vi "Vision_MainUI.vi"(5 "Seq Edit":T2, 7 "Vision Station On?":bool, 8 "error constant":errorcluster, 9 "Real Position Info":T1) -> (0 "error out":errorcluster)   [LabVIEW 2019]
doc: "20160716\nAdd VersionCheck\n\n20160614\nModify Analysis VI : Disable \"Inistialize\" When run it\nModify dll VI : ForCalCalculation memory allocation"
uses:
  Analysis/Controls/Analysis_Type.ctl
  <vilib>/vision/Image Controls.llb/IMAQ Image.ctl
  Controls/UI_Action.ctl
  ROI/Controls/ROI_List_Action.ctl
  Analysis/Controls/Analysis_Setting.ctl
  Process/Controls/Process_Setting.ctl
  Controls/Vision_DataEntry.ctl
  Caliper/Controls/Caliper_Entry_FGV_Action.ctl
  Caliper/Controls/CaliperResult.ctl
  Caliper/Controls/SelectionListEntryPointType.ctl
  Caliper/Controls/SelectionListEntry.ctl
  Caliper/Controls/CaliperType.ctl
  Caliper/Controls/CaliperDataEntry.ctl
  Coordinate/Control/CoordinateAction.ctl
  Coordinate/Control/CoordinateAnalysisSetting.ctl
  Coordinate/Control/CoordinatteEntry.ctl
  Caliper/Controls/AnalysisResultPointsAction.ctl
  Analysis/Controls/Analysis_Result_To_Caliper.ctl
  Controls/Parameter.ctl
  Controls/ParameterData.ctl
  <vilib>/vision/NI_Vision_Development_Module.lvlib
  SubVIs/[Global]iVision_Version.vi
  Controls/iVisionSEQ.ctl
  Coordinate/Control/CoordinateCaliperSetting.ctl
  Analysis/SubVI/[Global]VisionAnalysis_DVR.vi
  Analysis/VisionAnalysisFramework/PackedLibrary/VisionAnalysisFramework.lvlibp/VisionAnalysisFramework/Object/VisionAnalysisFramework.lvclass
  <vilib>/Utility/miscctls.llb/LVRowAndColumnUnsignedTypeDef.ctl
  Analysis/Controls/V_Analysis_Type.ctl
  Ctrl/VisionProcessName.ctl
panel:
  out "Boolean":bool
  in  "CameraName 2":u16(ring) items=["cam0"]
  out "ProjectNameOut":string
  out "Cal Info Image":T3
  in  "Calib":bool
  in  "ConfigROI":bool
  out "RootPath":path
  out "Folder Image Files":path[](array[path])
  in  "SEQ_Name":u16(ring) caption="SEQ Name" items=["v1"]
  in  "Main_Tab":enum32{"Setting", "Result"}(tab)
  in  "Rotate Image Angle":bool
  in  "Angle":dbl format="%#_6f"
  in  "Calibration On":bool
  out "Image Calibration":bool
  in  "Coordinate On":bool
  out "Coordinate Status":bool
  in  "File Path":path
  in  "CycleThruFolder":bool
  in  "GetImage":bool
  in  "SingleRun":bool
  in  "Snap":bool
  in  "ContRun":bool
  out "Vision_Image":T3(plugin-control)
  in  "ROI List":i32[](listbox)
  in  "DeleteROI":bool
  in  "Function_Tab":enum32{"Process", "Analysis", "Caliper"}(tab)
  out "Process Steps":i32(listbox)
  in  "ConfigProcess":bool
  in  "Analysis Function":T4 items=["None", "PatternMatch", "Edge Detection", "Barcode 1D", "Barcode 2D", "Clamp", "Clamp MAX", "Particle", "Histogram", "Straight Edge", "Circle", "Shape Detect", "OCR", "Contour", "ColorMatch"]
  in  "ConfigAnalysis":bool
  in  "CaliperList":i32[](listbox)
  in  "ConfigureCaliper":bool
  in  "RemoveROI":bool
  in  "CreateROI":bool
  in  "CameraName":u16(ring) items=["cam0"]
  in  "Auto Loading ROI Setting":bool
  in  "RemoveFromList":bool caption="Remove"
  in  "AddToOutput":bool caption="Add"
  in  "Output List":i32[](listbox)
  in  "Analysis Result":i32[](listbox)
  out "Item Names":string[][](array[string])
  in  "ExitVisionEditor":bool caption="Exit"
  in  "SaveVisionSEQ":bool caption="Save"
  in  "DeleteVisionSEQ":bool caption="Delete"
  in  "Vision_SEQ_Name":enum16{""}(ring)
  in  "NewVisionSEQ":bool caption="New"
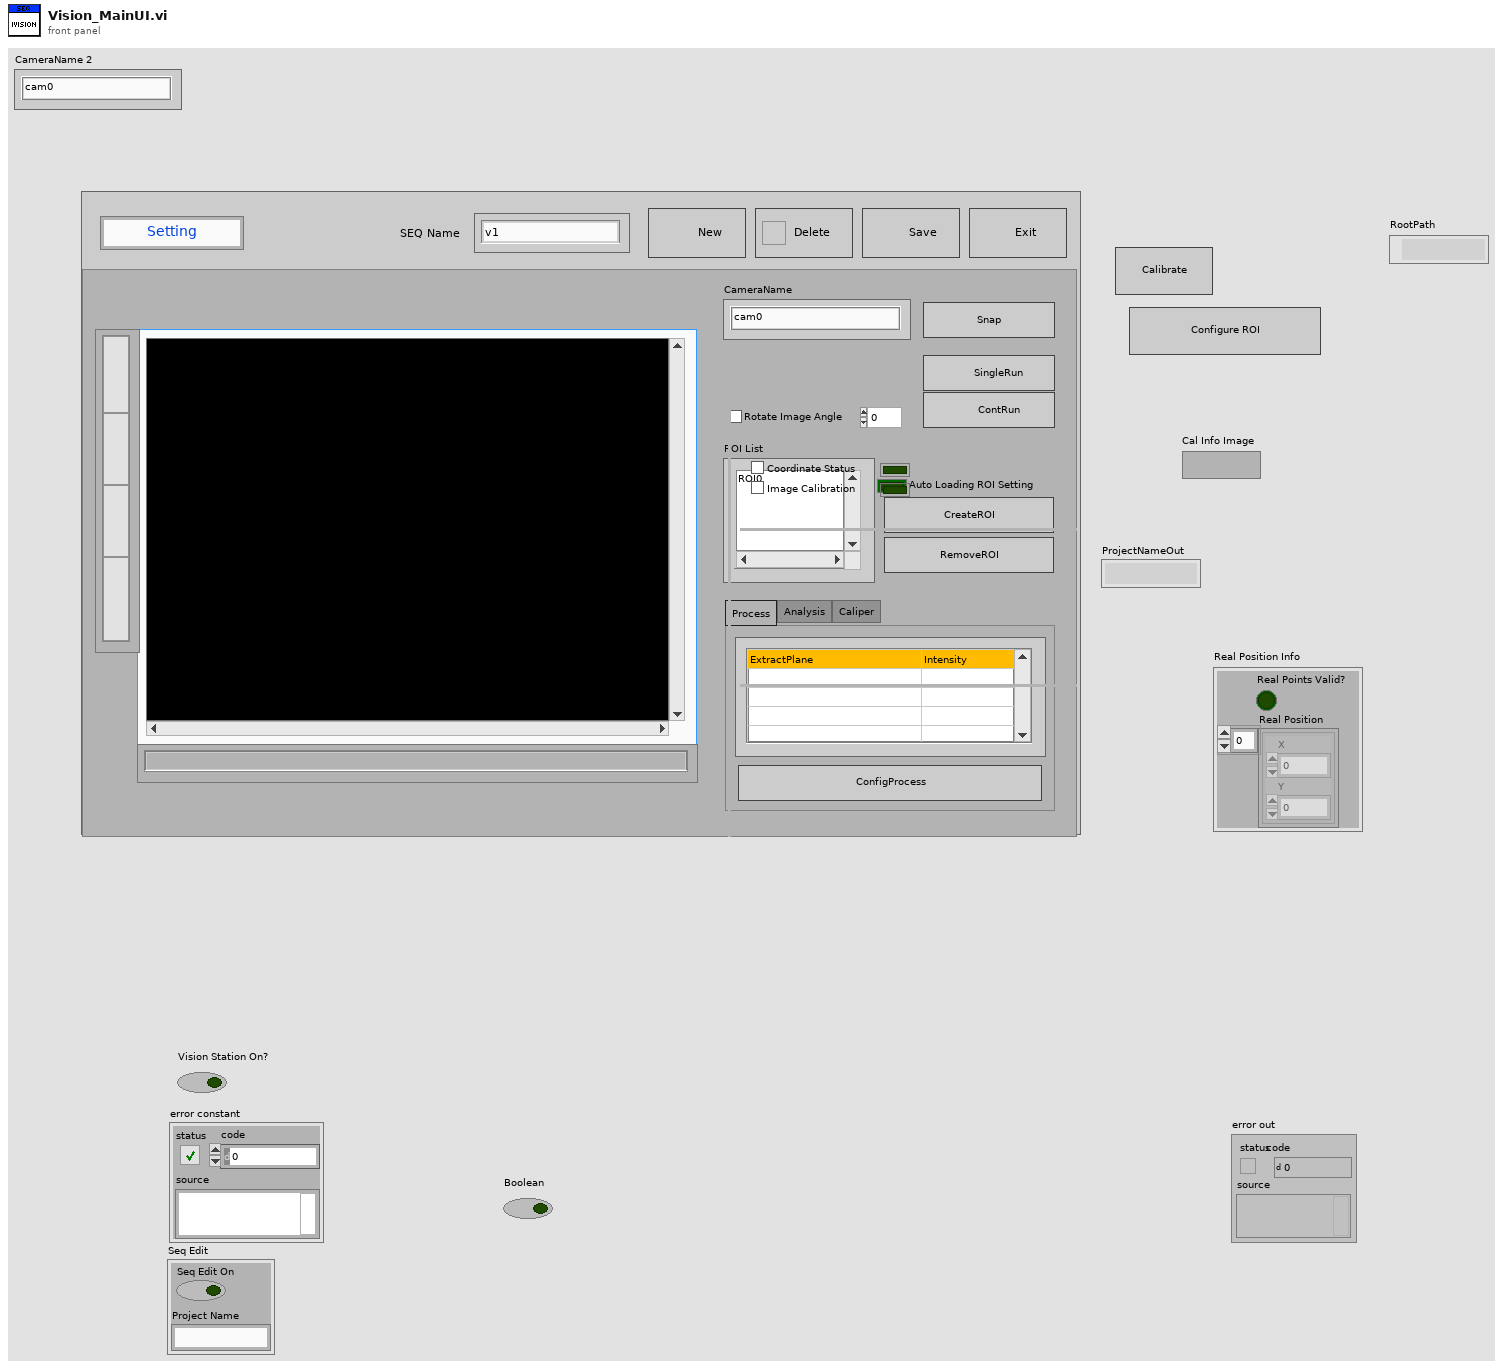
[diagram p1: front panel]
types:
  T1 = cluster{"Real Points Valid?":bool, "Real Position":cluster{"X":dbl, "Y":dbl}[]}
  T2 = cluster{"Seq Edit On":bool, "Project Name":string}
  T3 = typedef "IMAQ Image.ctl" = refnum<image>
  T4 = typedef "Analysis_Type.ctl" = u16
  T5 = typedef "UI_Action.ctl" = enum16{"Init Setting", "Get Root Path", "Exit", "ActivateAllControls", "UpdateROIListbox", "UpdateSelectROIOverlay", "UpdateUIOverlay", "UpdateSelectedOverlay", "ConfigAnalysis", "ConfigProcess", "UpdateExistProjNames", "Init Result Page", "UpdateResultTable", "Init Menu", "Activate Menu", "UpdateProcess", "UpdateAnalysis", "SingleRun", "UpdateSelecedOutput", "ReloadResultTable", "SingleRunWithoutCaliper", "AddNewSeq", "UpdateCaliper", "SaveVisionSEQ", "Init User Parameter", "Cont.Run", "CalRotateImage", "Idle", "UpdateInitStatus", "Initilaize Camera", "Init Read Template", ""}
  T6 = typedef "AnalysisResultPointsAction.ctl" = enum16{"Init", "Add", "Delete", "ReplaceAll", "ReadAll", "Close"}
  T7 = typedef "Caliper_Entry_FGV_Action.ctl" = enum16{"Init", "Close", "Add", "Delete", "ReplaceAll", "ReadAll"}
  T8 = enum8{"Enabled", "Disabled", "Disabled and Grayed Out"}
  T9 = enum16{"Init", "Add", "Remove", "Read All", "Remove All"}
  T10 = typedef "ROI_List_Action.ctl" = enum16{"Init", "Add ROI", "Delete ROI", "Get All ROI", "Get Specific ROI", "Set Analysis Setting", "Set Process Setting", "Replace All Entries", "ROIEntryBackup", "ROIEntryBackupClear", "ROIEntryReturn"}
  T11 = typedef "CoordinateAction.ctl" = enum16{"Initialize", "CoordEntryInput", "CoordEntryOutput", "CoordEntryTemp", "CoordEntryBackup", "CoordEntryReturn"}
  T12 = typedef "Parameter.ctl" = enum16{"Initialize", "Write", "Read", "WriteAll", "Save", "Load"}
  T13 = enum16{"Init", "Grab", "Get All", "Close", "Set Camera"}
  T14 = enum16{"None", "Pattern Match", "Edge Detection", "Barcode 1D", "Barcode 2D", "Clamp", "Clamp MAX", "Particle", "Histogram", "Straight Edge", "Circle", "Shape Dectect", "OCR"}
  T15 = typedef "Analysis_Result_To_Caliper.ctl" = cluster{"PointName":string, "Position_X":dbl, "Position_Y":dbl}
  T16 = enum16{"Init", "Add", "Remove", "Read All", "Remove All", "WriteCriteria"}
  T17 = typedef "CoordinatteEntry.ctl" = cluster{"ProcessSetting":T18[], "Project Name":string, "AnalysisSetting":T20[], "Coord?":bool, "OriginPointInfo":cluster{"Output Original":bool, "Origin Name":string, "Angle":dbl, "Mode":u16, "OriginPoint":cluster{"X":dbl, "Y":dbl}}, "CaliperSetting":T22[], "CoordIndex":i32[]}
  T18 = typedef "Process_Setting.ctl" = cluster{"Enum_PreProcess":T19, "Parameter":string}
  T19 = typedef "VisionProcessName.ctl" = enum16{"*CamParameter*", "CamAttributes", "*Preprocess*", "CG_Brightness", "C_Plane Extraction", "C_Threshold", "G_Lookup Table", "G_Threshold"}
  T20 = typedef "CoordinateAnalysisSetting.ctl" = cluster{"Analysis_Type":enum16{"PatternMatch", "Straight Edge"}, "ROI ":T21, "Parameter":variant, "Step Result":variant, "AnalysisStepName":string, "CoordinateUse":bool}
  T21 = typedef "ROI Descriptor" = cluster{"Global Rectangle":i32[], "Contours":cluster{"ID":enum32{"External", "Internal"}, "Type":u32, "Coordinates":i32[]}[]}
  T22 = typedef "CoordinateCaliperSetting.ctl" = cluster{"Result":variant, "CoordinateUse":bool, "CaliperEntry":T23}
  T23 = typedef "CaliperDataEntry.ctl" = cluster{"CaliperType":T24, "Points":T25[], "Result":T27, "StepName":string}
  T24 = typedef "CaliperType.ctl" = u32
  T25 = typedef "SelectionListEntry.ctl" = cluster{"Type":T26, "Index":i32}
  T26 = typedef "SelectionListEntryPointType.ctl" = enum16{"AnalysisResult", "CaliperResult"}
  T27 = typedef "CaliperResult.ctl" = cluster{"PointInclude?":bool, "Num_Of_Pts":u8, "Position.X":dbl, "Position.Y":dbl, "Angle":dbl, "Distance":dbl, "Area":dbl, "Radius_MAX":dbl, "Radius2_min":dbl, "Dev_Residual":dbl, "P2.X":dbl, "P2.Y":dbl, "StepName":string, "Point ID":u8, "StepError?":bool, "ResultDiff?":bool}
  T28 = typedef "ParameterData.ctl" = cluster{"Rotate Angle":dbl, "Rotate?":bool, "Calibration File Path":string, "Cal?":bool}
  T29 = typedef "Vision_DataEntry.ctl" = cluster{"vROIName":string, "vROIContour":cluster{"Contour Type":u32, "ROI Type":u32, "Points":i32[]}, "ProcessSetting":T18[], "Analysis_Setting":T30}
  T30 = typedef "Analysis_Setting.ctl" = cluster{"PreProcess":T31, "Parameter":string}
  T31 = typedef "V_Analysis_Type.ctl" = enum16{"None", "C_Color Pattern Matching", "G_PatternMatching", "G_ShapeDectect", "G_GeometricMatch", "B_Area Check"}
  T32 = typedef "Image Type" = u32
  T33 = enum32{"invalid app kind", "Development System", "Run Time System", "Student Edition", "Embedded LabVIEW", "Evaluation", "Custom"}
  T34 = typedef "Vision_DataEntry.ctl" = cluster{"vROIName":string, "vROIContour":cluster{"Contour Type":u32, "ROI Type":u32, "Points":i32[]}, "ProcessSetting":T18[], "Analysis_Setting":T35}
  T35 = typedef "Analysis_Setting.ctl" = cluster{"PreProcess":T36, "Parameter":string}
  T36 = typedef "VisionProcessName.ctl" = enum16{"*CamParameter*", "CamAttributes", "*Preprocess*", "CG_Brightness", "C_Plane Extraction", "C_Threshold", "G_Lookup Table", "G_Threshold", "B_Image Inversion", "*Algorithm*", "CG_Histogram", "C_Color Matching", "C_Color Pattern Matching", "G_PatternMatch", "CG_Find Straight Edge", "CG_Adv. Find Straight Edge", "CG_Find Circular Edge", "G_Max Clamp", "G_Clamp (Rake)", "G_Pattern Matching"}
  T37 = typedef "IMAQ Coordinate System" = cluster{"Reference System":cluster{"Origin":cluster{"X":sgl, "Y":sgl}, "Angle (deg)":sgl, "Axis Reference":u32}, "Measurement System":cluster{"Origin":cluster{"X":sgl, "Y":sgl}, "Angle (deg)":sgl, "Axis Reference":u32}}
  T38 = typedef "Analysis_Setting.ctl" = cluster{"PreProcess":T39, "Parameter":string}
  T39 = typedef "V_Analysis_Type.ctl" = enum16{"None", "C_Color Pattern Matching", "G_PatternMatching"}
  T40 = typedef "LVMenuShortCut.ctl" = cluster{"include Shift key?":bool, "include Ctrl key?":bool, "shortcut key":string}
  T41 = cluster{"OutputList":u16[], "Criteria Condition":string[]}
  T42 = typedef "iVisionSEQ.ctl" = cluster{"iVision_Version":string, "iVisionSEQParam":variant}
  T43 = enum16{"open", "replace", "create", "open or create", "replace or create", "replace or create with confirmation"}
  T44 = cluster{"All ROI":cluster{"vROIName":string, "vROIContour":cluster{"Contour Type":u32, "ROI Type":u32, "Points":i32[]}, "ProcessSetting":cluster{"Process_Type":enum16{"None", "ExtractPlane", "BinaryMono", "Operators", "GrayMorphology", "Filters", "Lookup Table", "Particle Filter", "Mask"}, "Parameter":variant}[], "Analysis_Setting":cluster{"Analysis_Type":enum16{"None", "PatternMatch", "Edge Detection", "Barcode 1D", "Barcode 2D", "Clamp", "Clamp MAX", "Particle", "Histogram", "Straight Edge", "Circle", "Shape Dectect", "OCR"}, "RegionContour":cluster{"Contour Type":u32, "ROI Type":u32, "Points":i32[]}, "Parameter":variant}}[], "Output":cluster{"OutputList":u16[], "Criteria Condition":string[]}, string[][], "AllCaliperEntries":cluster{"CaliperType":u32, "Points":cluster{"Type":enum16{"AnalysisResult", "CaliperResult"}, "Index":i32}[], "Result":cluster{"PointInclude?":bool, "Num_Of_Pts":u8, "Position.X":dbl, "Position.Y":dbl, "Angle":dbl, "Distance":dbl, "Area":dbl, "Radius_MAX":dbl, "Radius2_min":dbl, "Dev_Residual":dbl, "P2.X":dbl, "P2.Y":dbl, "StepName":string, "Point ID":u8, "StepError?":bool, "ResultDiff?":bool}, "StepName":string}[], "CoordinatteEntry Output":cluster{"ProcessSetting":cluster{"Process_Type":enum16{"None", "ExtractPlane", "BinaryMono", "Operators", "GrayMorphology", "Filters", "Lookup Table", "Particle Filter", "Mask"}, "Parameter":variant}[], "Project Name":string, "AnalysisSetting":cluster{"Analysis_Type":enum16{"PatternMatch", "Straight Edge"}, "ROI ":T21, "Parameter":variant, "Step Result":variant, "OriginPointInfo":cluster{"Output Original":bool, "Origin Name":string, "Angle":dbl, "Mode":u16, "OriginPoint":cluster{"X":dbl, "Y":dbl}}, "AnalysisStepName":string}[], "Coord?":bool}, "ParameterData Out":cluster{"Rotate Angle":dbl, "Rotate?":bool, "Calibration File Path":string, "Cal?":bool}, "AllCaliperEntries":cluster{"CaliperType":u32, "Points":cluster{"Type":enum16{"AnalysisResult", "CaliperResult"}, "Index":i32}[], "Result":cluster{"PointInclude?":bool, "Num_Of_Pts":u8, "Position.X":dbl, "Position.Y":dbl, "Angle":dbl, "Distance":dbl, "Area":dbl, "Radius_MAX":dbl, "Radius2_min":dbl, "Dev_Residual":dbl, "P2.X":dbl, "P2.Y":dbl, "StepName":string, "Point ID":u8, "StepError?":bool, "ResultDiff?":bool}, "StepName":string}[]}
  T45 = cluster{"All ROI":T29[], "Output":cluster{"OutputList":u16[], "Criteria Condition":string[]}, string[][], "AllCaliperEntries":T23[], "CoordinatteEntry Output":T17, "ParameterData Out":T28, "AllCaliperEntries":T23[]}
  T46 = typedef "LVRowAndColumnUnsignedTypeDef.ctl" = cluster{"Row":u32, "Column":u32}
  T47 = typedef "IMAQdx.ctl" = refnum<k21>
  T48 = cluster{"Global Rectangle":i32[], "Contours":cluster{"Contour Type":u32, "ROI Type":u32, "Points":i32[]}[]}
  T49 = cluster{"Contour Type":u32, "ROI Type":u32, "Points":i32[]}[]
  T50 = cluster{"Contour Type":u32, "ROI Type":u32, "Points":i32[]}
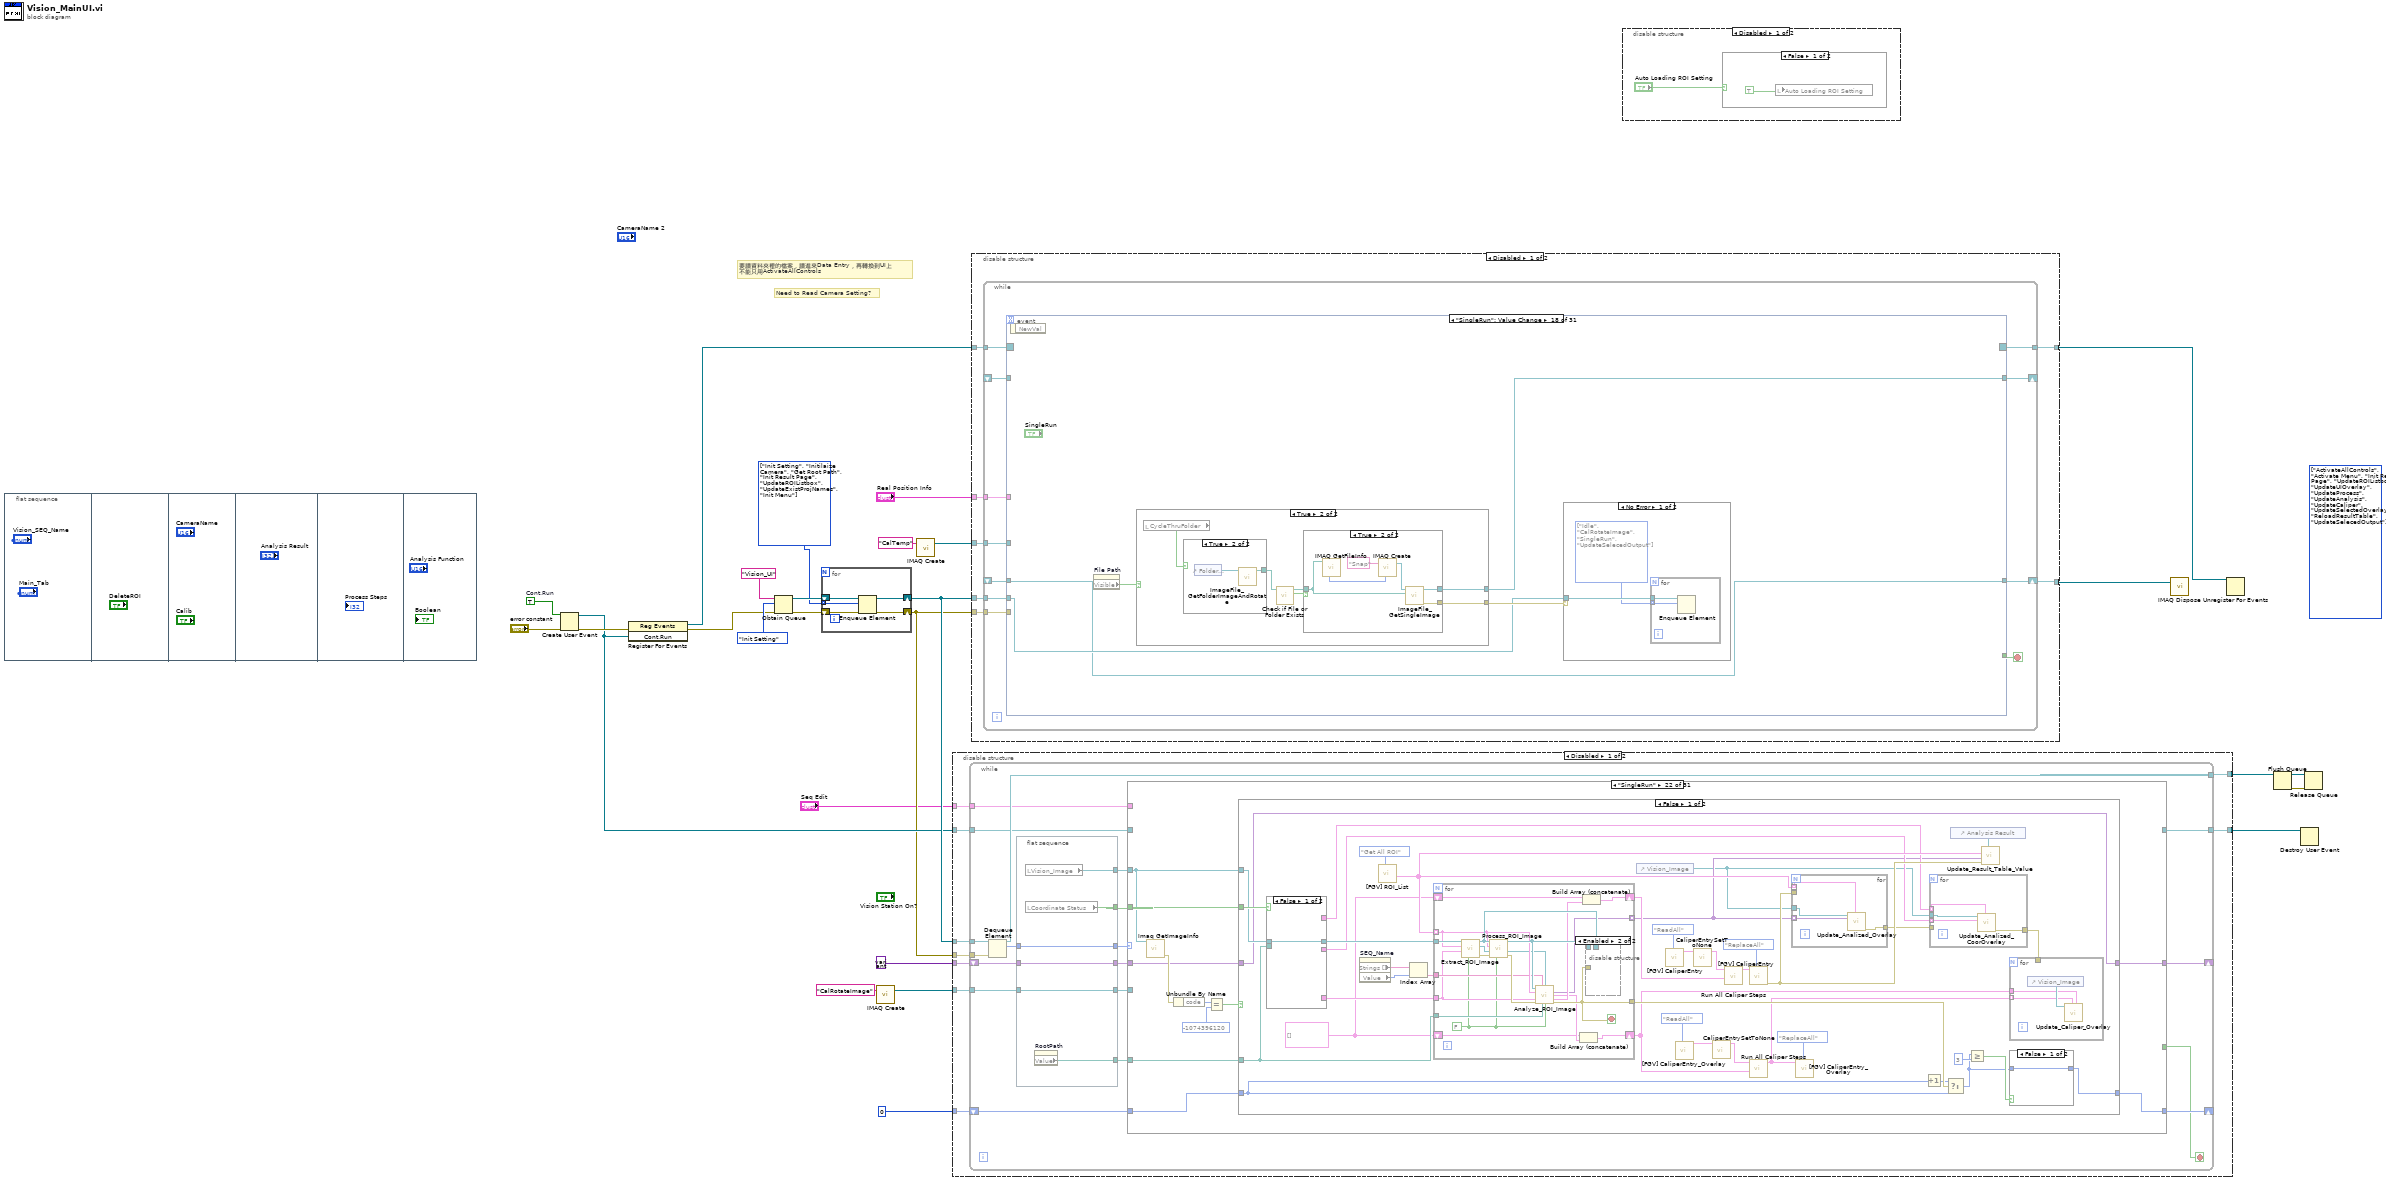
[diagram p0: block diagram]
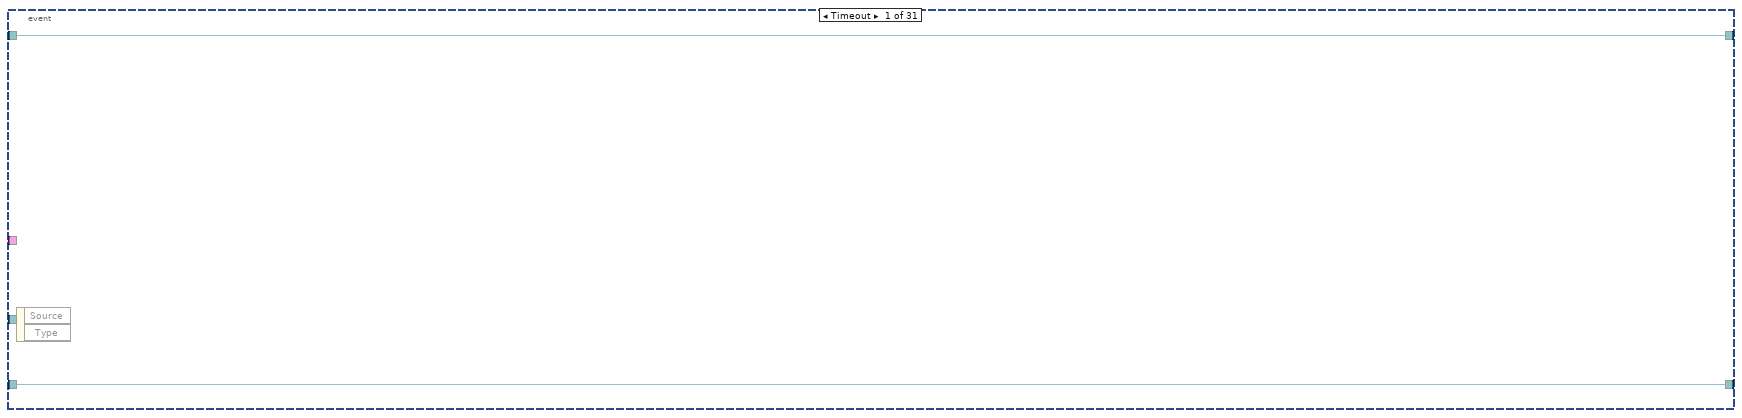
[diagram p2: hidden frame]
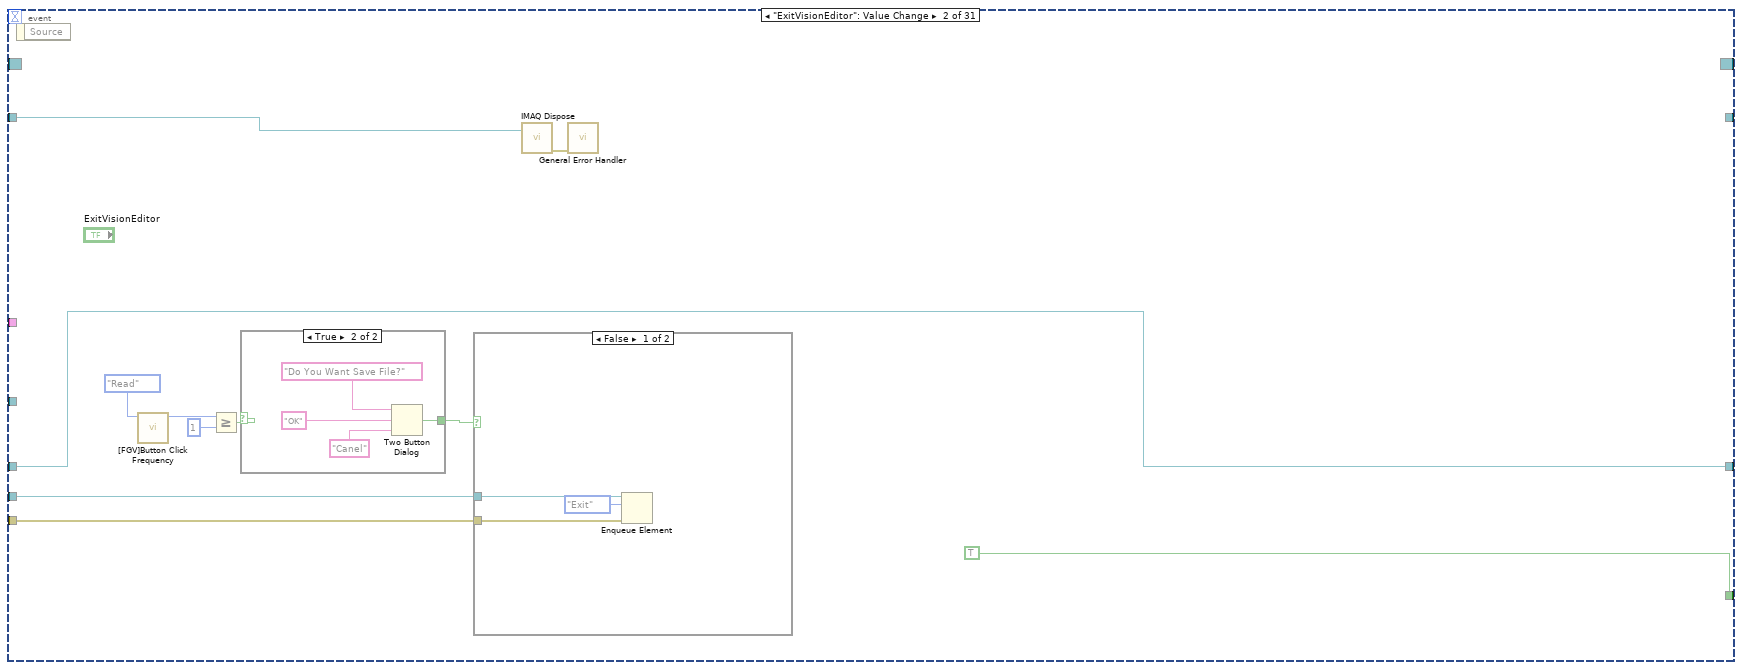
[diagram p3: hidden frame]
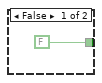
[diagram p4: hidden frame]
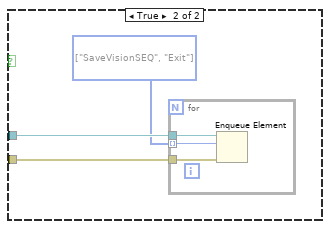
[diagram p5: hidden frame]
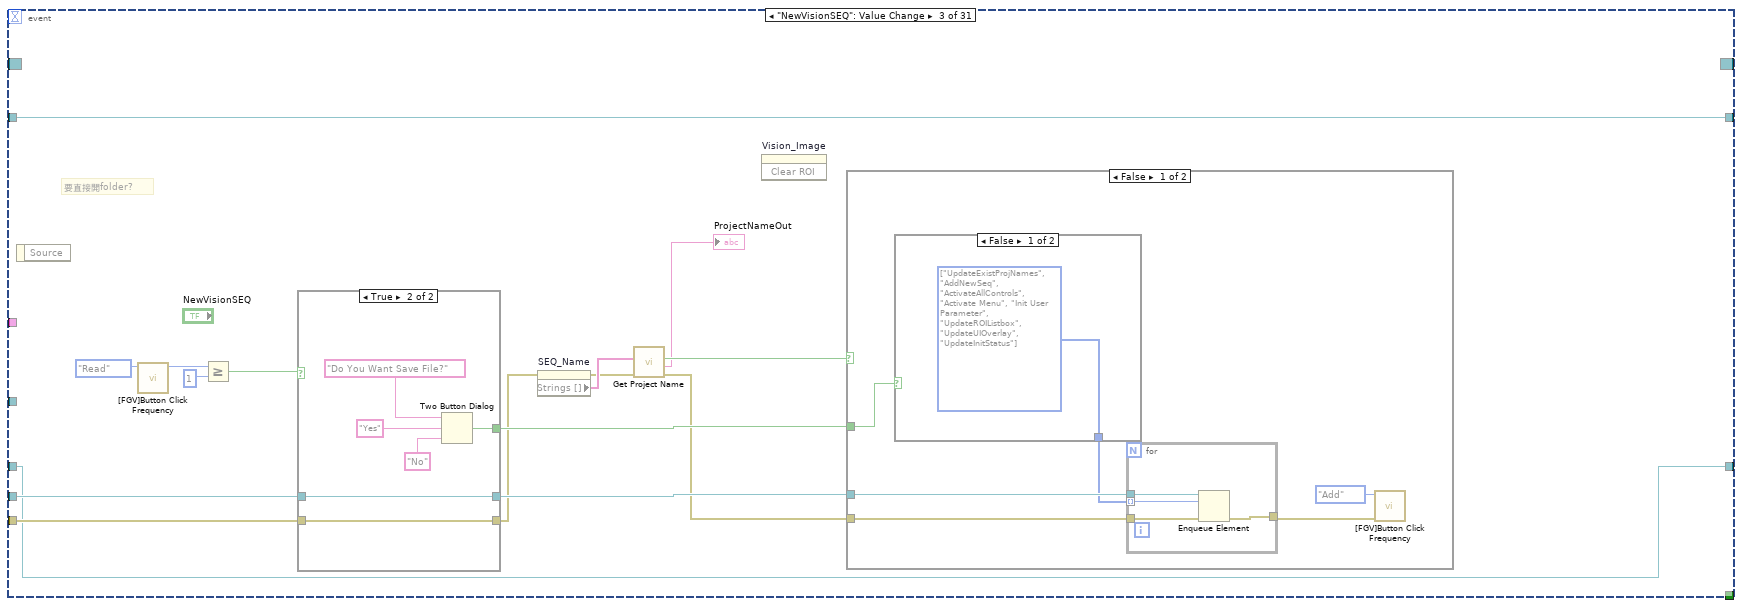
[diagram p6: hidden frame]
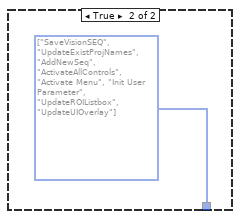
[diagram p7: hidden frame]
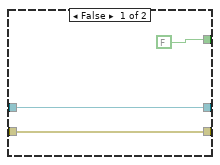
[diagram p9: hidden frame]
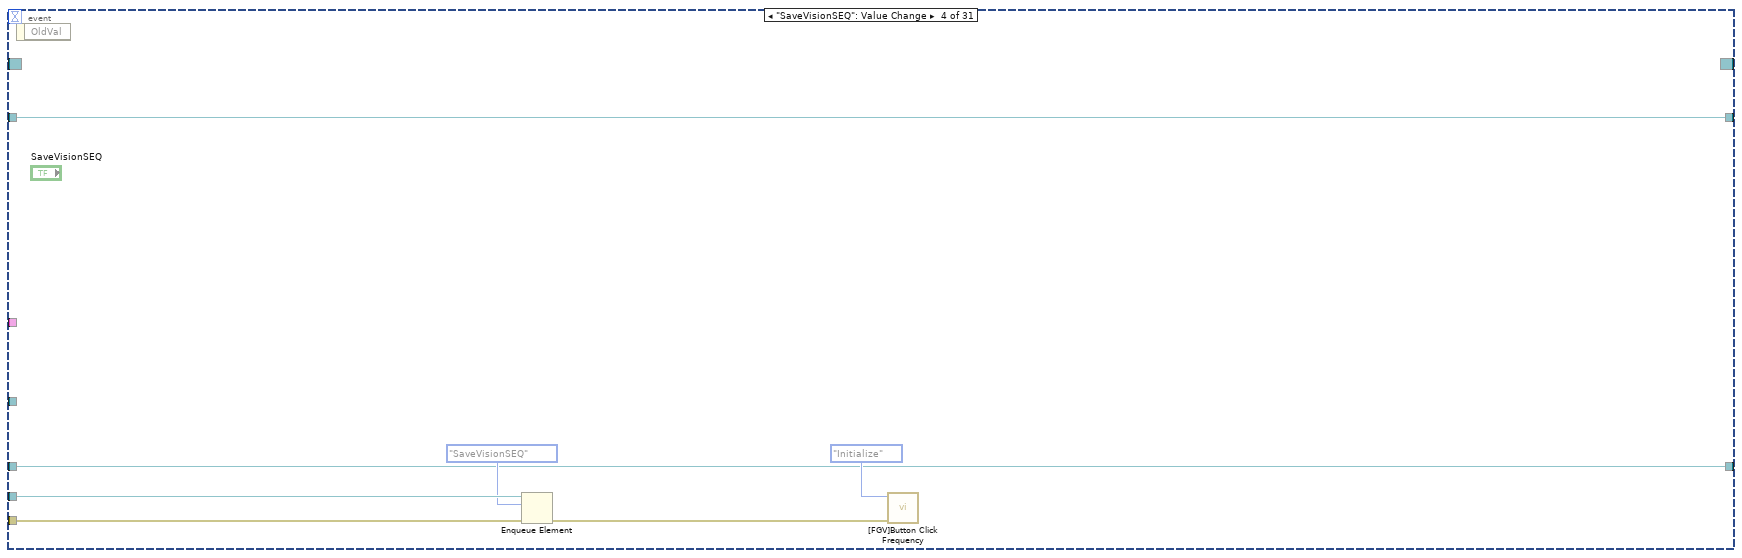
[diagram p10: hidden frame]
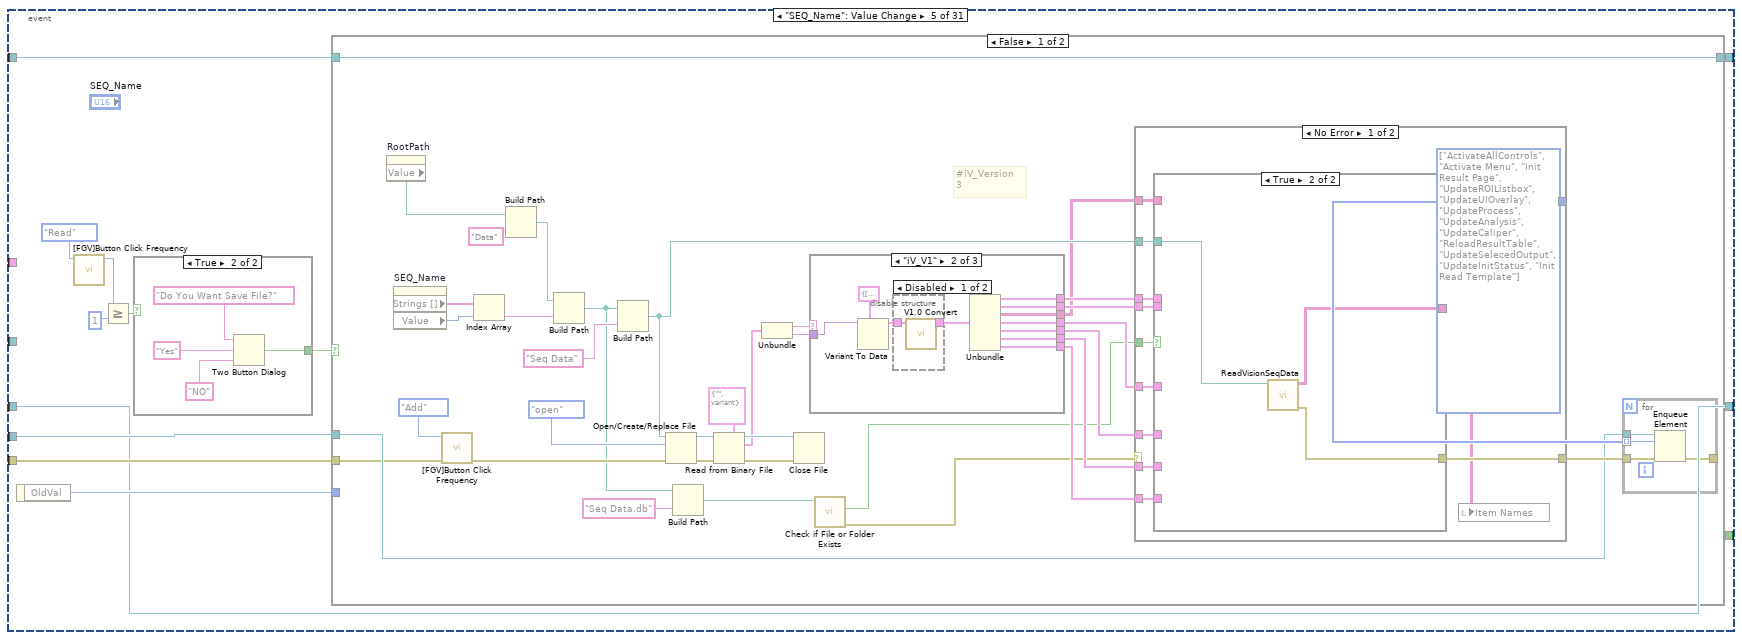
[diagram p11: hidden frame]
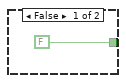
[diagram p12: hidden frame]
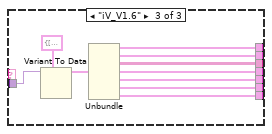
[diagram p15: hidden frame]
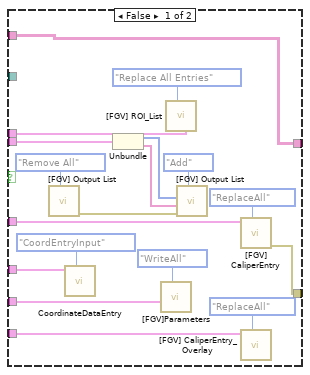
[diagram p16: hidden frame]
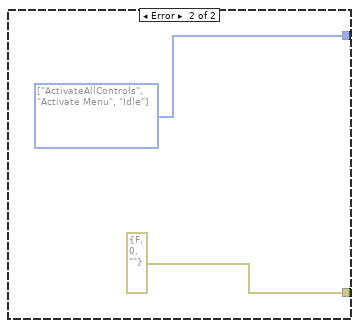
[diagram p17: hidden frame]
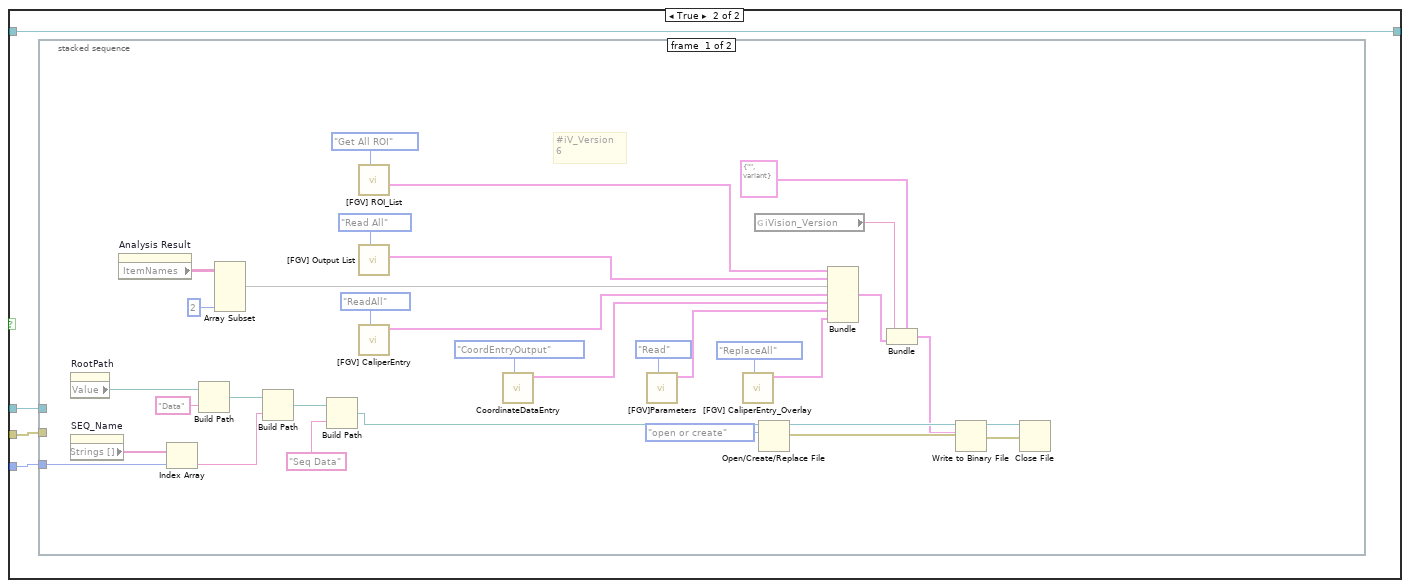
[diagram p18: hidden frame]
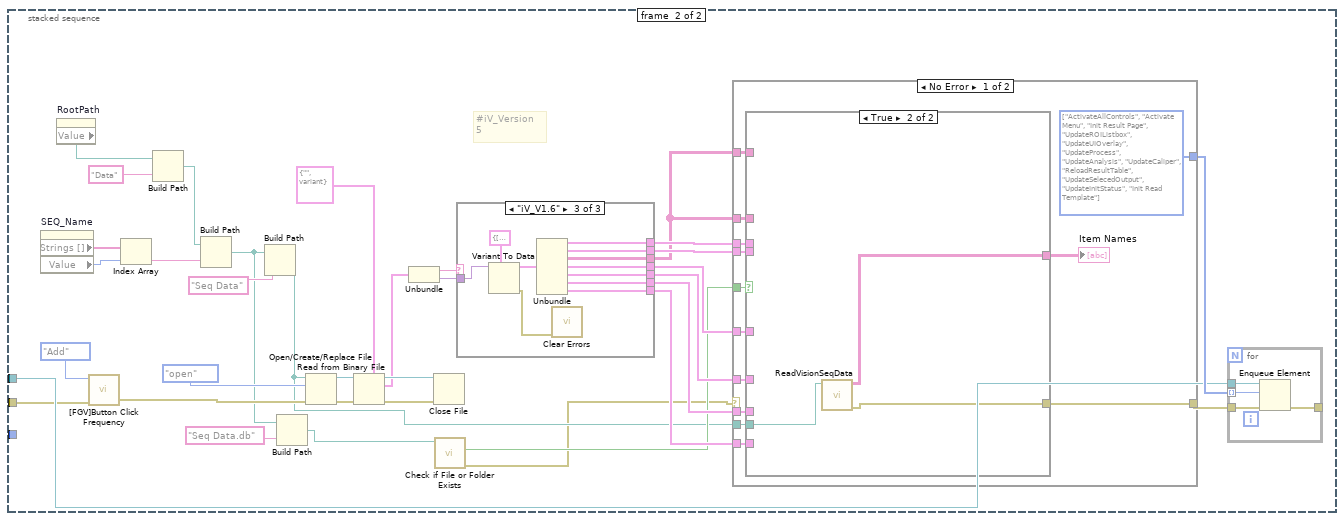
[diagram p19: hidden frame]
diagram:
  w20 = T5[] [enum."Init Setting", enum."Initilaize Camera", enum."Get Root Path", enum."Init Result Page", enum."UpdateROIListbox", enum."UpdateExistProjNames", enum."Init Menu"] items=["Init Setting", "Get Root Path", "Exit", "ActivateAllControls", "UpdateROIListbox", "UpdateSelectROIOverlay", "UpdateUIOverlay", "UpdateSelectedOverlay", "ConfigAnalysis", "ConfigProcess", "UpdateExistProjNames", "Init Result Page", "UpdateResultTable", "Init Menu", "Activate Menu", "UpdateProcess", "UpdateAnalysis", "SingleRun", "UpdateSelecedOutput", "ReloadResultTable", "SingleRunWithoutCaliper", "AddNewSeq", "UpdateCaliper", "SaveVisionSEQ", "Init User Parameter", "Cont.Run", "CalRotateImage", "Idle", "UpdateInitStatus", "Initilaize Camera", "Init Read Template", ""]
  w18 = TRUE  # Cont.Run
  (unwired) T5[] [enum."ActivateAllControls", enum."Activate Menu", enum."Init Result Page", enum."UpdateROIListbox", enum."UpdateUIOverlay", enum."UpdateProcess", enum."UpdateAnalysis", enum."UpdateCaliper", enum."UpdateSelectedOverlay", enum."ReloadResultTable", enum."UpdateSelecedOutput"] items=["Init Setting", "Get Root Path", "Exit", "ActivateAllControls", "UpdateROIListbox", "UpdateSelectROIOverlay", "UpdateUIOverlay", "UpdateSelectedOverlay", "ConfigAnalysis", "ConfigProcess", "UpdateExistProjNames", "Init Result Page", "UpdateResultTable", "Init Menu", "Activate Menu", "UpdateProcess", "UpdateAnalysis", "SingleRun", "UpdateSelecedOutput", "ReloadResultTable", "SingleRunWithoutCaliper", "AddNewSeq", "UpdateCaliper", "SaveVisionSEQ", "Init User Parameter", "Cont.Run", "CalRotateImage", "Idle", "UpdateInitStatus", "Initilaize Camera", "Init Read Template", ""]
  # "要讀資料夾裡的檔案，讀進來Data Entry，再轉換到UI上\n不能只用ActivateAllControls"
  # "Need to Read Camera Setting?"
  n1 = flat-sequence {
    frame #0 {
    }
    frame #1 {
    }
    frame #2 {
    }
    frame #3 {
    }
    frame #4 {
    }
    frame #5 {
    }
  }
  n2 = Create User Event(user event datatype=w18, error in="error constant") -> (user event=w14:refnum<user-event>, error out=w15:errorcluster)
  n3 = register-events(error in=w15, w14) -> (reference out=w17:refnum<event-registration>, error out=w5:errorcluster)  [unwired: 1 in]
  n4 = Obtain Queue(name (unnamed)="Vision_UI", element data type=UI_Action."Init Setting" ("UI_Action"), error in (no error)=w5) -> (queue out=w26:refnum<queue>, error out=w16:errorcluster)  [unwired: 2 in, 1 out]
  n5 = for {
    shift-right: [w30] -> w24
    shift-left: w26 -> [w32]
    shift-right: [w29] -> w4
    shift-left: w16 -> [w31]
    tunnel: w20 -> [w28] mode=indexing
    n6 = Enqueue Element(queue=w32, element=w28, error in (no error)=w31) -> (queue out=w30:refnum<queue>, error out=w29:errorcluster)  [unwired: 1 in, 1 out]
  }
  n7 = call "IMAQ Create"("Image Name"="CalRotateImage") -> ("New Image"=w8:T3)  [unwired: 4 in, 1 out]
  n8 = call "IMAQ Create"("Image Name"="CalTemp") -> ("New Image"=w10:T3)  [unwired: 4 in, 1 out]
  n9 = disable-structure shown="Disabled" {
    disable-tunnel: w24 -> [w41 _]
    disable-tunnel: [w40 _] -> w23
    disable-tunnel: w14 -> [w39 _]
    disable-tunnel: [w38 _] -> w13
    disable-tunnel: w8 -> [w37 _]
    disable-tunnel: 0 -> [w36 _]
    disable-tunnel: variant ("TempAnalysisResult") -> [w35 _]
    disable-tunnel: w4 -> [w34 _]
    disable-tunnel: "Seq Edit" -> [w33 _]
    frame Disabled {
      n10 = while {
        tunnel: w41 -> [w60]
        tunnel: w34 -> [w59]
        tunnel: [w58] -> w40
        tunnel: w39 -> [w55]
        tunnel: [w54] -> w38
        tunnel: w37 -> [w50]
        shift-right: [w47] -> _
        shift-left: w36 -> [w48]
        shift-right: [w46] -> _
        shift-left: w35 -> [w45]
        tunnel: w33 -> [w42]
        stop <- w43 stop-if-true
        n11 = Dequeue Element(queue=w60, error in (no error)=w59) -> (queue out=w58:refnum<queue>, element=w53:T5)  [unwired: 1 in, 2 out]
        n12 = flat-sequence {
          tunnel: [w66] -> w57
          tunnel: [w65] -> w56
          tunnel: [w62] -> w49
          tunnel: [w64] -> w52
          tunnel: w53 -> [w64]
          tunnel: [w63] -> w51
          tunnel: w50 -> [w63]
          tunnel: [w61] -> w44
          tunnel: w45 -> [w61]
          frame #0 {
            n13 = local read "Vision_Image"() -> (w62:T3)
            n14 = local read "Coordinate Status"() -> (w66:bool)
            n15 = property on="RootPath" class="Path"() -> ("Value"=w65:path)  [unwired: 2 in, 2 out]
          }
        }
        n16 = case shown="\"SingleRun\"" w52 {
          tunnel: w57 -> [_ _ _ _ _ _ _ _ _ _ _ w277 w452 _ _ _ _ _ _ _ _ w598 _ w719 _ _ _ _ _ _ _]
          tunnel: w56 -> [_ w116 _ w151 _ _ _ _ _ _ _ w278 w453 _ _ _ _ _ _ _ _ w597 _ w718 _ _ _ _ _ _ _]
          tunnel: w49 -> [_ _ _ _ _ _ _ _ _ _ _ w281 w456 _ _ _ _ _ _ _ _ w592 _ w713 _ _ _ _ _ _ _]
          tunnel: [_ _ _ _ _ TRUE _ _ _ _ _ _ _ _ _ _ _ _ _ _ _ _ _ _ _ _ _ _ _ _ _] -> w43
          tunnel: w55 -> [_ _ _ _ _ w241 _ _ _ _ _ _ _ _ _ _ _ _ _ _ _ _ _ _ _ _ _ _ _ w861 _]
          tunnel: [_ _ _ _ _ w241 _ _ _ _ _ _ _ _ _ _ _ _ _ _ _ _ _ _ _ _ _ _ _ w860 _] -> w54
          tunnel: w51 -> [_ _ _ _ _ _ _ _ _ _ _ _ _ _ _ _ _ _ _ _ _ _ w689 _ _ _ _ _ _ _ _]
          tunnel: w48 -> [w89 w119 w136 w154 w212 w240 w253 w259 w262 w267 w272 w280 w455 w497 w515 w519 w525 w528 w546 w562 w571 w591 w688 w712 w794 w810 w818 w838 w847 w859 w868]
          tunnel: [w89 w119 w136 w154 w212 w240 w253 w259 w262 w267 w272 w280 w455 w497 w515 w519 w525 w528 w546 w562 w571 w590 w688 w712 w794 w810 w818 w838 w847 w859 w868] -> w47
          tunnel: [w87 w115 w135 w153 w211 w239 w252 w258 w261 w266 w271 w279 w454 w496 w514 w518 w524 w527 w545 w561 w570 w589 w687 w711 w793 w809 w817 w837 w846 w858 w867] -> w46
          tunnel: w44 -> [w87 w115 w135 w153 w211 w239 w252 w258 w261 w266 w271 _ w454 w496 w514 w518 w524 w527 w545 w561 w570 w588 w687 w711 w793 w809 w817 w837 w846 w858 w867]
          tunnel: w42 -> [_ _ w134 _ w201 w238 _ _ _ _ _ _ _ _ _ _ _ _ _ _ _ _ _ _ _ _ _ _ _ _ _]
          frame "Init Setting", Default {
            w74 = T4 0 items=["None", "PatternMatch", "Edge Detection", "Barcode 1D", "Barcode 2D", "Clamp", "Clamp MAX", "Particle", "Histogram", "Straight Edge", "Circle", "Shape Detect", "OCR", "Contour", "ColorMatch"] ("Analysis Function")
            # "Load Vision Project Names?"
            # "Load Camera Setting?"
            n17 = control-ref of="Pane"() -> (w106:refnum<vi>)
            n18 = property class="Pane"(reference=w106) -> ("Controls[]"=w105:refnum<vi>[])  [unwired: 1 in, 2 out]
            n19 = for {
              tunnel: w105 -> [w114] mode=indexing
              tunnel: [T8."Enabled" ("Disabled")] -> w101
              tunnel: T8."Disabled and Grayed Out" ("Disabled") -> [w112]
              n20 = property class="Ctl" props=["DisabledEnum", "ClassName", "Label", "Text"](reference=w114, "DisabledEnum"=w112) -> ()  [unwired: 1 in, 4 out]
            }
            n21 = invoke on="Vision_Image" class="ImageControl" method="Reinit To Default"() -> (error out=w75:errorcluster)  [unwired: 3 in, 2 out]
            n22 = invoke on="Vision_Image" class="ImageControl" method="Clear ROI"(error in=w75) -> ()  [unwired: 2 in, 3 out]
            n23 = property on="Analysis Function" class="Ring (strict)"("Value"=w74) -> ()  [unwired: 2 in, 2 out]
            n24 = local write "Main_Tab"(enum32{"Setting", "Result"}."Setting" ("Main_Tab")) -> ()
            n25 = property on="Vision_SEQ_Name" class="Enum (strict)"("DisabledEnum"=w101) -> ()  [unwired: 2 in, 2 out]
            n26 = property on="NewVisionSEQ" class="Bool"("DisabledEnum"=w101) -> ()  [unwired: 2 in, 2 out]
            n27 = property on="ExitVisionEditor" class="Bool"("DisabledEnum"=w101) -> ()  [unwired: 2 in, 2 out]
            n28 = property on="SEQ_Name" class="Ring (strict)"("DisabledEnum"=w101) -> ()  [unwired: 2 in, 2 out]
            n29 = local write "Vision_Image"(T3 refnum ("Vision_Image")) -> ()
            n30 = control-ref of="This VI"() -> (w83:refnum<vi>)
            n31 = property on="ConfigROI" class="Bool"("Visible"=TRUE) -> ()  [unwired: 2 in, 2 out]
            n32 = property class="VI"(reference=w83, "Front Panel.CustomTitle"=TRUE ("Front Panel Window:Custom Title")) -> (reference out=w81:refnum<vi>, "Help.Tag"=w80:string)  [unwired: 1 in, 1 out]
            n33 = property on="Process Steps" class="MCListbox (strict)"("Value"=0 ("Process Steps"), "ItemNames"=string[][] [] ("Item Names")) -> ()  [unwired: 2 in, 2 out]
            n34 = property on="CaliperList" class="LstBox (strict)"("Item Names"=string[] [], "Value"=i32[] [] ("CaliperList")) -> ()  [unwired: 2 in, 2 out]
            n35 = Match Pattern(string=w80, regular expression="_") -> (after substring=w77:string)  [unwired: 1 in, 3 out]
            n36 = global write "[Global]iVision_Version.vi" "iVision_Version"(w80) -> ()
            n37 = call "[FGV] ROI_List.vi"("Action"=ROI_List_Action."Init") -> ()  [unwired: 8 in, 3 out]
            n38 = Concatenate Strings("iVision_" ("string"), w77) -> (w76:string)
            n39 = property class="VI"(reference=w81, "Front Panel.Title"=w76) -> ()  [unwired: 1 in, 2 out]
            n40 = call "[FGV] Analysis_Result_Points.vi"("Action"=AnalysisResultPointsAction."Init") -> ()  [unwired: 9 in, 2 out]
            n41 = call "[FGV] Analysis_Result_Points_Overlay.vi"("Action"=AnalysisResultPointsAction."Init") -> ()  [unwired: 9 in, 2 out]
            n42 = call "[FGV] Analysis_Result_Points_Overlay.vi"("Action"=AnalysisResultPointsAction."Init") -> ()  [unwired: 9 in, 2 out]
            n43 = call "[FGV] CaliperEntry.vi"("Action"=Caliper_Entry_FGV_Action."Init") -> ()  [unwired: 9 in, 2 out]
            n44 = call "[FGV] CaliperEntry_Overlay.vi"("Action"=Caliper_Entry_FGV_Action."Init") -> ()  [unwired: 9 in, 2 out]
            n45 = call "[FGV] Output List.vi"("Action"=T9."Init") -> ()  [unwired: 9 in, 2 out]
            n46 = call "[FGV]Button Click Frequency.vi"("Command"=enum16{"Initialize", "Add", "Read"}."Initialize") -> ()  [unwired: 9 in, 2 out]
            n47 = local read "File Path"() -> (w98:path)
            n48 = call "GetAllPPLFunction_VisionAnalysis.vi"() -> ("PluginRunTime Folder"=w70:path, "AnalysisFunction"=w71:string[])  [unwired: 10 in]
            n49 = call "ImageFile_GetFolderImageFiles.vi"("File Path"=w98) -> ("Folder Image Files"=→"Folder Image Files":path[])  [unwired: 9 in, 1 out]
            n50 = Build Array (concatenate)(string[] ["None", "PatternMatch", "Edge Detection", "Barcode 1D", "Barcode 2D", "Clamp", "Clamp MAX", "Particle", "Histogram", "Straight Edge", "Circle", "Shape Detect", "OCR", "Contour", "ColorMatch"] ("Strings []"), w71) -> (w72:string[])
            n51 = property on="Analysis Function" class="Ring (strict)"("Strings []"=w72) -> ()  [unwired: 2 in, 2 out]
            n52 = for {
              tunnel: w71 -> [w111] mode=indexing
              tunnel: w70 -> [w110]
              tunnel: [w108] -> w69 mode=indexing
              tunnel: refnum<class "VisionAnalysisFramework.lvclass"> refnum ("VisionAnalysisFramework.lvlibp:VisionAnalysisFramework.lvclass") -> [w107]
              n53 = call "GetClassInPPL_VisionAnalysis.vi"("FuncName"=w111, "appended path"=w110) -> ("object"=w109:refnum<class>)  [unwired: 9 in]
              n54 = To More Specific Class(target class=w107, reference=w109) -> (specific class reference=w108:refnum<class "VisionAnalysisFramework.lvclass">)  [unwired: 1 in, 1 out]
            }
            n55 = New Data Value Reference(data value=w69) -> (data value reference=w67:refnum<data-value>)  [unwired: 1 in, 1 out]
            n56 = global write "[Global]VisionAnalysis_DVR.vi" "VisionAnalysis_DVR"(w67) -> ()
          }
          frame "UpdateInitStatus" {
            n57 = call "CoordinateDataEntry.vi"("CoordinateAction"=CoordinateAction."CoordEntryOutput") -> ("CoordinatteEntry Output"=w121:T17)  [unwired: 9 in, 1 out]
            n58 = Unbundle By Name(w121) -> ("Coord?"=w120:bool)
            n59 = local write "Coordinate Status"(w120) -> ()
            n60 = local write "Coordinate On"(w120) -> ()
            n61 = call "[FGV]Parameters.vi"("Parameter"=Parameter."Read") -> ("ParameterData Out"=w125:T28)  [unwired: 9 in, 1 out]
            n62 = Unbundle By Name(w125) -> ("Rotate Angle"=w123:dbl, "Rotate?"=w124:bool, "Cal?"=w118:bool, "Calibration File Path"=w117:string)
            n63 = local write "Angle"(w123) -> ()
            n64 = local write "Rotate Image Angle"(w124) -> ()
            n65 = case shown="True" w118 {
              tunnel: w117 -> [_ w131]
              tunnel: w116 -> [_ w132]
              frame False {
              }
              frame True {
                (unwired) "Snap"
                n66 = Build Path(base path=w132, name or relative path=w131) -> (appended path=w130:path)
                n67 = call "IMAQ Read Image And Vision Info"("File Path"=w130, "Image"="CalTemp" ("string")) -> ("error out"=→"error out":errorcluster, "Image Out"=w129:T3)  [unwired: 7 in, 1 out]
                n68 = local write "Cal Info Image"(w129) -> ()
              }
            }
            n69 = local write "Calibration On"(w118) -> ()
            n70 = local write "Image Calibration"(w118) -> ()
          }
          frame "Initilaize Camera" {
            # "理論上Camera Setting會在Vision之前做好 ?"
            n71 = Unbundle By Name(w134) -> ("Seq Edit On"=w133:bool)
            n72 = case shown="True" w133 {
              tunnel: [w140 _] -> w137
              frame False {
                n73 = call "[FGV] Camera Settings.vi"("Action"=T13."Init") -> ("error out"=w140:errorcluster)  [unwired: 8 in, 2 out]
              }
              frame True {
              }
            }
            n74 = control-ref of="CameraName"() -> (w138:refnum<vi>)
            n75 = call "Camera_SetCameraRing.vi"("error in (no error)"=w137, "Camera Index"=u16 0, "CameraName"=w138) -> ()  [unwired: 8 in, 1 out]
          }
          frame "Init Read Template" {
            # "G:\\¹¤×÷\\Ÿo¹«Ë¾Œ¦Ïó¹²ÓÃ\\jesseFlowCtrl\\Automation_20160802\\Data\\1\\ivision\\data\\1\\CalTemp.png"
            # "CalTemp"
            # "先將所有專案中所有的ROI的Patterm MatchTemplate預讀進來"
            n76 = property on="SEQ_Name" class="Ring (strict)"() -> ("Strings []"=w158:string[], "Value"=w157:u16)  [unwired: 2 in, 2 out]
            n77 = Index Array(array=w158, index=w157) -> (element=w149:string)
            n78 = Build Path(base path=w151, name or relative path="Data") -> (appended path=w160:path)
            n79 = String To Path(string=w149) -> (path=w147:path)
            n80 = Build Path(base path=w160, name or relative path=w149) -> (appended path=w152:path)
            n81 = call "[FGV]Read Template.vi"("Project Name"=w149, "RootPath"=w151) -> ()  [unwired: 9 in, 1 out]
            n82 = Build Path(base path=w147, name or relative path="CalTemp.png" ("string")) -> (appended path=w146:path)
            n83 = call "IMAQ Read Image And Vision Info"("File Path"=w146, "Image"="CalTemp" ("string")) -> ("error out"=w145:errorcluster)  [unwired: 7 in, 2 out]
            n84 = call <vilib>:"Clear Errors.vi"("error in (no error)"=w145) -> ()  [unwired: 5 in, 2 out]
            n85 = call "[FGV] ROI_List.vi"("Action"=ROI_List_Action."Get All ROI") -> ("All ROI"=w162:T29[])  [unwired: 8 in, 2 out]
            n86 = for {
              tunnel: w162 -> [w175] mode=indexing
              tunnel: [w172] -> w156 mode=indexing
              tunnel: [w171] -> w155 mode=indexing
              tunnel: w149 -> [w170]
              tunnel: w152 -> [w169]
              tunnel: [w165] -> w143 mode=indexing
              tunnel: [w164] -> w142 mode=indexing
              i -> [w168]
              n87 = Unbundle By Name(w175) -> ("vROIName"=w167:string, "Analysis_Type"=w166:T4)
              n88 = Concatenate Strings(w170, "_" ("string"), w167) -> (w173:string)
              n89 = case shown="14" w166 {
                tunnel: w173 -> [_ w177 w194]
                tunnel: w169 -> [_ w186 w199]
                tunnel: w168 -> [_ w185 w198]
                tunnel: [T3 refnum ("Template Out") w179 _] -> w172
                tunnel: [_ w178 _] -> w171
                tunnel: [_ _ w192] -> w165
                tunnel: [_ _ w190] -> w164
                frame 0, Default {
                }
                frame 1 {
                  n90 = Number To Decimal String(number=w185) -> (decimal integer string=w184:string)  [unwired: 1 in]
                  n91 = Concatenate Strings(w184, "iVision Template" ("string")) -> (w182:string)
                  n92 = Concatenate Strings(w177, "_PM" ("string")) -> (w178:string)
                  n93 = Build Path(base path=w186, name or relative path=w178) -> (appended path=w181:path)
                  n94 = call "IMAQ Create"("Image Name"=w182) -> ("New Image"=w180:T3)  [unwired: 4 in, 1 out]
                  n95 = call "PatternMatch_ReadTemplate.vi"("template path"=w181, "Template"=w180) -> ("Template Out"=w179:T3)  [unwired: 8 in, 1 out]
                }
                frame 14 {
                  n96 = Number To Decimal String(number=w198) -> (decimal integer string=w197:string)  [unwired: 1 in]
                  n97 = Concatenate Strings(w197, "iVision Template" ("string")) -> (w195:string)
                  n98 = Concatenate Strings(w194, "_CM" ("string")) -> (w190:string)
                  n99 = Build Path(base path=w199, name or relative path=w190) -> (appended path=w189:path)
                  n100 = call "IMAQ GetFileInfo"("File Path"=w189) -> ("Image Type"=w188:T32)  [unwired: 4 in, 6 out]
                  n101 = call "IMAQ Create"("Image Name"=w195, "Image Type"=w188) -> ("New Image"=w193:T3)  [unwired: 3 in, 1 out]
                  n102 = call "IMAQ ReadFile"("File Path"=w189, "Image"=w193) -> ("error out"=w191:errorcluster, "Image Out"=w192:T3)  [unwired: 5 in, 3 out]
                  n103 = call <vilib>:"Clear Errors.vi"("error in (no error)"=w191) -> ()  [unwired: 5 in, 2 out]
                }
              }
            }
            n104 = call "[FGV] Template.vi"("Image Name Array"=w155, "Image Array"=w156, "Command"=enum16{"Initialize", "Save", "Read"}."Save") -> ()  [unwired: 6 in, 3 out]
            n105 = call "[FGV]ColorMatch_Template.vi"("CMTemplateCommand"="Save", "Image Name Array"=w142, "Image Array"=w143) -> ()  [unwired: 6 in, 3 out]
          }
          frame "Get Root Path" {
            n106 = local read "Vision Station On?"() -> (w210:bool)
            n107 = Unbundle By Name(w201) -> ("Seq Edit On"=w209:bool, "Project Name"=w205:string)
            n108 = Build Array(w210, w209) -> (w208:bool[])
            n109 = Search 1D Array(1D array=w208, element=TRUE) -> (index of element=w206:i32)  [unwired: 1 in]
            n110 = case shown="1" w206 {
              tunnel: [w213 w223 w231] -> w204
              tunnel: w205 -> [_ _ w234]
              tunnel: [w213 _ w226] -> w202
              frame -1, Default {
                n111 = control-ref of="This Application"() -> (w214:refnum<vi>)
                n112 = property class="App"(reference=w214) -> (reference out=w216:refnum<vi>, "App.Kind"=w215:T33)  [unwired: 1 in, 1 out]
                n113 = Close Reference(reference=w216) -> ()  [unwired: 1 in, 1 out]
                n114 = Current VI's Path() -> (path=w217:path)
                n115 = case shown="\"Run Time System\"" w215 {
                  tunnel: w217 -> [w219 w222]
                  tunnel: [w218 w220] -> w213
                  frame "Development System", Default {
                    n116 = Strip Path(path=w219) -> (stripped path=w218:path)  [unwired: 1 out]
                  }
                  frame "Run Time System" {
                    n117 = Strip Path(path=w222) -> (stripped path=w221:path)  [unwired: 1 out]
                    n118 = Strip Path(path=w221) -> (stripped path=w220:path)  [unwired: 1 out]
                  }
                }
              }
              frame 0 {
                n119 = call <vilib>:"Application Directory.vi"() -> ("Application Directory"=w225:path)
                n120 = Build Path(base path=w225, name or relative path="Data\\IVision") -> (appended path=w223:path)
              }
              frame 1 {
                n121 = call <vilib>:"Application Directory.vi"() -> ("Application Directory"=w230:path)
                n122 = Build Path(base path=w230, name or relative path="Data") -> (appended path=w235:path)
                n123 = Build Path(base path=w230, name or relative path="Vision") -> (appended path=w228:path)
                n124 = Build Path(base path=w235, name or relative path=w234) -> (appended path=w233:path)
                n125 = Build Path(base path=w228, name or relative path="iVision") -> (appended path=w226:path)
                n126 = Build Path(base path=w233, name or relative path="ivision") -> (appended path=w231:path)
              }
            }
            "RootPath" <- w204
            n127 = call "Get Dll Path.vi"("Action"=enum16{"WriteDllRoot", "GetDllRoot"}."WriteDllRoot", "Root"=w202) -> ()  [unwired: 9 in, 1 out]
          }
          frame "Exit" {
            w243 = u16 0
            w244 = string[] [] ("Strings []")
            n128 = control-ref of="Pane"() -> (w246:refnum<vi>)
            n129 = property class="Pane"(reference=w246) -> ("Controls[]"=w245:refnum<vi>[])  [unwired: 1 in, 2 out]
            n130 = Unbundle By Name(w238) -> ("Seq Edit On"=w237:bool)
            n131 = for {
              tunnel: w245 -> [w251] mode=indexing
              n132 = property class="Ctl"(reference=w251, "DisabledEnum"=T8."Enabled" ("Disabled")) -> ()  [unwired: 1 in, 2 out]
            }
            n133 = case shown="False" w237 {
              frame False {
                n134 = call "[FGV] Camera Settings.vi"("Action"=T13."Close") -> ()  [unwired: 8 in, 3 out]
              }
              frame True {
              }
            }
            n135 = disable-structure shown="Enabled" {
              disable-tunnel: w244 -> [w249 _]
              disable-tunnel: w243 -> [w248 _]
              frame Enabled {
                n136 = property on="CameraName" class="Ring (strict)"("Value"=w248, "Strings []"=w249) -> ()  [unwired: 2 in, 2 out]
              }
              frame Disabled {
              }
            }
            n137 = property on="SEQ_Name" class="Ring (strict)"("Value"=w243, "Strings []"=w244) -> ()  [unwired: 2 in, 2 out]
          }
          frame "ActivateAllControls" {
            n138 = control-ref of="Pane"() -> (w255:refnum<vi>)
            n139 = property class="Pane"(reference=w255) -> ("Controls[]"=w254:refnum<vi>[])  [unwired: 1 in, 2 out]
            n140 = for {
              tunnel: w254 -> [w257] mode=indexing
              n141 = property class="Ctl"(reference=w257, "DisabledEnum"=T8."Enabled" ("Disabled")) -> ()  [unwired: 1 in, 2 out]
            }
          }
          frame "UpdateROIListbox" {
            n142 = control-ref of="ROI List"() -> (w260:refnum<vi>)
            n143 = call "Update_UI_ROI_List.vi"("LstBox Refnum"=w260) -> ()  [unwired: 10 in, 1 out]
          }
          frame "UpdateUIOverlay" {
            n144 = control-ref of="Vision_Image"() -> (w263:refnum<vi>)
            n145 = call "Update_UI_Overlay.vi"("Image Refnum"=w263) -> ()  [unwired: 10 in, 1 out]
          }
          frame "UpdateSelectROIOverlay" {
            n146 = property on="ROI List" class="LstBox (strict)"() -> ("Value"=w265:i32[])  [unwired: 2 in, 2 out]
            n147 = control-ref of="Vision_Image"() -> (w268:refnum<vi>)
            n148 = Index Array(array=w265) -> (element=w264:i32)  [unwired: 1 in]
            n149 = call "UpdateSelectROIOverlay.vi"("Index"=w264, "Image Refnum"=w268) -> ()  [unwired: 9 in, 1 out]
          }
          frame "UpdateSelectedOverlay" {
            n150 = control-ref of="Vision_Image"() -> (w270:refnum<vi>)
            n151 = control-ref of="ROI List"() -> (w269:refnum<vi>)
            n152 = disable-structure shown="Enabled" {
              disable-tunnel: w270 -> [w274 w276]
              disable-tunnel: w269 -> [w273 w275]
              frame Disabled {
                n153 = call "Update_UI_SelectedOverlay.vi"("LstBox Refnum"=w273, "Image Refnum"=w274) -> ()  [unwired: 9 in, 1 out]
              }
              frame Enabled {
                n154 = call "Update_UI_SelectedOverlayChangeToROI.vi"("LstBox Refnum"=w275, "Image Refnum"=w276) -> ()  [unwired: 9 in, 1 out]
              }
            }
          }
          frame "ConfigAnalysis" {
            # "沒有影像輸入的錯誤碼"
            n155 = call "Imaq GetImageInfo"("Image"=w281) -> ("error out"=w282:errorcluster)  [unwired: 3 in, 7 out]
            n156 = Unbundle By Name(w282) -> ("code"=w285:i32)
            n157 = Equal?(x=w285, y=-1074396120) -> (x = y?=w283:bool)
            n158 = case shown="False" w283 {
              tunnel: w281 -> [w298 _]
              tunnel: w282 -> [_ _]
              tunnel: [w288 _] -> w279
              tunnel: w278 -> [w286 _]
              tunnel: w277 -> [w287 _]
              frame False {
                # "1 or 0"
                n159 = property on="ROI List" class="LstBox (strict)"() -> ("Value"=w291:i32[])  [unwired: 2 in, 2 out]
                n160 = property on="Analysis Function" class="Ring (strict)"() -> ("Value"=w297:T4)  [unwired: 2 in, 2 out]
                n161 = control-ref of="ROI List"() -> (w293:refnum<vi>)
                n162 = call "IMAQ Clear Overlay"("Image"=w298) -> ("Image Out"=w289:T3)  [unwired: 9 in, 1 out]
                n163 = Index Array(array=w291) -> (element=w295:i32)  [unwired: 1 in]
                n164 = call "[FGV] ROI_List.vi"("Action"=ROI_List_Action."Get Specific ROI", "ROIs_Index"=w291) -> ("ROI Entry"=w290:T34)  [unwired: 7 in, 2 out]
                n165 = Greater Or Equal?(x=w295, y=0) -> (x >= y?=w294:bool)
                n166 = case shown="True" w294 {
                  tunnel: w297 -> [_ w324]
                  tunnel: w289 -> [_ w304]
                  tunnel: w293 -> [_ w323]
                  tunnel: w291 -> [_ w313]
                  tunnel: w290 -> [_ w311]
                  tunnel: w286 -> [_ w300]
                  tunnel: [_ w308] -> w288
                  tunnel: w286 -> [_ _]
                  tunnel: w287 -> [_ w302]
                  frame False {
                    n167 = One Button Dialog(message="Please Create & Select  1 ROI For Analysis~!!!") -> ()  [unwired: 1 in, 1 out]
                  }
                  frame True {
                    w309 = FALSE ("CreatDllImage")
                    n168 = case shown="True" w302 {
                      tunnel: w304 -> [w325 w329]
                      tunnel: [w325 w328] -> w303
                      tunnel: [_ w327] -> w301
                      tunnel: w300 -> [_ w326]
                      frame False {
                      }
                      frame True {
                        n169 = call "RunCoordinateSys.vi"("RootPath"=w326, "Image In"=w329) -> ("Coordinate System Out"=w327:T37, "Vision_Image Out"=w328:T3)  [unwired: 5 in, 3 out]
                      }
                    }
                    n170 = call "Extract_ROI_Image.vi"("CreatDllImage"=w309, "Coordinate System Out"=w301, "ROI Entry"=w311, "ImageIn"=w303) -> ("error out"=w322:errorcluster, "ForCalCalculaton Out"=w307:T3, "ExtractedOriginalImage"=w305:T3)  [unwired: 5 in]
                    n171 = call "Process_ROI_Image.vi"("CreatDllImage"=w309, "error in (no error)"=w322, "ForCalCalculaton In"=w307, "ROI Entry"=w311, "ImageIn"=w305) -> ("error out"=w321:errorcluster, "ForCalCalculaton Out"=w306:T3, "ExtractedProcessedImage"=w320:T3)  [unwired: 4 in]
                    n172 = property on="SEQ_Name" class="Ring (strict)"() -> ("Strings []"=w316:string[], "Value"=w315:u16)  [unwired: 2 in, 2 out]
                    n173 = Unbundle By Name(w311) -> ("Analysis_Setting"=w312:T35)
                    n174 = Index Array(array=w316, index=w315) -> (element=w314:string)
                    n175 = case shown="1" w324 {
                      tunnel: w320 -> [_ w345 w353 w361 w369 w377 w384 w395 w403 w411 w419 w425 w426 w439 w449 _]
                      tunnel: w323 -> [_ w344 w348 w356 w364 w371 w379 w389 w396 w410 w415 _ w433 _ w448 _]
                      tunnel: w321 -> [_ w343 w352 w360 w368 w376 w385 w394 w402 w404 w412 w420 w428 w438 w447 _]
                      tunnel: [_ w342 w351 w359 w367 w375 w382 w393 w399 w405 w416 w424 w431 w434 w446 _] -> w317
                      tunnel: [_ w341 w350 w357 w366 w374 w381 w392 w400 w406 w417 w423 w427 w435 w445 _] -> w319
                      tunnel: [_ w340 w349 w358 w365 w373 w383 w391 w401 w407 w418 w422 w432 w436 w444 _] -> w318
                      tunnel: w314 -> [_ w339 w347 w355 w362 w370 w378 w388 w398 w408 w414 _ w430 _ w443 _]
                      tunnel: w312 -> [_ w338 w346 w354 w363 w372 w380 w390 w397 w409 w413 w421 w429 w437 w442 _]
                      tunnel: w300 -> [_ w337 _ _ _ _ _ _ _ _ _ _ _ _ w441 _]
                      tunnel: [_ _ _ _ _ _ _ w387 _ _ _ _ _ _ _ _] -> w308
                      tunnel: w306 -> [_ _ _ _ _ _ _ w386 _ _ _ _ _ _ _ _]
                      frame 0 {
                      }
                      frame 1 {
                        n176 = call "PatternMatch_Setting_UI.vi"("RootPath"=w337, "Type"="iVision", "Analysis_Setting In"=w338, "error in (no error)"=w343, "ProjectName"=w339, "LstBox Refnum"=w344, "Vision_Image In"=w345) -> ("error out"=w342:errorcluster, "Cancel?"=w341:bool, "Analysis_Setting"=w340:T38)  [unwired: 2 in]
                      }
                      frame 2 {
                        n177 = call "EdgeDetection_Setting_UI.vi"("Analysis_Setting IN"=w346, "error in (no error)"=w352, "ProjectName"=w347, "ROI List IN"=w348, "Vision_Image"=w353) -> ("error out"=w351:errorcluster, "Cancel?"=w350:bool, "Analysis_Setting"=w349:T35)  [unwired: 4 in]
                      }
                      frame 3 {
                        n178 = call "Barcode 1D_Setting_UI.vi"("Analysis_Setting IN"=w354, "error in (no error)"=w360, "ProjectName"=w355, "ROI List IN"=w356, "Vision_Image"=w361) -> ("error out"=w359:errorcluster, "Cancel?"=w357:bool, "Analysis_Setting"=w358:T35)  [unwired: 4 in]
                      }
                      frame 4 {
                        n179 = call "Barcode 2D_Setting_UI.vi"("Analysis_Setting In"=w363, "error in (no error)"=w368, "ProjectName"=w362, "ROI List IN"=w364, "Vision_Image"=w369) -> ("error out"=w367:errorcluster, "Cancel?"=w366:bool, "Analysis_Setting"=w365:T35)  [unwired: 4 in]
                      }
                      frame 5 {
                        n180 = call "Clamp_Setting_UI.vi"("Analysis_Setting IN"=w372, "error in (no error)"=w376, "ProjectName"=w370, "ROI List IN"=w371, "Vision_Image"=w377) -> ("error out"=w375:errorcluster, "Cancel?"=w374:bool, "Analysis_Setting"=w373:T35)  [unwired: 4 in]
                      }
                      frame 6 {
                        n181 = call "Clamp MAX_Setting_UI.vi"("Analysis_Setting IN"=w380, "error in (no error)"=w385, "ProjectName"=w378, "ROI List IN"=w379, "Vision_Image"=w384) -> ("error out"=w382:errorcluster, "Cancel?"=w381:bool, "Analysis_Setting"=w383:T35)  [unwired: 4 in]
                      }
                      frame 7 {
                        n182 = call "Particles_Setting_UI.vi"("ForCalCalculaton In"=w386, "Analysis_Setting IN"=w390, "error in (no error)"=w394, "ProjectName"=w388, "ROI List IN"=w389, "Vision_Image"=w395) -> ("error out"=w393:errorcluster, "Cancel?"=w392:bool, "TempAnalysisResult"=w387:variant, "Analysis_Setting"=w391:T35)  [unwired: 2 in]
                      }
                      frame 8 {
                        n183 = call "Histogram_Setting_UI.vi"("Analysis_Setting IN"=w397, "error in (no error)"=w402, "ProjectName"=w398, "ROI List IN"=w396, "Vision_Image"=w403) -> ("error out"=w399:errorcluster, "Cancel?"=w400:bool, "Analysis_Setting"=w401:T35)  [unwired: 4 in]
                      }
                      frame 9 {
                        n184 = call "Find Straight Edge.vi"("Analysis_Setting IN"=w409, "error in (no error)"=w404, "ProjectName"=w408, "ROI List IN"=w410, "Vision_Image"=w411) -> ("error out"=w405:errorcluster, "Cancel?"=w406:bool, "Analysis_Setting"=w407:T35)  [unwired: 4 in]
                      }
                      frame 10 {
                        n185 = call "Circle_Setting_UI.vi"("Analysis_Setting IN"=w413, "error in (no error)"=w412, "ProjectName"=w414, "ROI List IN"=w415, "Vision_Image"=w419) -> ("error out"=w416:errorcluster, "Cancel?"=w417:bool, "Analysis_Setting"=w418:T35)  [unwired: 4 in]
                      }
                      frame 11 {
                        n186 = call "ShapeDetect_Setting_UI.vi"(6:w421, "error in (no error)"=w420, "Vision_Image"=w425) -> ("error out"=w424:errorcluster, "Cancel?"=w423:bool, "ParameterOut"=w422:string)  [unwired: 6 in]
                      }
                      frame 12 {
                        n187 = call "OCR_Setting_UI.vi"("Analysis_Setting"=w429, "error in (no error)"=w428, "ProjectName"=w430, "LstBox Refnum"=w433, "Vision_Image"=w426) -> ("error out"=w431:errorcluster, "Cancel?"=w427:bool, "output cluster"=w432:T35)  [unwired: 4 in]
                      }
                      frame 13 {
                        n188 = call "Contour_Setting_UI.vi"("Analysis_Setting In"=w437, "error in (no error)"=w438, "Vision_Image"=w439) -> ("error out"=w434:errorcluster, "Cancel?"=w435:bool, "Analysis_Setting Out"=w436:T35)  [unwired: 6 in]
                      }
                      frame 14 {
                        n189 = call "ColorMatch_Setting_UI.vi"("Vision_Image In"=w449, 3:"iVision" ("Type"), "List ROI 2"=w448, "ProjectName"=w443, "error in (no error)"=w447, "Parameter"=w442, "RootPath"=w441) -> ("Analysis_Setting"=w444:string, "Cancel?"=w445:bool, "error out"=w446:errorcluster)  [unwired: 4 in, 2 out]
                      }
                      frame 15, Default {
                      }
                    }
                    n190 = case shown="False" w319 {
                      tunnel: w318 -> [w333 _]
                      tunnel: w317 -> [w331 w335]
                      tunnel: w313 -> [w332 _]
                      tunnel: [w330 w335] -> w310
                      frame False {
                        n191 = call "[FGV] ROI_List.vi"("Action"=ROI_List_Action."Set Analysis Setting", "error in (no error)"=w331, "ROIs_Index"=w332, "Analysis_Setting"=w333) -> ("error out"=w330:errorcluster)  [unwired: 5 in, 2 out]
                      }
                      frame True {
                      }
                    }
                    n192 = call "IMAQ Dispose"("Image"=w320, "error in (no error)"=w310) -> ()  [unwired: 4 in, 1 out]
                    n193 = call "IMAQ Dispose"("Image"=w305, "error in (no error)"=w310) -> ()  [unwired: 4 in, 1 out]
                  }
                }
              }
              frame True {
                n194 = One Button Dialog(message="Not an image.", button name ("OK")="Stop") -> ()  [unwired: 1 out]
              }
            }
          }
          frame "ConfigProcess" {
            # "沒有影像輸入的錯誤碼"
            n195 = call "Imaq GetImageInfo"("Image"=w456) -> ("error out"=w458:errorcluster)  [unwired: 3 in, 7 out]
            n196 = Unbundle By Name(w458) -> ("code"=w460:i32)
            n197 = Equal?(x=w460, y=-1074396120) -> (x = y?=w457:bool)
            n198 = case shown="False" w457 {
              tunnel: w456 -> [w464 _]
              tunnel: w453 -> [w463 _]
              tunnel: w452 -> [w462 _]
              frame False {
                # "1 or 0"
                n199 = call "IMAQ Clear Overlay"("Image"=w464) -> ("Image Out"=w461:T3)  [unwired: 9 in, 1 out]
                n200 = property on="ROI List" class="LstBox (strict)"() -> ("Value"=w466:i32[])  [unwired: 2 in, 2 out]
                n201 = Index Array(array=w466) -> (element=w469:i32)  [unwired: 1 in]
                n202 = control-ref of="ROI List"() -> ()  [unwired: 1 out]
                n203 = Greater Or Equal?(x=w469, y=0) -> (x >= y?=w468:bool)
                n204 = call "[FGV] ROI_List.vi"("Action"=ROI_List_Action."Get Specific ROI", "ROIs_Index"=w466) -> ("ROI Entry"=w465:T34)  [unwired: 7 in, 2 out]
                n205 = case shown="True" w468 {
                  tunnel: w461 -> [_ w474]
                  tunnel: w466 -> [_ w482]
                  tunnel: w465 -> [_ w479]
                  tunnel: w463 -> [_ w476]
                  tunnel: w462 -> [_ w475]
                  frame False {
                    n206 = One Button Dialog(message="Please Create & Select  1 ROI For Analysis~!!!") -> ()  [unwired: 1 in, 1 out]
                  }
                  frame True {
                    # "點選每個ROI,  各自的參數沒辦法各自己顯示"
                    n207 = case shown="True" w475 {
                      tunnel: w474 -> [w485 w489]
                      tunnel: [w485 w488] -> w472
                      tunnel: [_ w487] -> w473
                      tunnel: w476 -> [_ w486]
                      frame False {
                      }
                      frame True {
                        n208 = call "RunCoordinateSys.vi"("RootPath"=w486, "Image In"=w489) -> ("Coordinate System Out"=w487:T37, "Vision_Image Out"=w488:T3)  [unwired: 5 in, 3 out]
                      }
                    }
                    n209 = Unbundle By Name(w479) -> ("ProcessSetting"=w478:T18[])
                    n210 = call "Extract_ROI_Image.vi"("CreatDllImage"=FALSE, "Coordinate System Out"=w473, "ROI Entry"=w479, "ImageIn"=w472) -> ("ExtractedOriginalImage"=w484:T3)  [unwired: 5 in, 2 out]
                    n211 = control-ref of="Process Steps"() -> (w480:refnum<vi>)
                    n212 = call "Process_Setting_UI.vi"("ProcessSettingIn"=w478, "Vision_Image_In"=w484) -> ("Cancel?"=w481:bool, "ProcessSettingOut"=w483:T18[])  [unwired: 8 in]
                    n213 = case shown="False" w481 {
                      tunnel: w483 -> [w490 _]
                      tunnel: w482 -> [w492 _]
                      tunnel: w480 -> [w491 _]
                      frame False {
                        n214 = call "Show_Process_Steps.vi"("ProcessSettingIn"=w490, "ProcessSteps"=w491) -> ()  [unwired: 9 in, 1 out]
                        n215 = call "[FGV] ROI_List.vi"("ProcessSetting"=w490, "Action"=ROI_List_Action."Set Process Setting", "ROIs_Index"=w492) -> ()  [unwired: 6 in, 3 out]
                      }
                      frame True {
                      }
                    }
                  }
                }
              }
              frame True {
                n216 = One Button Dialog(message="Not an image.", button name ("OK")="Stop") -> ()  [unwired: 1 out]
              }
            }
          }
          frame "UpdateExistProjNames" {
            # "在執行UpdateExistProjNames之前，\n一定要先執行 Get Root Path"
            n217 = property on="RootPath" class="Path"() -> ("Value"=w498:path)  [unwired: 2 in, 2 out]
            n218 = Build Path(base path=w498, name or relative path="Data") -> (appended path=w503:path)
            n219 = call <vilib>:"Check if File or Folder Exists.vi"("path"=w503) -> ("file or folder exists?"=w502:bool, "dup path"=w501:path)  [unwired: 8 in, 1 out]
            n220 = case shown="False" w502 {
              tunnel: w501 -> [_ w513]
              tunnel: [w506 w511] -> w500
              tunnel: [FALSE w508] -> _
              frame False {
                # "要Create Foldedr?"
                n221 = Build Array("") -> (w506:string[])
              }
              frame True {
                n222 = List Folder(path=w513) -> (folder names=w510:string[])  [unwired: 3 in, 3 out]
                n223 = Array Size(array=w510) -> (size(s)=w509:i32)
                n224 = Build Array (concatenate)("", w510) -> (w511:string[])
                n225 = Not Equal To 0?(x=w509) -> (x != 0?=w508:bool)
              }
            }
            n226 = property on="SEQ_Name" class="Ring (strict)"("Strings []"=w500, "Value"=u16 0) -> ()  [unwired: 2 in, 2 out]
          }
          frame "Init Result Page" {
            w516 = i32[] [] ("Analysis Result")
            w517 = string[][] [] ("Item Names")
            n227 = property on="Analysis Result" class="MCListbox (strict)"("Value"=w516, "ItemNames"=w517) -> ()  [unwired: 2 in, 2 out]
            n228 = property on="Output List" class="MCListbox (strict)"("Value"=w516, "ItemNames"=w517) -> ()  [unwired: 2 in, 2 out]
          }
          frame "UpdateResultTable" {
            # "#AnalysisResult \nitem names"
            n229 = property on="SEQ_Name" class="Ring (strict)"() -> ("Strings []"=w523:string[], "Value"=w522:u16)  [unwired: 2 in, 2 out]
            n230 = Index Array(array=w523, index=w522) -> (element=w521:string)
            n231 = control-ref of="Analysis Result"() -> (w520:refnum<vi>)
            n232 = call "Update_Result_Table.vi"("MCListbox Refnum"=w520, "TempAnalysisResult"=w518, "ProjectName"=w521) -> ()  [unwired: 9 in]
          }
          frame "ReloadResultTable" {
            n233 = property on="Item Names" class="Arr (strict)"() -> ("Value"=w526:string[][])  [unwired: 2 in, 2 out]
            n234 = property on="Analysis Result" class="MCListbox (strict)"("ItemNames"=w526) -> ()  [unwired: 2 in, 2 out]
          }
          frame "Init Menu" {
            w530 = FALSE ("checked")
            w529 = TRUE ("checked")
            w535 = "Image File Mode" ("message")
            w540 = "Camera Mode" ("message")
            n235 = Current VI's Menubar() -> (w542:refnum<k9>)
            n236 = Get Menu Item Info(7:w540, 11:w542) -> (2:w539:string, 3:w541:refnum<k9>, 6:w538:T40)  [unwired: 1 in, 4 out]
            n237 = Set Menu Item Info(4:w538, 6:w529, 7:w540, 9:FALSE ("enabled"), 10:w539, 11:w541) -> (3:w533:refnum<k9>)  [unwired: 1 in, 1 out]
            n238 = Get Menu Item Info(7:w535, 11:w533) -> (2:w536:string, 3:w534:refnum<k9>, 6:w537:T40)  [unwired: 1 in, 4 out]
            n239 = disable-structure shown="Enabled" {
              disable-tunnel: w529 -> [w543 w544]
              frame Enabled {
                n240 = property on="CameraName" class="Ring (strict)"("Visible"=w543) -> ()  [unwired: 2 in, 2 out]
              }
              frame Disabled {
              }
            }
            n241 = property on="Snap" class="Bool"("Visible"=w529) -> ()  [unwired: 2 in, 2 out]
            n242 = Set Menu Item Info(4:w537, 6:w530, 7:w535, 9:FALSE ("enabled"), 10:w536, 11:w534) -> ()  [unwired: 1 in, 2 out]
            n243 = property on="CycleThruFolder" class="Bool (strict)"("Visible"=w530) -> ()  [unwired: 2 in, 2 out]
            n244 = property on="GetImage" class="Bool"("Visible"=w530) -> ()  [unwired: 2 in, 2 out]
            n245 = property on="File Path" class="Path"("Visible"=w530) -> ()  [unwired: 2 in, 2 out]
          }
          frame "Activate Menu" {
            w553 = "Image File Mode" ("message")
            w558 = "Camera Mode" ("message")
            n246 = Current VI's Menubar() -> (w560:refnum<k9>)
            n247 = Get Menu Item Info(7:w558, 11:w560) -> (2:w557:string, 3:w559:refnum<k9>, 4:w548:bool, 6:w556:T40)  [unwired: 1 in, 3 out]
            n248 = Set Menu Item Info(4:w556, 6:w548, 7:w558, 9:TRUE ("enabled"), 10:w557, 11:w559) -> (3:w551:refnum<k9>)  [unwired: 1 in, 1 out]
            n249 = Get Menu Item Info(7:w553, 11:w551) -> (2:w554:string, 3:w552:refnum<k9>, 4:w547:bool, 6:w555:T40)  [unwired: 1 in, 3 out]
            n250 = Set Menu Item Info(4:w555, 6:w547, 7:w553, 9:TRUE ("enabled"), 10:w554, 11:w552) -> ()  [unwired: 1 in, 2 out]
          }
          frame "UpdateProcess" {
            n251 = property on="ROI List" class="LstBox (strict)"() -> ("Value"=w566:i32[])  [unwired: 2 in, 2 out]
            n252 = call "[FGV] ROI_List.vi"("Action"=ROI_List_Action."Get Specific ROI", "ROIs_Index"=w566) -> ("ROI Entry"=w564:T34)  [unwired: 7 in, 2 out]
            n253 = Unbundle By Name(w564) -> ("ProcessSetting"=w563:T18[])
            n254 = control-ref of="Process Steps"() -> (w565:refnum<vi>)
            n255 = call "Show_Process_Steps.vi"("ProcessSettingIn"=w563, "ProcessSteps"=w565) -> ()  [unwired: 9 in, 1 out]
          }
          frame "UpdateAnalysis" {
            n256 = property on="ROI List" class="LstBox (strict)"() -> ("Value"=w572:i32[])  [unwired: 2 in, 2 out]
            n257 = call "[FGV] ROI_List.vi"("Action"=ROI_List_Action."Get Specific ROI", "ROIs_Index"=w572) -> ("ROI Entry"=w569:T34)  [unwired: 7 in, 2 out]
            n258 = Unbundle By Name(w569) -> ("Analysis_Type"=w568:T4)
            n259 = disable-structure shown="Disabled" {
              disable-tunnel: w568 -> [w574 _]
              frame Disabled {
                n260 = case shown="3" w574 {
                  tunnel: [T14."None" ("Analysis Function") T14."Pattern Match" ("Analysis Function") T14."Edge Detection" ("Analysis Function") T14."Barcode 1D" ("Analysis Function") T14."Barcode 2D" ("Analysis Function") T14."Clamp" ("Analysis Function") T14."Clamp MAX" ("Analysis Function") T14."Particle" ("Analysis Function") T14."Histogram" ("Analysis Function") T14."Straight Edge" ("Analysis Function") T14."Circle" ("Analysis Function") T14."Shape Dectect" ("Analysis Function") T14."OCR" ("Analysis Function")] -> _
                  frame 0, Default {
                  }
                  frame 1 {
                  }
                  frame 2 {
                  }
                  frame 3 {
                  }
                  frame 4 {
                  }
                  frame 5 {
                  }
                  frame 6 {
                  }
                  frame 7 {
                  }
                  frame 8 {
                  }
                  frame 9 {
                  }
                  frame 10 {
                  }
                  frame 11 {
                  }
                  frame 12 {
                  }
                }
              }
              frame Enabled {
              }
            }
            n261 = property on="Analysis Function" class="Ring (strict)"("Value"=w568) -> ()  [unwired: 2 in, 2 out]
          }
          frame "SingleRun" {
            n262 = call "Imaq GetImageInfo"("Image"=w592) -> ("error out"=w594:errorcluster)  [unwired: 3 in, 7 out]
            n263 = Unbundle By Name(w594) -> ("code"=w596:i32)
            n264 = Equal?(x=w596, y=-1074396120) -> (x = y?=w593:bool)
            n265 = case shown="False" w593 {
              tunnel: w598 -> [w629 _]
              tunnel: w597 -> [w626 _]
              tunnel: w592 -> [w624 _]
              tunnel: w591 -> [w619 w683]
              tunnel: [w615 w683] -> w590
              tunnel: [w613 w682] -> w589
              tunnel: w588 -> [w613 w682]
              frame False {
                w610 = T15[] [] ("Analysis_Point_Result")
                n266 = case shown="False" w629 {
                  tunnel: w624 -> [w652 w658]
                  tunnel: [w652 w657] -> w628
                  tunnel: [_ w656] -> w627
                  tunnel: w626 -> [_ w655]
                  tunnel: [_ w654] -> w603
                  tunnel: [_ w653] -> w604
                  frame False {
                  }
                  frame True {
                    n267 = call "RunCoordinateSys.vi"("RootPath"=w655, "Image In"=w658) -> ("AnalysisSetting"=w654:T20[], "Coordinate System Out"=w656:T37, "Vision_Image Out"=w657:T3, "Main Out"=w653:T29[])  [unwired: 5 in, 1 out]
                  }
                }
                n268 = property on="SEQ_Name" class="Ring (strict)"() -> ("Strings []"=w636:string[], "Value"=w625:u16)  [unwired: 2 in, 2 out]
                n269 = call "[FGV] ROI_List.vi"("Action"=ROI_List_Action."Get All ROI") -> ("All ROI"=w623:T29[])  [unwired: 8 in, 2 out]
                n270 = Index Array(array=w636, index=w625) -> (element=w635:string)
                n271 = for {
                  tunnel: w623 -> [w673] mode=indexing
                  tunnel: w628 -> [w677]
                  tunnel: [w665] -> w600 mode=indexing
                  tunnel: w626 -> [w672]
                  tunnel: w635 -> [w671]
                  shift-right: [w668] -> w621
                  shift-left: w610 -> [w670]
                  tunnel: w627 -> [w667]
                  tunnel: [w666] -> w620
                  shift-right: [w659] -> w605
                  shift-left: w610 -> [w660]
                  stop <- w666 stop-if-true
                  w662 = FALSE ("CreatDllImage")
                  n272 = call "Extract_ROI_Image.vi"("CreatDllImage"=w662, "Coordinate System Out"=w667, "ROI Entry"=w673, "ImageIn"=w677) -> ("error out"=w678:errorcluster, "ForCalCalculaton Out"=w664:T3, "ExtractedOriginalImage"=w675:T3)  [unwired: 5 in]
                  n273 = call "Process_ROI_Image.vi"("CreatDllImage"=w662, "error in (no error)"=w678, "ForCalCalculaton In"=w664, "ROI Entry"=w673, "ImageIn"=w675) -> ("error out"=w676:errorcluster, "ForCalCalculaton Out"=w663:T3, "ExtractedProcessedImage"=w674:T3)  [unwired: 4 in]
                  n274 = call "Analyze_ROI_Image.vi"("ImageIn"=w674, "ProjectName"=w671, "ForCalCalculaton In"=w663, "ROI Entry"=w673, "Coordinate System In"=w667, "error in (no error)"=w676, "RootPath"=w672, "CreatDllImage"=w662) -> ("AnalysisResult"=w665:variant, "Analysis_Point_Result Out Overlay"=w661:T15[], "Analysis_Point_Result"=w669:T15[], "error out"=w666:errorcluster)  [unwired: 3 in, 1 out]
                  n275 = Build Array (concatenate)(w660, w661) -> (w659:T15[])
                  n276 = Build Array (concatenate)(w670, w669) -> (w668:T15[])
                  n277 = disable-structure shown="Enabled" {
                    disable-tunnel: w675 -> [w681 _]
                    disable-tunnel: w666 -> [w680 _]
                    disable-tunnel: w674 -> [w679 _]
                    frame Disabled {
                      n278 = call "IMAQ Dispose"("Image"=w681, "error in (no error)"=w680) -> ()  [unwired: 4 in, 1 out]
                      n279 = call "IMAQ Dispose"("Image"=w679, "error in (no error)"=w680) -> ()  [unwired: 4 in, 1 out]
                    }
                    frame Enabled {
                    }
                  }
                }
                n280 = control-ref of="Vision_Image"() -> (w599:refnum<vi>)
                n281 = call "[FGV] CaliperEntry.vi"("Action"=Caliper_Entry_FGV_Action."ReadAll") -> ("AllCaliperEntries"=w632:T23[])  [unwired: 9 in, 1 out]
                n282 = call "[FGV] CaliperEntry_Overlay.vi"("Action"=Caliper_Entry_FGV_Action."ReadAll") -> ("AllCaliperEntries"=w608:T23[])  [unwired: 9 in, 1 out]
                n283 = call "CaliperEntrySetToNone.vi"("CaliperEntryList"=w632) -> ("CaliperEntryOut"=w634:T23[])  [unwired: 9 in, 1 out]
                n284 = call "CaliperEntrySetToNone.vi"("CaliperEntryList"=w608) -> ("CaliperEntryOut"=w609:T23[])  [unwired: 9 in, 1 out]
                n285 = call "Run All Caliper Steps.vi"("Analysis_Point_Result"=w621, "CaliperEntryList"=w634) -> ("CaliperEntryOut"=w622:T23[])  [unwired: 9 in]
                n286 = call "[FGV] CaliperEntry.vi"("Action"=Caliper_Entry_FGV_Action."ReplaceAll", "CaliperEntriesIn"=w622) -> ("error out"=w630:errorcluster)  [unwired: 8 in, 1 out]
                n287 = call "Run All Caliper Steps.vi"("Analysis_Point_Result"=w605, "CaliperEntryList"=w609) -> ("CaliperEntryOut"=w606:T23[])  [unwired: 9 in]
                n288 = for {
                  tunnel: w623 -> [w648] mode=indexing
                  tunnel: w600 -> [w647] mode=indexing
                  tunnel: [w646] -> w602
                  tunnel: w630 -> [_]
                  tunnel: w599 -> [w645]
                  n289 = call "Update_Analized_Overlay.vi"("ROI Entry"=w648, "AnalysisResult"=w647, "Image Refnum"=w645) -> ("error out"=w646:errorcluster)  [unwired: 7 in, 1 out]
                }
                n290 = call "[FGV] CaliperEntry_Overlay.vi"("Action"=Caliper_Entry_FGV_Action."ReplaceAll", "CaliperEntriesIn"=w606) -> ()  [unwired: 8 in, 2 out]
                n291 = Increment(x=w619) -> (x+1=w618:i32)
                n292 = for {
                  tunnel: w604 -> [w641] mode=indexing
                  tunnel: w603 -> [w640] mode=indexing
                  tunnel: w602 -> [_]
                  tunnel: [w639] -> w601
                  tunnel: w599 -> [w638]
                  n293 = call "Update_Analized_CoorOverlay.vi"("ROI Entry"=w641, "AnalysisResult"=w640, "Image Refnum"=w638) -> ("error out"=w639:errorcluster)  [unwired: 7 in, 1 out]
                }
                n294 = Select(t=w618, s=w620, f=w619) -> (s? t:f=w614:i32)
                n295 = control-ref of="Analysis Result"() -> (w612:refnum<vi>)
                n296 = Greater Or Equal?(x=w614, y=3) -> (x >= y?=w616:bool)
                n297 = call "Update_Result_Table_Value.vi"("MCListbox Refnum"=w612, "error in (no error)"=w630, "AnalysisResults"=w600, "All ROI"=w623) -> ()  [unwired: 7 in, 1 out]
                n298 = for {
                  tunnel: w606 -> [w643] mode=indexing
                  tunnel: w605 -> [w642]
                  tunnel: w601 -> [_]
                  n299 = control-ref of="Vision_Image"() -> (w644:refnum<vi>)
                  n300 = call "Update_Caliper_Overlay.vi"("Analysis_Point_Result"=w642, "CaliperEntry"=w643, "Image Refnum"=w644) -> ()  [unwired: 9 in]
                }
                n301 = case shown="False" w616 {
                  tunnel: [w649 0 ("y")] -> w615
                  tunnel: w614 -> [w649 _]
                  frame False {
                  }
                  frame True {
                    n302 = property on="ContRun" class="Bool (strict)"("Val(Sgnl)"=FALSE ("ContRun")) -> ()  [unwired: 2 in, 2 out]
                  }
                }
              }
              frame True {
                n303 = One Button Dialog(message="Not an image.", button name ("OK")="Stop") -> ()  [unwired: 1 out]
              }
            }
          }
          frame "CalRotateImage" {
            # "記得在做dll時要另外建立一個calibration記憶體空間"
            n304 = local read "Image Calibration"() -> (w690:bool)
            n305 = local read "Cal Info Image"() -> (w693:T3)
            n306 = call "SetCalInfo.vi"("CalRotateImage"=w689, "CalibrationTemplate"=w693, "Image Calibration"=w690, "Vision_Image"="Snap") -> ("Not an Image?"=w691:bool, "ImageRef Out"=w692:T3)  [unwired: 6 in]
            n307 = case shown="False" w691 {
              frame False {
              }
              frame True {
                n308 = One Button Dialog(message="Not an image.", button name ("OK")="Stop") -> ()  [unwired: 1 out]
              }
            }
            n309 = local read "Rotate Image Angle"() -> (w694:bool)
            n310 = case shown="False" w694 {
              tunnel: [w698 w702] -> w695
              tunnel: w692 -> [w698 w700]
              tunnel: w690 -> [_ w701]
              tunnel: w689 -> [_ w699]
              frame False {
              }
              frame True {
                n311 = case shown="False" w701 {
                  tunnel: [w709 w710] -> w703
                  tunnel: w700 -> [w708 w710]
                  tunnel: w699 -> [w707 _]
                  frame False {
                    n312 = call "IMAQ Copy"("Image Dst"=w707, "Image Src"=w708) -> ("Image Dst Out"=w709:T3)  [unwired: 4 in, 1 out]
                  }
                  frame True {
                  }
                }
                n313 = call "[FGV]Parameters.vi"("Parameter"=Parameter."Read") -> ("ParameterData Out"=w705:T28)  [unwired: 9 in, 1 out]
                n314 = Unbundle By Name(w705) -> ("Rotate Angle"=w704:dbl)
                n315 = call "IMAQ Rotate"("Angle (degrees)"=w704, "Image Src"=w703) -> ("Image Dst Out"=w702:T3)  [unwired: 8 in, 1 out]
              }
            }
            n316 = local write "Vision_Image"(w695) -> ()
          }
          frame "SingleRunWithoutCaliper" {
            # "沒有影像輸入的錯誤碼"
            n317 = call "Imaq GetImageInfo"("Image"=w713) -> ("error out"=w715:errorcluster)  [unwired: 3 in, 7 out]
            n318 = Unbundle By Name(w715) -> ("code"=w717:i32)
            n319 = Equal?(x=w717, y=-1074396120) -> (x = y?=w714:bool)
            n320 = case shown="False" w714 {
              tunnel: w719 -> [w733 _]
              tunnel: w718 -> [w732 _]
              tunnel: w713 -> [w731 _]
              frame False {
                n321 = property on="SEQ_Name" class="Ring (strict)"() -> ("Strings []"=w746:string[], "Value"=w745:u16)  [unwired: 2 in, 2 out]
                n322 = disable-structure shown="Enabled" {
                  disable-tunnel: w731 -> [w750 w751]
                  disable-tunnel: [w749 w751] -> w730
                  frame Enabled {
                    n323 = call "IMAQ Clear Overlay"("Image"=w750) -> ("Image Out"=w749:T3)  [unwired: 9 in, 1 out]
                  }
                  frame Disabled {
                  }
                }
                n324 = Index Array(array=w746, index=w745) -> (element=w744:string)
                n325 = call "[FGV] ROI_List.vi"("Action"=ROI_List_Action."Get All ROI") -> ("All ROI"=w747:T29[])  [unwired: 8 in, 2 out]
                n326 = case shown="False" w733 {
                  tunnel: w730 -> [w752 w756]
                  tunnel: [w752 w755] -> w729
                  tunnel: [_ w754] -> w720
                  tunnel: w732 -> [_ w753]
                  frame False {
                  }
                  frame True {
                    n327 = call "RunCoordinateSys.vi"("RootPath"=w753, "Image In"=w756) -> ("Coordinate System Out"=w754:T37, "Vision_Image Out"=w755:T3)  [unwired: 5 in, 3 out]
                  }
                }
                n328 = for {
                  tunnel: w747 -> [w771] mode=indexing
                  tunnel: w729 -> [w782]
                  tunnel: [w777] -> w735 mode=indexing
                  tunnel: w732 -> [w776]
                  tunnel: w744 -> [w775]
                  shift-right: [w772] -> w722
                  shift-left: T15[] [] ("Analysis_Point_Result") -> [w774]
                  tunnel: [w771] -> w741 mode=indexing
                  shift-right: [w766] -> w726
                  shift-left: T15[] [] -> [w767]
                  tunnel: w720 -> [w765]
                  n329 = call "Extract_ROI_Image.vi"("Coordinate System Out"=w765, "ROI Entry"=w771, "ImageIn"=w782) -> ("error out"=w783:errorcluster, "ForCalCalculaton Out"=w770:T3, "ExtractedOriginalImage"=w780:T3)  [unwired: 6 in]
                  n330 = call "Process_ROI_Image.vi"("error in (no error)"=w783, "ForCalCalculaton In"=w770, "ROI Entry"=w771, "ImageIn"=w780) -> ("error out"=w781:errorcluster, "ForCalCalculaton Out"=w769:T3, "ExtractedProcessedImage"=w778:T3)  [unwired: 5 in]
                  n331 = call "Analyze_ROI_Image.vi"("ImageIn"=w778, "ProjectName"=w775, "ForCalCalculaton In"=w769, "ROI Entry"=w771, "Coordinate System In"=w765, "error in (no error)"=w781, "RootPath"=w776) -> ("AnalysisResult"=w777:variant, "Analysis_Point_Result Out Overlay"=w768:T15[], "Analysis_Point_Result"=w773:T15[], "error out"=w779:errorcluster)  [unwired: 4 in, 1 out]
                  n332 = Build Array (concatenate)(w774, w773) -> (w772:T15[])
                  n333 = Build Array (concatenate)(w767, w768) -> (w766:T15[])
                  n334 = disable-structure shown="Enabled" {
                    disable-tunnel: w780 -> [w786 _]
                    disable-tunnel: w779 -> [w785 _]
                    disable-tunnel: w778 -> [w784 _]
                    frame Disabled {
                      n335 = call "IMAQ Dispose"("Image"=w786, "error in (no error)"=w785) -> ()  [unwired: 4 in, 1 out]
                      n336 = call "IMAQ Dispose"("Image"=w784, "error in (no error)"=w785) -> ()  [unwired: 4 in, 1 out]
                    }
                    frame Enabled {
                    }
                  }
                }
                n337 = call "[FGV] Analysis_Result_Points.vi"("Action"=AnalysisResultPointsAction."ReplaceAll", "Analysis_Point_Result"=w722) -> ("error out"=w734:errorcluster)  [unwired: 8 in, 1 out]
                n338 = call "[FGV] Analysis_Result_Points_Overlay.vi"("Action"=AnalysisResultPointsAction."ReplaceAll", "Analysis_Point_Result"=w726) -> ()  [unwired: 8 in, 2 out]
                n339 = for {
                  tunnel: w741 -> [w763] mode=indexing
                  tunnel: w735 -> [w762] mode=indexing
                  tunnel: [w761] -> w740
                  tunnel: w734 -> [_]
                  n340 = control-ref of="Vision_Image"() -> (w764:refnum<vi>)
                  n341 = call "Update_Analized_Overlay.vi"("ROI Entry"=w763, "AnalysisResult"=w762, "Image Refnum"=w764) -> ("error out"=w761:errorcluster)  [unwired: 7 in, 1 out]
                }
                n342 = call "[FGV] CaliperEntry.vi"("Action"=Caliper_Entry_FGV_Action."ReadAll") -> ("AllCaliperEntries"=w738:T23[])  [unwired: 9 in, 1 out]
                n343 = call "[FGV] CaliperEntry_Overlay.vi"("Action"=Caliper_Entry_FGV_Action."ReadAll") -> ("AllCaliperEntries"=w724:T23[])  [unwired: 9 in, 1 out]
                n344 = call "Caliper Setting UI.vi"("Coor?"=FALSE, "error in (no error)"=w740, "CaliperEntryIn Overlay In"=w724, "CaliperEntryIn"=w738, "Vision_Image"=w729) -> ("CaliperEntryOut Overlay"=w723:T23[], "CaliperEntryOut"=w736:T23[], "Cancel?"=w737:bool)  [unwired: 3 in, 1 out]
                n345 = case shown="False" w737 {
                  tunnel: w736 -> [w759 _]
                  tunnel: w723 -> [w757 _]
                  frame False {
                    n346 = call "[FGV] CaliperEntry.vi"("Action"=Caliper_Entry_FGV_Action."ReplaceAll", "CaliperEntriesIn"=w759) -> ()  [unwired: 8 in, 2 out]
                    n347 = call "[FGV] CaliperEntry_Overlay.vi"("Action"=Caliper_Entry_FGV_Action."ReplaceAll", "CaliperEntriesIn"=w757) -> ()  [unwired: 8 in, 2 out]
                  }
                  frame True {
                  }
                }
              }
              frame True {
                n348 = One Button Dialog(message="Not an image.", button name ("OK")="Stop") -> ()  [unwired: 1 out]
              }
            }
          }
          frame "UpdateSelecedOutput" {
            n349 = call "[FGV] Output List.vi"("Action"=T16."Read All") -> ("Output"=w791:T41)  [unwired: 9 in, 1 out]
            n350 = property on="Analysis Result" class="MCListbox (strict)"() -> ("ItemNames"=w796:string[][])  [unwired: 2 in, 2 out]
            n351 = Unbundle(w791) -> ("OutputList"=w790:u16[], "Criteria Condition"=w789:string[])
            n352 = for {
              tunnel: w790 -> [w805] mode=indexing
              shift-right: [w806] -> w795
              shift-left: string[][] [] ("Item Names") -> [w808]
              tunnel: w796 -> [w807]
              tunnel: w789 -> [w803] mode=indexing
              n353 = Index Array(array=w807, index (row)=w805) -> (element=w800:string[])  [unwired: 1 in]
              n354 = Index Array(array=w800, index=2) -> (element=w798:string)
              n355 = call "UpdateCriteriaResult.vi"("Data ain"=w798, "Criteria In"=w803) -> ("PASS?"=w801:string, "Criteria"=w802:string)  [unwired: 7 in, 1 out]
              n356 = Build Array (concatenate)(w800, w802, w801) -> (w804:string[])
              n357 = Build Array (concatenate)(w808, w804) -> (w806:string[][])
            }
            n358 = property on="Output List" class="MCListbox (strict)"("ItemNames"=w795) -> ()  [unwired: 2 in, 2 out]
          }
          frame "UpdateCaliper" {
            n359 = call "[FGV] CaliperEntry.vi"("Action"=Caliper_Entry_FGV_Action."ReadAll") -> ("AllCaliperEntries"=w813:T23[])  [unwired: 9 in, 1 out]
            n360 = for {
              tunnel: w813 -> [w816] mode=indexing
              tunnel: [w815] -> w812 mode=indexing
              n361 = Unbundle By Name(w816) -> ("StepName"=w815:string)
            }
            n362 = property on="CaliperList" class="LstBox (strict)"("Item Names"=w812, "Value"=i32[] [] ("CaliperList")) -> ()  [unwired: 2 in, 2 out]
          }
          frame "AddNewSeq" {
            # "要直接開folder?"
            n363 = property on="SEQ_Name" class="Ring (strict)"() -> ("Strings []"=w824:string[])  [unwired: 2 in, 2 out]
            n364 = local read "ProjectNameOut"() -> (w819:string)
            n365 = Replace Array Subset(array=w824, new element=w819, index=0) -> (w821:string[])
            n366 = property on="SEQ_Name" class="Ring (strict)"("Strings []"=w821, "Value"=u16 0) -> (error out=w825:errorcluster)  [unwired: 2 in, 1 out]
            n367 = case shown="True" TRUE {
              tunnel: w825 -> [_ _]
              tunnel: w819 -> [_ w829]
              tunnel: [_ w826] -> _
              frame False {
              }
              frame True {
                n368 = property on="RootPath" class="Path"() -> ("Value"=w827:path)  [unwired: 2 in, 2 out]
                n369 = Build Path(base path=w827, name or relative path="Data") -> (appended path=w830:path)
                n370 = Build Path(base path=w830, name or relative path=w829) -> (appended path=w828:path)
                n371 = Create Folder(path (use dialog)=w828) -> (error out=w826:errorcluster)  [unwired: 2 in, 2 out]
              }
            }
          }
          frame "SaveVisionSEQ" {
            # "#iV_Version\n4"
            n372 = call <vilib>:"Set Busy.vi"() -> ("error out"=w836:errorcluster)  [unwired: 10 in, 1 out]
            n373 = property on="Analysis Result" class="MCListbox (strict)"() -> ("ItemNames"=w840:string[][])  [unwired: 2 in, 2 out]
            n374 = property on="RootPath" class="Path"() -> ("Value"=w839:path)  [unwired: 2 in, 2 out]
            n375 = property on="SEQ_Name" class="Ring (strict)"(error in=w836) -> ("Strings []"=w834:string[], "Value"=w833:u16)  [unwired: 1 in, 2 out]
            n376 = Index Array(array=w834, index=w833) -> (element=w832:string)
            n377 = call "SaveVseq.vi"("ProjectName"=w832, "ItemNames"=w840, "RootPath"=w839) -> ("error out"=w835:errorcluster)  [unwired: 8 in]
            n378 = call <vilib>:"Unset Busy.vi"("error in (no error)"=w835) -> ()  [unwired: 10 in, 1 out]
          }
          frame "Init User Parameter" {
            w843 = T4 0 items=["None", "PatternMatch", "Edge Detection", "Barcode 1D", "Barcode 2D", "Clamp", "Clamp MAX", "Particle", "Histogram", "Straight Edge", "Circle", "Shape Detect", "OCR", "Contour", "ColorMatch"] ("Analysis Function")
            n379 = invoke on="Vision_Image" class="ImageControl" method="Reinit To Default"() -> ()  [unwired: 3 in, 3 out]
            n380 = property on="Process Steps" class="MCListbox (strict)"("Value"=0 ("Process Steps"), "ItemNames"=string[][] [] ("Item Names")) -> ()  [unwired: 2 in, 2 out]
            n381 = property on="Analysis Function" class="Ring (strict)"("Value"=w843) -> ()  [unwired: 2 in, 2 out]
            n382 = property on="CaliperList" class="LstBox (strict)"("Item Names"=string[] [], "Value"=i32[] [] ("CaliperList")) -> ()  [unwired: 2 in, 2 out]
            n383 = control-ref of="CameraName"() -> (w848:refnum<vi>)
            n384 = call "Camera_SetCameraRing.vi"("Camera Index"=u16 0, "CameraName"=w848) -> ()  [unwired: 9 in, 1 out]
            n385 = call "[FGV] ROI_List.vi"("Action"=ROI_List_Action."Init") -> ()  [unwired: 8 in, 3 out]
            n386 = call "CoordinateDataEntry.vi"("CoordinateAction"=CoordinateAction."Initialize") -> ()  [unwired: 9 in, 2 out]
            n387 = call "[FGV] Output List.vi"("Action"=T9."Init") -> ()  [unwired: 9 in, 2 out]
            n388 = call "[FGV] Analysis_Result_Points.vi"("Action"=AnalysisResultPointsAction."Init") -> ()  [unwired: 9 in, 2 out]
            n389 = call "[FGV] Analysis_Result_Points_Overlay.vi"("Action"=AnalysisResultPointsAction."Init") -> ()  [unwired: 9 in, 2 out]
            n390 = call "[FGV] CaliperEntry.vi"("Action"=Caliper_Entry_FGV_Action."Init") -> ()  [unwired: 9 in, 2 out]
            n391 = call "[FGV] CaliperEntry_Overlay.vi"("Action"=Caliper_Entry_FGV_Action."Init") -> ()  [unwired: 9 in, 2 out]
            n392 = call "[FGV]Parameters.vi"("Parameter"=Parameter."Initialize") -> ()  [unwired: 9 in, 2 out]
          }
          frame "Cont.Run" {
            n393 = case shown="True" "ContRun" {
              tunnel: w861 -> [w863 w866]
              tunnel: [w863 w864] -> w860
              frame False {
              }
              frame True {
                w865 = TRUE  # Cont.Run
                n394 = Generate User Event(user event=w866, event data cluster=w865) -> (user event out=w864:refnum<user-event>)  [unwired: 2 in, 1 out]
              }
            }
          }
          frame "Idle" {
          }
        }
      }
    }
    frame Enabled {
    }
  }
  n395 = disable-structure shown="Disabled" {
    disable-tunnel: w24 -> [w875 _]
    disable-tunnel: [w874 _] -> w19
    disable-tunnel: w17 -> [w873 _]
    disable-tunnel: [w872 _] -> w12
    disable-tunnel: w10 -> [w871 _]
    disable-tunnel: w4 -> [w870 _]
    disable-tunnel: "Real Position Info" -> [w869 _]
    frame Disabled {
      n396 = while {
        tunnel: w875 -> [w886]
        tunnel: w870 -> [w885]
        shift-right: [w878] -> _
        shift-left: _ -> [w884]
        shift-right: [w883] -> w874
        shift-left: _ -> [w882]
        tunnel: w873 -> [w881]
        tunnel: [w880] -> w872
        tunnel: w871 -> [w879]
        tunnel: w869 -> [w876]
        stop <- w877 stop-if-true
        n397 = event shown="[17] \"SingleRun\": Value Change" {
          selector: w881 -> [_ _ _ _ _ _ _ _ _ _ _ _ _ _ _ _ _ _ _ _ _ _ _ _ _ _ _ _ _ _ _]
          dyn-events: [_ _ _ _ _ _ _ _ _ _ _ _ _ _ _ _ _ _ _ _ _ _ _ _ _ _ _ _ _ _ _] -> w880
          timeout: _ -> [_ _ _ _ _ _ _ _ _ _ _ _ _ _ _ _ _ _ _ _ _ _ _ _ _ _ _ _ _ _ _]
          tunnel: w886 -> [_ w896 w920 w955 w967 w1211 w1233 w1242 w1248 w1276 _ _ w1289 w1325 _ w1373 w1383 w1411 w1471 _ _ w1498 w1505 w1509 _ w1631 w1648 _ w1727 w1778 w1842]
          tunnel: w885 -> [_ w895 w919 w956 w964 _ w1232 w1241 w1247 w1275 _ _ _ w1324 _ w1371 w1379 _ w1470 _ _ _ _ w1508 _ w1633 w1647 _ w1726 _ w1841]
          tunnel: [w888 _ w929 w957 w965 w1212 w1231 w1240 w1249 w1278 w1280 w1283 w1284 w1330 w1357 w1378 w1386 w1413 w1472 w1474 w1484 w1495 w1501 w1515 w1624 w1634 w1645 w1718 w1730 w1776 w1847] -> w878
          tunnel: w884 -> [w888 w898 w929 w957 w966 w1212 w1231 w1240 w1249 w1278 w1280 w1283 _ w1330 w1357 w1378 _ _ w1472 w1474 w1484 w1495 w1501 w1515 w1624 w1634 w1646 w1718 w1730 _ w1847]
          tunnel: [w887 w890 w914 w951 w958 w1208 w1229 w1238 w1246 w1271 w1279 w1282 w1285 w1329 w1356 w1377 w1380 w1410 w1462 w1473 w1481 w1494 w1500 w1512 w1623 w1635 w1642 w1719 w1729 w1777 w1839] -> w883
          tunnel: w882 -> [w887 w890 w914 w951 w958 w1208 w1229 w1238 w1246 w1271 w1279 w1282 w1285 w1329 w1356 w1377 w1380 w1410 w1462 w1473 w1481 w1494 w1500 w1511 w1623 w1635 w1642 w1719 w1729 w1777 w1840]
          tunnel: [_ TRUE _ _ _ _ _ _ _ _ _ _ _ _ _ _ _ _ _ _ _ _ _ _ _ _ _ _ _ _ _] -> w877
          tunnel: w879 -> [_ _ _ _ _ _ _ _ _ _ _ _ _ _ _ _ _ _ _ _ _ _ _ w1510 _ _ _ _ _ _ _]
          tunnel: w876 -> [_ _ _ _ _ _ _ _ _ _ _ _ _ _ _ _ _ _ _ _ _ _ _ w1507 _ _ _ _ _ _ _]
          event Timeout {
            n398 = event-data() -> ()  [unwired: 1 in, 2 out]
          }
          event "ExitVisionEditor": Value Change {
            n399 = event-data() -> ()  [unwired: 1 in, 1 out]
            n400 = call "[FGV]Button Click Frequency.vi"("Command"=enum16{"Initialize", "Add", "Read"}."Read") -> ("Value"=w893:i32)  [unwired: 9 in, 1 out]
            n401 = Greater Or Equal?(x=w893, y=1) -> (x >= y?=w891:bool)
            n402 = case shown="True" w891 {
              tunnel: [FALSE ("T button?") w901] -> w897
              frame False {
              }
              frame True {
                n403 = Two Button Dialog(message="Do You Want Save File?", 1:"Canel" ("F button name (\"Cancel\")"), 2:"OK" ("T button name (\"OK\")")) -> (T button?=w901:bool)
              }
            }
            n404 = case shown="False" w897 {
              tunnel: w896 -> [w906 w910]
              tunnel: w895 -> [w905 w909]
              frame False {
                n405 = Enqueue Element(queue=w906, element=UI_Action."Exit", error in (no error)=w905) -> ()  [unwired: 1 in, 3 out]
              }
              frame True {
                w908 = T5[] [enum."SaveVisionSEQ", enum."Exit"] items=["Init Setting", "Get Root Path", "Exit", "ActivateAllControls", "UpdateROIListbox", "UpdateSelectROIOverlay", "UpdateUIOverlay", "UpdateSelectedOverlay", "ConfigAnalysis", "ConfigProcess", "UpdateExistProjNames", "Init Result Page", "UpdateResultTable", "Init Menu", "Activate Menu", "UpdateProcess", "UpdateAnalysis", "SingleRun", "UpdateSelecedOutput", "ReloadResultTable", "SingleRunWithoutCaliper", "AddNewSeq", "UpdateCaliper", "SaveVisionSEQ", "Init User Parameter", "Cont.Run", "CalRotateImage", "Idle", "UpdateInitStatus", "Initilaize Camera", "Init Read Template", ""]
                n406 = for {
                  tunnel: w910 -> [w913]
                  tunnel: w909 -> [w912]
                  tunnel: w908 -> [w911] mode=indexing
                  n407 = Enqueue Element(queue=w913, element=w911, error in (no error)=w912) -> ()  [unwired: 1 in, 3 out]
                }
              }
            }
            n408 = call "IMAQ Dispose"("Image"=w898) -> ("error out"=w899:errorcluster)  [unwired: 5 in]
            n409 = call <vilib>:"General Error Handler.vi"("error in (no error)"=w899) -> ()  [unwired: 2 in, 13 out]
          }
          event "NewVisionSEQ": Value Change {
            # "要直接開folder?"
            n410 = event-data() -> ()  [unwired: 1 in, 1 out]
            n411 = call "[FGV]Button Click Frequency.vi"("Command"=enum16{"Initialize", "Add", "Read"}."Read") -> ("Value"=w925:i32)  [unwired: 9 in, 1 out]
            n412 = Greater Or Equal?(x=w925, y=1) -> (x >= y?=w926:bool)
            n413 = case shown="True" w926 {
              tunnel: [FALSE w950] -> w924
              tunnel: w920 -> [w943 w946]
              tunnel: w919 -> [w942 w945]
              tunnel: [w943 w946] -> w918
              tunnel: [w942 w945] -> w917
              frame False {
              }
              frame True {
                n414 = Two Button Dialog(message="Do You Want Save File?", 1:"No" ("F button name (\"Cancel\")"), 2:"Yes" ("T button name (\"OK\")")) -> (T button?=w950:bool)
              }
            }
            n415 = property on="SEQ_Name" class="Ring (strict)"(error in=w917) -> (error out=w916:errorcluster, "Strings []"=w923:string[])  [unwired: 1 in, 1 out]
            n416 = call "Get Project Name.vi"("error in (no error)"=w916, "ProjectNamesIn"=w923) -> ("error out"=w915:errorcluster, "ProjectNameOut"=→"ProjectNameOut":string, "Cancel?"=w922:bool)  [unwired: 7 in]
            n417 = invoke on="Vision_Image" class="ImageControl" method="Clear ROI"() -> ()  [unwired: 3 in, 3 out]
            n418 = case shown="False" w922 {
              tunnel: w918 -> [w935 _]
              tunnel: w915 -> [w934 _]
              tunnel: w924 -> [w933 _]
              frame False {
                n419 = case shown="False" w933 {
                  tunnel: [w936 w937] -> w930
                  frame False {
                    w936 = T5[] [enum."UpdateExistProjNames", enum."AddNewSeq", enum."ActivateAllControls", enum."Activate Menu", enum."Init User Parameter", enum."UpdateROIListbox", enum."UpdateUIOverlay", enum."UpdateInitStatus"] items=["Init Setting", "Get Root Path", "Exit", "ActivateAllControls", "UpdateROIListbox", "UpdateSelectROIOverlay", "UpdateUIOverlay", "UpdateSelectedOverlay", "ConfigAnalysis", "ConfigProcess", "UpdateExistProjNames", "Init Result Page", "UpdateResultTable", "Init Menu", "Activate Menu", "UpdateProcess", "UpdateAnalysis", "SingleRun", "UpdateSelecedOutput", "ReloadResultTable", "SingleRunWithoutCaliper", "AddNewSeq", "UpdateCaliper", "SaveVisionSEQ", "Init User Parameter", "Cont.Run", "CalRotateImage", "Idle", "UpdateInitStatus", "Initilaize Camera", "Init Read Template", ""]
                  }
                  frame True {
                    w937 = T5[] [enum."SaveVisionSEQ", enum."UpdateExistProjNames", enum."AddNewSeq", enum."ActivateAllControls", enum."Activate Menu", enum."Init User Parameter", enum."UpdateROIListbox", enum."UpdateUIOverlay"] items=["Init Setting", "Get Root Path", "Exit", "ActivateAllControls", "UpdateROIListbox", "UpdateSelectROIOverlay", "UpdateUIOverlay", "UpdateSelectedOverlay", "ConfigAnalysis", "ConfigProcess", "UpdateExistProjNames", "Init Result Page", "UpdateResultTable", "Init Menu", "Activate Menu", "UpdateProcess", "UpdateAnalysis", "SingleRun", "UpdateSelecedOutput", "ReloadResultTable", "SingleRunWithoutCaliper", "AddNewSeq", "UpdateCaliper", "SaveVisionSEQ", "Init User Parameter", "Cont.Run", "CalRotateImage", "Idle", "UpdateInitStatus", "Initilaize Camera", "Init Read Template", ""]
                  }
                }
                n420 = for {
                  tunnel: w935 -> [w941]
                  tunnel: w934 -> [w940]
                  tunnel: w930 -> [w939] mode=indexing
                  tunnel: [w938] -> w931
                  n421 = Enqueue Element(queue=w941, element=w939, error in (no error)=w940) -> (error out=w938:errorcluster)  [unwired: 1 in, 2 out]
                }
                n422 = call "[FGV]Button Click Frequency.vi"("error in (no error)"=w931, "Command"=enum16{"Initialize", "Add", "Read"}."Add") -> ()  [unwired: 8 in, 2 out]
              }
              frame True {
              }
            }
          }
          event "SaveVisionSEQ": Value Change {
            n423 = event-data() -> ()  [unwired: 1 in, 1 out]
            n424 = Enqueue Element(queue=w955, element=UI_Action."SaveVisionSEQ", error in (no error)=w956) -> (error out=w952:errorcluster)  [unwired: 1 in, 2 out]
            n425 = call "[FGV]Button Click Frequency.vi"("error in (no error)"=w952, "Command"=enum16{"Initialize", "Add", "Read"}."Initialize") -> ()  [unwired: 8 in, 2 out]
          }
          event "SEQ_Name": Value Change {
            n426 = event-data() -> ("OldVal"=w959:u16)  [unwired: 1 in]
            n427 = call "[FGV]Button Click Frequency.vi"("Command"=enum16{"Initialize", "Add", "Read"}."Read") -> ("Value"=w962:i32)  [unwired: 9 in, 1 out]
            n428 = Greater Or Equal?(x=w962, y=1) -> (x >= y?=w960:bool)
            n429 = case shown="True" w960 {
              tunnel: [FALSE w973] -> w968
              frame False {
              }
              frame True {
                n430 = Two Button Dialog(message="Do You Want Save File?", 1:"NO" ("F button name (\"Cancel\")"), 2:"Yes" ("T button name (\"OK\")")) -> (T button?=w973:bool)
              }
            }
            n431 = case shown="False" w968 {
              tunnel: w967 -> [w991 w1074]
              tunnel: w966 -> [w990 w1075]
              tunnel: [w990 w1075] -> w965
              tunnel: w964 -> [w988 w1073]
              tunnel: w959 -> [_ w1072]
              frame False {
                # "#iV_Version\n3"
                n432 = property on="RootPath" class="Path"() -> ("Value"=w994:path)  [unwired: 2 in, 2 out]
                n433 = property on="SEQ_Name" class="Ring (strict)"() -> ("Strings []"=w1007:string[], "Value"=w1008:u16)  [unwired: 2 in, 2 out]
                n434 = call "[FGV]Button Click Frequency.vi"("error in (no error)"=w988, "Command"=enum16{"Initialize", "Add", "Read"}."Add") -> ("error out"=w987:errorcluster)  [unwired: 8 in, 1 out]
                n435 = Index Array(array=w1007, index=w1008) -> (element=w1004:string)
                n436 = Build Path(base path=w994, name or relative path="Data") -> (appended path=w1005:path)
                n437 = Build Path(base path=w1005, name or relative path=w1004) -> (appended path=w979:path)
                n438 = Build Path(base path=w979, name or relative path="Seq Data") -> (appended path=w975:path)
                n439 = Open/Create/Replace File(file path (use dialog)=w975, error in=w987, operation (0:open)=T43."open") -> (refnum out=w999:refnum<file>, error out=w1002:errorcluster)  [unwired: 3 in, 1 out]
                n440 = Build Path(base path=w979, name or relative path="Seq Data.db") -> (appended path=w980:path)
                n441 = Read from Binary File(5:T42 {"iVision_Version"="", "iVisionSEQParam"=variant} ("iVisionSEQ"), 8:w1002, 11:w999) -> (0:w1001:errorcluster, 2:w983:T42, 3:w998:refnum<file>)  [unwired: 3 in, 1 out]
                n442 = Unbundle(w983) -> ("iVision_Version"=w982:string, "iVisionSEQParam"=w981:variant)
                n443 = Close File(refnum=w998, error in=w1001) -> ()  [unwired: 2 out]
                n444 = case shown="\"iV_V1\"" w982 {
                  tunnel: [_ w1016 w1032] -> w997
                  tunnel: [_ w1015 w1031] -> w996
                  tunnel: [_ w1013 w1030] -> w993
                  tunnel: [_ w1012 w1029] -> w992
                  tunnel: [_ w1011 w1028] -> w986
                  tunnel: [_ w1010 w1027] -> w985
                  tunnel: w981 -> [_ w1018 w1025]
                  tunnel: [_ w1014 w1023] -> w974
                  frame "False", Default {
                  }
                  frame "iV_V1" {
                    n445 = Variant To Data(type=T44 {"All ROI"=[], "Output"={"OutputList"=[], "Criteria Condition"=[]}, [], "AllCaliperEntries"=[], "CoordinatteEntry Output"={"ProcessSetting"=[], "Project Name"="", "AnalysisSetting"=[], "Coord?"=FALSE}, "ParameterData Out"={"Rotate Angle"=0.0, "Rotate?"=FALSE, "Calibration File Path"="", "Cal?"=FALSE}, "AllCaliperEntries"=[]} ("Old"), Variant=w1018) -> (data=w1020:T44)  [unwired: 1 in, 1 out]
                    n446 = disable-structure shown="Disabled" {
                      disable-tunnel: w1020 -> [w1022 _]
                      disable-tunnel: [w1021 _] -> w1017
                      frame Disabled {
                        n447 = call "V1.0 Convert.vi"("Old"=w1022) -> ("NewOut"=w1021:T45)  [unwired: 10 in]
                      }
                      frame Enabled {
                      }
                    }
                    n448 = Unbundle(w1017) -> ("All ROI"=w1016:T29[], "Output"=w1015:T41, w1014:string[][], "AllCaliperEntries"=w1013:T23[], "CoordinatteEntry Output"=w1012:T17, "ParameterData Out"=w1011:T28, "AllCaliperEntries"=w1010:T23[])
                  }
                  frame "iV_V1.6" {
                    n449 = Variant To Data(type=T45 {"All ROI"=[], "Output"={"OutputList"=[], "Criteria Condition"=[]}, [], "AllCaliperEntries"=[], "CoordinatteEntry Output"={"ProcessSetting"=[], "Project Name"="", "AnalysisSetting"=[], "Coord?"=FALSE, "OriginPointInfo"={"Output Original"=FALSE, "Origin Name"="", "Angle"=0.0, "Mode"=0, "OriginPoint"={"X"=0.0, "Y"=0.0}}, "CaliperSetting"=[], "CoordIndex"=[]}, "ParameterData Out"={"Rotate Angle"=0.0, "Rotate?"=FALSE, "Calibration File Path"="", "Cal?"=FALSE}, "AllCaliperEntries"=[]} ("output cluster"), Variant=w1025) -> (data=w1024:T45)  [unwired: 1 in, 1 out]
                    n450 = Unbundle(w1024) -> ("All ROI"=w1032:T29[], "Output"=w1031:T41, w1023:string[][], "AllCaliperEntries"=w1030:T23[], "CoordinatteEntry Output"=w1029:T17, "ParameterData Out"=w1028:T28, "AllCaliperEntries"=w1027:T23[])
                  }
                }
                n451 = call <vilib>:"Check if File or Folder Exists.vi"("path"=w980) -> ("error out"=w977:errorcluster, "file or folder exists?"=w976:bool)  [unwired: 8 in, 1 out]
                n452 = case shown="No Error" w977 {
                  tunnel: [w1042 w1067] -> w1009
                  tunnel: w997 -> [w1043 _]
                  tunnel: w996 -> [w1044 _]
                  tunnel: [w1039 errorcluster {"status"=FALSE, "code"=0, "source"=""} ("error IO")] -> w995
                  tunnel: w993 -> [w1041 _]
                  tunnel: w992 -> [w1040 _]
                  tunnel: w986 -> [w1038 _]
                  tunnel: w985 -> [w1037 _]
                  tunnel: w976 -> [w1036 _]
                  tunnel: w975 -> [w1035 _]
                  tunnel: w974 -> [w1033 _]
                  frame No Error {
                    w1042 = T5[] [enum."ActivateAllControls", enum."Activate Menu", enum."Init Result Page", enum."UpdateROIListbox", enum."UpdateUIOverlay", enum."UpdateProcess", enum."UpdateAnalysis", enum."UpdateCaliper", enum."ReloadResultTable", enum."UpdateSelecedOutput", enum."UpdateInitStatus", enum."Init Read Template"] items=["Init Setting", "Get Root Path", "Exit", "ActivateAllControls", "UpdateROIListbox", "UpdateSelectROIOverlay", "UpdateUIOverlay", "UpdateSelectedOverlay", "ConfigAnalysis", "ConfigProcess", "UpdateExistProjNames", "Init Result Page", "UpdateResultTable", "Init Menu", "Activate Menu", "UpdateProcess", "UpdateAnalysis", "SingleRun", "UpdateSelecedOutput", "ReloadResultTable", "SingleRunWithoutCaliper", "AddNewSeq", "UpdateCaliper", "SaveVisionSEQ", "Init User Parameter", "Cont.Run", "CalRotateImage", "Idle", "UpdateInitStatus", "Initilaize Camera", "Init Read Template", ""]
                    n453 = case shown="True" w1036 {
                      tunnel: w1044 -> [w1058 _]
                      tunnel: w1043 -> [w1057 _]
                      tunnel: w1041 -> [w1055 _]
                      tunnel: w1040 -> [w1053 _]
                      tunnel: [w1052 w1063] -> w1039
                      tunnel: w1038 -> [w1050 _]
                      tunnel: w1037 -> [w1048 _]
                      tunnel: w1035 -> [_ w1065]
                      tunnel: [w1045 w1064] -> w1034
                      tunnel: w1033 -> [w1045 _]
                      frame False {
                        n454 = call "[FGV] Output List.vi"("Action"=T9."Remove All") -> ("error out"=w1059:errorcluster)  [unwired: 9 in, 1 out]
                        n455 = call "CoordinateDataEntry.vi"("CoordinateAction"=CoordinateAction."CoordEntryInput", "OneCoordStep Input"=w1053) -> ()  [unwired: 8 in, 2 out]
                        n456 = Unbundle(w1058) -> ("OutputList"=w1047:u16[], "Criteria Condition"=w1046:string[])
                        n457 = call "[FGV]Parameters.vi"("Parameter"=Parameter."WriteAll", "ParameterData In"=w1050) -> ()  [unwired: 8 in, 2 out]
                        n458 = call "[FGV] ROI_List.vi"("ROIEntriesIn"=w1057, "Action"=ROI_List_Action."Replace All Entries") -> ()  [unwired: 7 in, 3 out]
                        n459 = call "[FGV] Output List.vi"("Action"=T9."Add", "error in (no error)"=w1059, "Criteria"=w1046, "Indexes In"=w1047) -> ()  [unwired: 6 in, 2 out]
                        n460 = call "[FGV] CaliperEntry.vi"("Action"=Caliper_Entry_FGV_Action."ReplaceAll", "CaliperEntriesIn"=w1055) -> ("error out"=w1052:errorcluster)  [unwired: 8 in, 1 out]
                        n461 = call "[FGV] CaliperEntry_Overlay.vi"("Action"=Caliper_Entry_FGV_Action."ReplaceAll", "CaliperEntriesIn"=w1048) -> ()  [unwired: 8 in, 2 out]
                      }
                      frame True {
                        n462 = call "ReadVisionSeqData.vi"("SeqDataPath"=w1065) -> ("error out"=w1063:errorcluster, "AnalysisResult"=w1064:string[][])  [unwired: 9 in]
                      }
                    }
                    n463 = local write "Item Names"(w1034) -> ()
                  }
                  frame Error {
                    w1067 = T5[] [enum."ActivateAllControls", enum."Activate Menu", enum."Idle"] items=["Init Setting", "Get Root Path", "Exit", "ActivateAllControls", "UpdateROIListbox", "UpdateSelectROIOverlay", "UpdateUIOverlay", "UpdateSelectedOverlay", "ConfigAnalysis", "ConfigProcess", "UpdateExistProjNames", "Init Result Page", "UpdateResultTable", "Init Menu", "Activate Menu", "UpdateProcess", "UpdateAnalysis", "SingleRun", "UpdateSelecedOutput", "ReloadResultTable", "SingleRunWithoutCaliper", "AddNewSeq", "UpdateCaliper", "SaveVisionSEQ", "Init User Parameter", "Cont.Run", "CalRotateImage", "Idle", "UpdateInitStatus", "Initilaize Camera", "Init Read Template", ""]
                  }
                }
                n464 = for {
                  tunnel: w991 -> [w1071]
                  tunnel: w995 -> [w1070]
                  tunnel: w1009 -> [w1069] mode=indexing
                  tunnel: [w1068] -> _
                  n465 = Enqueue Element(queue=w1071, element=w1069, error in (no error)=w1070) -> (error out=w1068:errorcluster)  [unwired: 1 in, 2 out]
                }
              }
              frame True {
                n466 = stacked-sequence {
                  tunnel: w1074 -> [_ w1123]
                  tunnel: w1073 -> [_ w1122]
                  tunnel: w1072 -> [w1084 _]
                  frame #0 {
                    # "#iV_Version\n6"
                    n467 = property on="RootPath" class="Path"() -> ("Value"=w1093:path)  [unwired: 2 in, 2 out]
                    n468 = property on="SEQ_Name" class="Ring (strict)"() -> ("Strings []"=w1085:string[])  [unwired: 2 in, 2 out]
                    n469 = property on="Analysis Result" class="MCListbox (strict)"() -> ("ItemNames"=w1091:string[][])  [unwired: 2 in, 2 out]
                    n470 = Index Array(array=w1085, index=w1084) -> (element=w1106:string)
                    n471 = Build Path(base path=w1093, name or relative path="Data") -> (appended path=w1107:path)
                    n472 = Array Subset(array=w1091, length (col)=2 ("length")) -> (w1090:string[][])  [unwired: 3 in]
                    n473 = Build Path(base path=w1107, name or relative path=w1106) -> (appended path=w1097:path)
                    n474 = Build Path(base path=w1097, name or relative path="Seq Data") -> (appended path=w1096:path)
                    n475 = call "[FGV] ROI_List.vi"("Action"=ROI_List_Action."Get All ROI") -> ("All ROI"=w1099:T29[])  [unwired: 8 in, 2 out]
                    n476 = call "[FGV] Output List.vi"("Action"=T9."Read All") -> ("Output"=w1098:T41)  [unwired: 9 in, 1 out]
                    n477 = call "[FGV] CaliperEntry.vi"("Action"=Caliper_Entry_FGV_Action."ReadAll") -> ("AllCaliperEntries"=w1088:T23[])  [unwired: 9 in, 1 out]
                    n478 = call "CoordinateDataEntry.vi"("CoordinateAction"=CoordinateAction."CoordEntryOutput") -> ("CoordinatteEntry Output"=w1086:T17)  [unwired: 9 in, 1 out]
                    n479 = call "[FGV]Parameters.vi"("Parameter"=Parameter."Read") -> ("ParameterData Out"=w1082:T28)  [unwired: 9 in, 1 out]
                    n480 = call "[FGV] CaliperEntry_Overlay.vi"("Action"=Caliper_Entry_FGV_Action."ReplaceAll") -> ("AllCaliperEntries"=w1080:T23[])  [unwired: 9 in, 1 out]
                    n481 = global read "[Global]iVision_Version.vi" "iVision_Version"() -> (w1076:string)
                    n482 = Open/Create/Replace File(file path (use dialog)=w1096, operation (0:open)=T43."open or create") -> (refnum out=w1105:refnum<file>, error out=w1103:errorcluster)  [unwired: 4 in, 1 out]
                    n483 = Bundle("All ROI"=w1099, "Output"=w1098, w1090, "AllCaliperEntries"=w1088, "CoordinatteEntry Output"=w1086, "ParameterData Out"=w1082, "AllCaliperEntries"=w1080) -> (w1078:T45)  [unwired: 1 in]
                    n484 = Bundle(cluster=T42 {"iVision_Version"="", "iVisionSEQParam"=variant} ("iVisionSEQ"), "iVision_Version"=w1076, "iVisionSEQParam"=w1078) -> (w1077:T42)
                    n485 = Write to Binary File(file (use dialog)=w1105, data=w1077, error in=w1103) -> (refnum out=w1104:refnum<file>, error out=w1102:errorcluster)  [unwired: 3 in, 1 out]
                    n486 = Close File(refnum=w1104, error in=w1102) -> ()  [unwired: 2 out]
                  }
                  frame #1 {
                    # "#iV_Version\n5"
                    n487 = property on="SEQ_Name" class="Ring (strict)"() -> ("Strings []"=w1141:string[], "Value"=w1142:u16)  [unwired: 2 in, 2 out]
                    n488 = property on="RootPath" class="Path"() -> ("Value"=w1128:path)  [unwired: 2 in, 2 out]
                    n489 = call "[FGV]Button Click Frequency.vi"("error in (no error)"=w1122, "Command"=enum16{"Initialize", "Add", "Read"}."Add") -> ("error out"=w1124:errorcluster)  [unwired: 8 in, 1 out]
                    n490 = Index Array(array=w1141, index=w1142) -> (element=w1138:string)
                    n491 = Build Path(base path=w1128, name or relative path="Data") -> (appended path=w1139:path)
                    n492 = Build Path(base path=w1139, name or relative path=w1138) -> (appended path=w1115:path)
                    n493 = Build Path(base path=w1115, name or relative path="Seq Data") -> (appended path=w1111:path)
                    n494 = Build Path(base path=w1115, name or relative path="Seq Data.db") -> (appended path=w1113:path)
                    n495 = Open/Create/Replace File(file path (use dialog)=w1111, error in=w1124, operation (0:open)=T43."open") -> (refnum out=w1133:refnum<file>, error out=w1136:errorcluster)  [unwired: 3 in, 1 out]
                    n496 = Read from Binary File(5:T42 {"iVision_Version"="", "iVisionSEQParam"=variant} ("iVisionSEQ"), 8:w1136, 11:w1133) -> (0:w1135:errorcluster, 2:w1118:T42, 3:w1132:refnum<file>)  [unwired: 3 in, 1 out]
                    n497 = Unbundle(w1118) -> ("iVision_Version"=w1117:string, "iVisionSEQParam"=w1116:variant)
                    n498 = Close File(refnum=w1132, error in=w1135) -> ()  [unwired: 2 out]
                    n499 = call <vilib>:"Check if File or Folder Exists.vi"("path"=w1113) -> ("error out"=w1109:errorcluster, "file or folder exists?"=w1112:bool)  [unwired: 8 in, 1 out]
                    n500 = case shown="\"iV_V1.6\"" w1117 {
                      tunnel: [_ w1150 w1167] -> w1131
                      tunnel: [_ w1149 w1166] -> w1130
                      tunnel: [_ w1148 w1165] -> w1110
                      tunnel: [_ w1147 w1164] -> w1127
                      tunnel: [_ w1146 w1163] -> w1126
                      tunnel: [_ w1145 w1162] -> w1121
                      tunnel: [_ w1144 w1161] -> w1120
                      tunnel: w1116 -> [_ w1154 w1159]
                      frame "False", Default {
                      }
                      frame "iV_V1" {
                        n501 = Variant To Data(type=T44 {"All ROI"=[], "Output"={"OutputList"=[], "Criteria Condition"=[]}, [], "AllCaliperEntries"=[], "CoordinatteEntry Output"={"ProcessSetting"=[], "Project Name"="", "AnalysisSetting"=[], "Coord?"=FALSE}, "ParameterData Out"={"Rotate Angle"=0.0, "Rotate?"=FALSE, "Calibration File Path"="", "Cal?"=FALSE}, "AllCaliperEntries"=[]} ("Old"), Variant=w1154) -> (data=w1152:T44)  [unwired: 1 in, 1 out]
                        n502 = disable-structure shown="Disabled" {
                          disable-tunnel: w1152 -> [w1156 _]
                          disable-tunnel: [w1155 _] -> w1151
                          frame Disabled {
                            n503 = call "V1.0 Convert.vi"("Old"=w1156) -> ("NewOut"=w1155:T45)  [unwired: 10 in]
                          }
                          frame Enabled {
                          }
                        }
                        n504 = Unbundle(w1151) -> ("All ROI"=w1150:T29[], "Output"=w1149:T41, w1148:string[][], "AllCaliperEntries"=w1147:T23[], "CoordinatteEntry Output"=w1146:T17, "ParameterData Out"=w1145:T28, "AllCaliperEntries"=w1144:T23[])
                      }
                      frame "iV_V1.6" {
                        n505 = Variant To Data(type=T45 {"All ROI"=[], "Output"={"OutputList"=[], "Criteria Condition"=[]}, [], "AllCaliperEntries"=[], "CoordinatteEntry Output"={"ProcessSetting"=[], "Project Name"="", "AnalysisSetting"=[], "Coord?"=FALSE, "OriginPointInfo"={"Output Original"=FALSE, "Origin Name"="", "Angle"=0.0, "Mode"=0, "OriginPoint"={"X"=0.0, "Y"=0.0}}, "CaliperSetting"=[], "CoordIndex"=[]}, "ParameterData Out"={"Rotate Angle"=0.0, "Rotate?"=FALSE, "Calibration File Path"="", "Cal?"=FALSE}, "AllCaliperEntries"=[]} ("output cluster"), Variant=w1159) -> (data=w1158:T45, error out=w1157:errorcluster)  [unwired: 1 in]
                        n506 = Unbundle(w1158) -> ("All ROI"=w1167:T29[], "Output"=w1166:T41, w1165:string[][], "AllCaliperEntries"=w1164:T23[], "CoordinatteEntry Output"=w1163:T17, "ParameterData Out"=w1162:T28, "AllCaliperEntries"=w1161:T23[])
                        n507 = call <vilib>:"Clear Errors.vi"("error in (no error)"=w1157) -> ()  [unwired: 5 in, 2 out]
                      }
                    }
                    n508 = case shown="No Error" w1109 {
                      tunnel: [w1179 w1203] -> w1143
                      tunnel: w1131 -> [w1180 _]
                      tunnel: w1130 -> [w1174 _]
                      tunnel: [w1176 errorcluster {"status"=FALSE, "code"=0, "source"=""} ("error IO")] -> w1129
                      tunnel: w1127 -> [w1178 _]
                      tunnel: w1126 -> [w1177 _]
                      tunnel: w1121 -> [w1175 _]
                      tunnel: w1120 -> [w1173 _]
                      tunnel: w1112 -> [w1172 _]
                      tunnel: w1111 -> [w1171 _]
                      tunnel: w1110 -> [w1170 _]
                      tunnel: w1110 -> [w1168 _]
                      frame No Error {
                        w1179 = T5[] [enum."ActivateAllControls", enum."Activate Menu", enum."Init Result Page", enum."UpdateROIListbox", enum."UpdateUIOverlay", enum."UpdateProcess", enum."UpdateAnalysis", enum."UpdateCaliper", enum."ReloadResultTable", enum."UpdateSelecedOutput", enum."UpdateInitStatus", enum."Init Read Template"] items=["Init Setting", "Get Root Path", "Exit", "ActivateAllControls", "UpdateROIListbox", "UpdateSelectROIOverlay", "UpdateUIOverlay", "UpdateSelectedOverlay", "ConfigAnalysis", "ConfigProcess", "UpdateExistProjNames", "Init Result Page", "UpdateResultTable", "Init Menu", "Activate Menu", "UpdateProcess", "UpdateAnalysis", "SingleRun", "UpdateSelecedOutput", "ReloadResultTable", "SingleRunWithoutCaliper", "AddNewSeq", "UpdateCaliper", "SaveVisionSEQ", "Init User Parameter", "Cont.Run", "CalRotateImage", "Idle", "UpdateInitStatus", "Initilaize Camera", "Init Read Template", ""]
                        n509 = case shown="True" w1172 {
                          tunnel: w1180 -> [w1195 _]
                          tunnel: w1178 -> [w1193 _]
                          tunnel: w1177 -> [w1191 _]
                          tunnel: [w1190 w1199] -> w1176
                          tunnel: w1175 -> [w1188 _]
                          tunnel: w1174 -> [w1185 _]
                          tunnel: w1173 -> [w1182 _]
                          tunnel: w1171 -> [_ w1201]
                          tunnel: w1170 -> [_ _]
                          tunnel: [w1181 w1200] -> w1169
                          tunnel: w1168 -> [w1181 _]
                          frame False {
                            n510 = call "[FGV] Output List.vi"("Action"=T16."Remove All") -> ("error out"=w1196:errorcluster)  [unwired: 9 in, 1 out]
                            n511 = call "CoordinateDataEntry.vi"("CoordinateAction"=CoordinateAction."CoordEntryInput", "OneCoordStep Input"=w1191) -> ()  [unwired: 8 in, 2 out]
                            n512 = call "[FGV] ROI_List.vi"("ROIEntriesIn"=w1195, "Action"=ROI_List_Action."Replace All Entries") -> ()  [unwired: 7 in, 3 out]
                            n513 = Unbundle(w1185) -> ("OutputList"=w1184:u16[], "Criteria Condition"=w1183:string[])
                            n514 = call "[FGV]Parameters.vi"("Parameter"=Parameter."WriteAll", "ParameterData In"=w1188) -> ()  [unwired: 8 in, 2 out]
                            n515 = call "[FGV] Output List.vi"("Action"=T9."Add", "error in (no error)"=w1196, "Criteria"=w1183, "Indexes In"=w1184) -> ()  [unwired: 6 in, 2 out]
                            n516 = call "[FGV] CaliperEntry.vi"("Action"=Caliper_Entry_FGV_Action."ReplaceAll", "CaliperEntriesIn"=w1193) -> ("error out"=w1190:errorcluster)  [unwired: 8 in, 1 out]
                            n517 = call "[FGV] CaliperEntry_Overlay.vi"("Action"=Caliper_Entry_FGV_Action."ReplaceAll", "CaliperEntriesIn"=w1182) -> ()  [unwired: 8 in, 2 out]
                          }
                          frame True {
                            n518 = call "ReadVisionSeqData.vi"("SeqDataPath"=w1201) -> ("error out"=w1199:errorcluster, "AnalysisResult"=w1200:string[][])  [unwired: 9 in]
                          }
                        }
                        "Item Names" <- w1169
                      }
                      frame Error {
                        w1203 = T5[] [enum."ActivateAllControls", enum."Activate Menu", enum."Idle"] items=["Init Setting", "Get Root Path", "Exit", "ActivateAllControls", "UpdateROIListbox", "UpdateSelectROIOverlay", "UpdateUIOverlay", "UpdateSelectedOverlay", "ConfigAnalysis", "ConfigProcess", "UpdateExistProjNames", "Init Result Page", "UpdateResultTable", "Init Menu", "Activate Menu", "UpdateProcess", "UpdateAnalysis", "SingleRun", "UpdateSelecedOutput", "ReloadResultTable", "SingleRunWithoutCaliper", "AddNewSeq", "UpdateCaliper", "SaveVisionSEQ", "Init User Parameter", "Cont.Run", "CalRotateImage", "Idle", "UpdateInitStatus", "Initilaize Camera", "Init Read Template", ""]
                      }
                    }
                    n519 = for {
                      tunnel: w1123 -> [w1207]
                      tunnel: w1129 -> [w1206]
                      tunnel: w1143 -> [w1205] mode=indexing
                      tunnel: [w1204] -> _
                      n520 = Enqueue Element(queue=w1207, element=w1205, error in (no error)=w1206) -> (error out=w1204:errorcluster)  [unwired: 1 in, 2 out]
                    }
                  }
                }
              }
            }
          }
          event "ConfigROI": Value Change {
            n521 = event-data() -> ()  [unwired: 1 in, 1 out]
            n522 = Not Equal?(x=w1212, y=T3 refnum ("Image Out")) -> (x != y?=w1209:bool)
            n523 = case shown="True" w1209 {
              tunnel: w1212 -> [_ w1216]
              tunnel: w1211 -> [_ w1215]
              frame False {
                n524 = One Button Dialog(message="Please Acquire Image First") -> ()  [unwired: 1 in, 1 out]
              }
              frame True {
                n525 = call "ROI_Setting_UI.vi"("Vision_Image"=w1216) -> ("error out"=w1214:errorcluster)  [unwired: 10 in]
                n526 = disable-structure shown="Enabled" {
                  disable-tunnel: w1215 -> [w1222 w1225]
                  disable-tunnel: w1214 -> [w1221 w1224]
                  frame Disabled {
                    n527 = Enqueue Element(queue=w1222, element=UI_Action."UpdateROIListbox", error in (no error)=w1221) -> (queue out=w1219:refnum<queue>, error out=w1218:errorcluster)  [unwired: 1 in, 1 out]
                    n528 = Enqueue Element(queue=w1219, element=UI_Action."UpdateUIOverlay", error in (no error)=w1218) -> ()  [unwired: 1 in, 3 out]
                  }
                  frame Enabled {
                    w1223 = T5[] [enum."UpdateROIListbox", enum."UpdateUIOverlay", enum."UpdateProcess", enum."UpdateAnalysis", enum."UpdateCaliper", enum."UpdateResultTable", enum."UpdateSelecedOutput"] items=["Init Setting", "Get Root Path", "Exit", "ActivateAllControls", "UpdateROIListbox", "UpdateSelectROIOverlay", "UpdateUIOverlay", "UpdateSelectedOverlay", "ConfigAnalysis", "ConfigProcess", "UpdateExistProjNames", "Init Result Page", "UpdateResultTable", "Init Menu", "Activate Menu", "UpdateProcess", "UpdateAnalysis", "SingleRun", "UpdateSelecedOutput", "ReloadResultTable", "SingleRunWithoutCaliper", "AddNewSeq", "UpdateCaliper", "SaveVisionSEQ", "Init User Parameter", "Cont.Run", "CalRotateImage", "Idle", "UpdateInitStatus", "Initilaize Camera", "Init Read Template", ""]
                    n529 = for {
                      tunnel: w1225 -> [w1228]
                      tunnel: w1224 -> [w1227]
                      tunnel: w1223 -> [w1226] mode=indexing
                      n530 = Enqueue Element(queue=w1228, element=w1226, error in (no error)=w1227) -> ()  [unwired: 1 in, 3 out]
                    }
                  }
                }
              }
            }
          }
          event "ROI List": Mouse Down {
            w1230 = T5[] [enum."UpdateSelectROIOverlay", enum."UpdateProcess", enum."UpdateAnalysis", enum."UpdateCaliper"] items=["Init Setting", "Get Root Path", "Exit", "ActivateAllControls", "UpdateROIListbox", "UpdateSelectROIOverlay", "UpdateUIOverlay", "UpdateSelectedOverlay", "ConfigAnalysis", "ConfigProcess", "UpdateExistProjNames", "Init Result Page", "UpdateResultTable", "Init Menu", "Activate Menu", "UpdateProcess", "UpdateAnalysis", "SingleRun", "UpdateSelecedOutput", "ReloadResultTable", "SingleRunWithoutCaliper", "AddNewSeq", "UpdateCaliper", "SaveVisionSEQ", "Init User Parameter", "Cont.Run", "CalRotateImage", "Idle", "UpdateInitStatus", "Initilaize Camera", "Init Read Template", ""]
            n531 = event-data() -> ()  [unwired: 1 in, 8 out]
            n532 = for {
              tunnel: w1233 -> [w1236]
              tunnel: w1232 -> [w1235]
              tunnel: w1230 -> [w1234] mode=indexing
              n533 = Enqueue Element(queue=w1236, element=w1234, error in (no error)=w1235) -> ()  [unwired: 1 in, 3 out]
            }
          }
          event "ROI List": Double Click {
            w1239 = T5[] [enum."UpdateSelectedOverlay", enum."UpdateProcess", enum."UpdateAnalysis", enum."UpdateCaliper"] items=["Init Setting", "Get Root Path", "Exit", "ActivateAllControls", "UpdateROIListbox", "UpdateSelectROIOverlay", "UpdateUIOverlay", "UpdateSelectedOverlay", "ConfigAnalysis", "ConfigProcess", "UpdateExistProjNames", "Init Result Page", "UpdateResultTable", "Init Menu", "Activate Menu", "UpdateProcess", "UpdateAnalysis", "SingleRun", "UpdateSelecedOutput", "ReloadResultTable", "SingleRunWithoutCaliper", "AddNewSeq", "UpdateCaliper", "SaveVisionSEQ", "Init User Parameter", "Cont.Run", "CalRotateImage", "Idle", "UpdateInitStatus", "Initilaize Camera", "Init Read Template", ""]
            n534 = event-data() -> ()  [unwired: 1 in, 9 out]
            n535 = for {
              tunnel: w1242 -> [w1245]
              tunnel: w1241 -> [w1244]
              tunnel: w1239 -> [w1243] mode=indexing
              n536 = Enqueue Element(queue=w1245, element=w1243, error in (no error)=w1244) -> ()  [unwired: 1 in, 3 out]
            }
            n537 = local write "Boolean"(TRUE) -> ()
          }
          event "ConfigAnalysis": Value Change {
            n538 = event-data() -> ()  [unwired: 1 in, 1 out]
            n539 = disable-structure shown="Enabled" {
              disable-tunnel: w1248 -> [w1258 w1263]
              disable-tunnel: w1247 -> [w1257 w1262]
              frame Disabled {
                n540 = Enqueue Element(queue=w1258, element=UI_Action."ConfigAnalysis", error in (no error)=w1257) -> (queue out=w1252:refnum<queue>, error out=w1250:errorcluster)  [unwired: 1 in, 1 out]
                n541 = Enqueue Element(queue=w1252, element=UI_Action."UpdateAnalysis", error in (no error)=w1250) -> (queue out=w1253:refnum<queue>, error out=w1251:errorcluster)  [unwired: 1 in, 1 out]
                n542 = Enqueue Element(queue=w1253, element=UI_Action."UpdateResultTable", error in (no error)=w1251) -> ()  [unwired: 1 in, 3 out]
              }
              frame Enabled {
                n543 = Enqueue Element(queue=w1263, element=UI_Action."ConfigAnalysis", error in (no error)=w1262) -> (queue out=w1266:refnum<queue>, error out=w1264:errorcluster)  [unwired: 1 in, 1 out]
                n544 = Enqueue Element(queue=w1266, element=UI_Action."UpdateAnalysis", error in (no error)=w1264) -> (queue out=w1267:refnum<queue>, error out=w1265:errorcluster)  [unwired: 1 in, 1 out]
                n545 = Enqueue Element(queue=w1267, element=UI_Action."UpdateResultTable", error in (no error)=w1265) -> (queue out=w1261:refnum<queue>, error out=w1260:errorcluster)  [unwired: 1 in, 1 out]
                n546 = Enqueue Element(queue=w1261, element=UI_Action."Init Read Template", error in (no error)=w1260) -> ()  [unwired: 1 in, 3 out]
              }
            }
          }
          event "ConfigProcess": Value Change {
            n547 = event-data() -> ()  [unwired: 1 in, 1 out]
            n548 = Enqueue Element(queue=w1276, element=UI_Action."ConfigProcess", error in (no error)=w1275) -> (queue out=w1273:refnum<queue>, error out=w1272:errorcluster)  [unwired: 1 in, 1 out]
            n549 = Enqueue Element(queue=w1273, element=UI_Action."UpdateProcess", error in (no error)=w1272) -> ()  [unwired: 1 in, 3 out]
          }
          event "Function_Tab": Value Change {
            # "Need to Load Entry According to Specified ROI"
            n550 = event-data() -> ()  [unwired: 1 in, 6 out]
          }
          event "Main_Tab": Value Change {
            w1281 = T46 {"Row"=0, "Column"=0} ("Top Left Visible Cell")
            n551 = event-data() -> ()  [unwired: 1 in, 6 out]
            n552 = property on="Analysis Result" class="MCListbox (strict)"("TopLeft"=w1281) -> ()  [unwired: 2 in, 2 out]
            n553 = property on="Output List" class="MCListbox (strict)"("TopLeft"=w1281) -> ()  [unwired: 2 in, 2 out]
          }
          event "Snap": Value Change {
            # "Jesse : 因為我的webcam的問題, 得改成這樣才拍的到照片"
            n554 = event-data() -> ()  [unwired: 1 in, 1 out]
            n555 = control-ref of="CameraName"() -> (w1287:refnum<vi>)
            n556 = call "Camera_CheckCameraSetting.vi"("CameraName"=w1287) -> ("CameraGot?"=w1288:bool, "Camera Session"=w1286:T47)  [unwired: 9 in]
            n557 = case shown="True" w1288 {
              tunnel: w1289 -> [_ w1296]
              tunnel: [T3 refnum ("New Image") w1294] -> w1284
              tunnel: w1286 -> [_ _]
              frame False {
              }
              frame True {
                w1291 = T5[] [enum."CalRotateImage", enum."UpdateUIOverlay"] items=["Init Setting", "Get Root Path", "Exit", "ActivateAllControls", "UpdateROIListbox", "UpdateSelectROIOverlay", "UpdateUIOverlay", "UpdateSelectedOverlay", "ConfigAnalysis", "ConfigProcess", "UpdateExistProjNames", "Init Result Page", "UpdateResultTable", "Init Menu", "Activate Menu", "UpdateProcess", "UpdateAnalysis", "SingleRun", "UpdateSelecedOutput", "ReloadResultTable", "SingleRunWithoutCaliper", "AddNewSeq", "UpdateCaliper", "SaveVisionSEQ", "Init User Parameter", "Cont.Run", "CalRotateImage", "Idle", "UpdateInitStatus", "Initilaize Camera", "Init Read Template", ""]
                n558 = call "IMAQ Create"("Image Name"="Snap") -> ("New Image"=w1293:T3)  [unwired: 3 in, 2 out]
                n559 = disable-structure shown="Enabled" {
                  disable-tunnel: [w1303 w1312] -> w1295
                  disable-tunnel: [w1302 w1313] -> w1294
                  disable-tunnel: w1293 -> [w1301 w1314]
                  disable-tunnel: T13."Grab" ("Action") -> [_ w1315]
                  frame Disabled {
                    n560 = disable-structure shown="Enabled" {
                      disable-tunnel: [w1307 w1311] -> w1303
                      disable-tunnel: w1301 -> [w1306 w1309]
                      disable-tunnel: [w1305 w1310] -> w1302
                      disable-tunnel: _ -> [w1304 w1308]
                      frame Disabled {
                        n561 = call "Camera_Snap.vi"("Camera Session In"=w1304, "Image In"=w1306) -> ("error out"=w1307:errorcluster, "New Image"=w1305:T3)  [unwired: 8 in]
                      }
                      frame Enabled {
                        n562 = call "Camera_Snap_Jesse.vi"("Camera Session In"=w1308, "Image In"=w1309) -> ("error out"=w1311:errorcluster, "New Image"=w1310:T3)  [unwired: 8 in]
                      }
                    }
                  }
                  frame Enabled {
                    n563 = call "[FGV] Camera Settings.vi"("Action"=w1315, "Image In"=w1314) -> ("error out"=w1312:errorcluster, "Image Out"=w1313:T3)  [unwired: 7 in, 1 out]
                  }
                }
                n564 = for {
                  tunnel: w1296 -> [w1300]
                  tunnel: w1295 -> [w1299]
                  tunnel: w1291 -> [w1298] mode=indexing
                  n565 = Enqueue Element(queue=w1300, element=w1298, error in (no error)=w1299) -> ()  [unwired: 1 in, 3 out]
                }
              }
            }
            "Vision_Image" <- w1284
          }
          event "Vision_Image": Mouse Up {
            n566 = event-data() -> ()  [unwired: 1 in, 1 out]
            n567 = control-ref of="ROI List"() -> (w1326:refnum<vi>)
            n568 = property class="LstBox (strict)"(reference=w1326, error in=w1324) -> ("Item Names"=w1327:string[], "Value"=w1328:i32[])  [unwired: 2 out]
            n569 = property on="Vision_Image" class="ImageControl"() -> ("ROI"=w1321:T48)  [unwired: 2 in, 2 out]
            n570 = Unbundle By Name(w1321) -> ("Contours"=w1322:T49)
            n571 = Index Array(array=w1328) -> (element=w1323:i32)  [unwired: 1 in]
            n572 = Index Array(array=w1322) -> (element=w1317:T50)  [unwired: 1 in]
            n573 = local read "Boolean"() -> (w1316:bool)
            n574 = Index Array(array=w1327, index=w1323) -> (element=w1318:string)
            n575 = call "[FGV] ROI_List.vi"("Action"=ROI_List_Action."Get All ROI") -> ("All ROI"=w1319:T29[])  [unwired: 8 in, 2 out]
            n576 = case shown="True" w1316 {
              tunnel: w1325 -> [_ w1339]
              tunnel: w1319 -> [_ w1338]
              tunnel: w1318 -> [_ w1337]
              tunnel: w1317 -> [_ w1332]
              frame False {
              }
              frame True {
                w1334 = T5[] [enum."UpdateUIOverlay"] items=["Init Setting", "Get Root Path", "Exit", "ActivateAllControls", "UpdateROIListbox", "UpdateSelectROIOverlay", "UpdateUIOverlay", "UpdateSelectedOverlay", "ConfigAnalysis", "ConfigProcess", "UpdateExistProjNames", "Init Result Page", "UpdateResultTable", "Init Menu", "Activate Menu", "UpdateProcess", "UpdateAnalysis", "SingleRun", "UpdateSelecedOutput", "ReloadResultTable", "SingleRunWithoutCaliper", "AddNewSeq", "UpdateCaliper", "SaveVisionSEQ", "Init User Parameter", "Cont.Run", "CalRotateImage", "Idle", "UpdateInitStatus", "Initilaize Camera", "Init Read Template", ""]
                n577 = for {
                  tunnel: w1338 -> [w1346] mode=indexing
                  tunnel: w1337 -> [w1349]
                  tunnel: w1332 -> [w1345]
                  tunnel: [w1347] -> w1335 mode=indexing
                  n578 = Unbundle By Name(w1346) -> ("vROIName"=w1350:string)
                  n579 = Equal?(x=w1350, y=w1349) -> (x = y?=w1348:bool)
                  n580 = case shown="True" w1348 {
                    tunnel: [w1351 w1352] -> w1347
                    tunnel: w1346 -> [w1351 w1354]
                    tunnel: w1345 -> [_ w1353]
                    frame False {
                    }
                    frame True {
                      n581 = Bundle By Name(cluster=w1354, "vROIContour"=w1353) -> (w1352:T29)
                    }
                  }
                }
                n582 = call "[FGV] ROI_List.vi"("ROIEntriesIn"=w1335, "Action"=ROI_List_Action."Replace All Entries") -> ("error out"=w1333:errorcluster)  [unwired: 7 in, 2 out]
                n583 = for {
                  tunnel: w1339 -> [w1344]
                  tunnel: w1333 -> [w1343]
                  tunnel: w1334 -> [w1342] mode=indexing
                  tunnel: [w1341] -> w1331
                  n584 = Enqueue Element(queue=w1344, element=w1342, error in (no error)=w1343) -> (error out=w1341:errorcluster)  [unwired: 1 in, 2 out]
                }
                n585 = flat-sequence {
                  tunnel: w1331 -> [_]
                  frame #0 {
                    n586 = invoke on="Vision_Image" class="ImageControl" method="Clear ROI"() -> ()  [unwired: 3 in, 3 out]
                    n587 = local write "Boolean"(FALSE ("Boolean")) -> ()
                  }
                }
              }
            }
          }
          event "Vision_Image": Shortcut Menu Selection (User) {
            n588 = event-data() -> ("ItemTag"=w1355:string)  [unwired: 1 in, 7 out]
            n589 = case shown="\"Zoom to Fit\"" w1355 {
              frame Default {
              }
              frame "Save Image" {
                n590 = call "File Dialog"("pattern (all files)"="*.png") -> ("selected path"=w1361:path, "cancelled"=w1359:bool, "error out"=w1360:errorcluster)  [unwired: 11 in, 1 out]
                n591 = case shown="False" w1359 {
                  tunnel: w1361 -> [w1363 _]
                  tunnel: w1360 -> [w1362 _]
                  frame False {
                    n592 = call-poly "IMAQ Write File 2"("error in (no error)"=w1362, "File Path"=w1363, "Image"="Snap" ("Image Name")) -> ()  [unwired: 7 in, 2 out]
                  }
                  frame True {
                  }
                }
              }
              frame "Zoom to Fit" {
                n593 = property on="Vision_Image" class="ImageControl"("Zoom to Fit Mode"=TRUE) -> ()  [unwired: 2 in, 2 out]
              }
            }
          }
          event "Angle", "Rotate Image Angle": Value Change {
            n594 = event-data() -> ()  [unwired: 1 in, 6 out]
            n595 = call "[FGV]Parameters.vi"(7:"Parameter"=Parameter."Write" ("Parameter"), "Error In"=w1371, "ParamName"="RotateAngle", 11:"Parameter"="Angle") -> ("Error Out"=w1370:errorcluster)  [unwired: 6 in, 1 out]
            n596 = call "[FGV]Parameters.vi"(7:"Parameter"=Parameter."Write" ("Parameter"), "Error In"=w1370, "ParamName"="Rotate?", 11:"Parameter"="Rotate Image Angle") -> ("Error Out"=w1366:errorcluster)  [unwired: 6 in, 1 out]
            n597 = Enqueue Element(queue=w1373, element=UI_Action."CalRotateImage", error in (no error)=w1366) -> ()  [unwired: 1 in, 3 out]
          }
          event "GetImage": Value Change {
            n598 = event-data() -> ()  [unwired: 1 in, 3 out]
            n599 = local read "CycleThruFolder"() -> (w1381:bool)
            n600 = case shown="False" w1381 {
              tunnel: [w1387 w1389] -> w1385
              frame False {
                n601 = property on="File Path" class="Path"() -> ("Value"=w1387:path)  [unwired: 2 in, 2 out]
              }
              frame True {
                n602 = control-ref of="Folder Image Files"() -> (w1388:refnum<vi>)
                n603 = call "ImageFile_GetFolderImageAndRotate.vi"("Folder Image Files"=w1388) -> ("File Path"=w1389:path)  [unwired: 9 in, 1 out]
              }
            }
            n604 = call <vilib>:"Check if File or Folder Exists.vi"("path"=w1385) -> ("file or folder exists?"=w1384:bool, "dup path"=w1382:path)  [unwired: 8 in, 1 out]
            n605 = case shown="True" w1384 {
              tunnel: w1383 -> [_ w1396]
              tunnel: [T3 refnum ("New Image") w1392] -> w1386
              tunnel: w1382 -> [_ w1394]
              tunnel: w1379 -> [_ w1391]
              frame False {
              }
              frame True {
                n606 = call "IMAQ GetFileInfo"("File Path"=w1394) -> ("error out"=w1393:errorcluster, "Image Type"=w1395:T32)  [unwired: 4 in, 5 out]
                n607 = case shown="No Error" w1393 {
                  tunnel: w1396 -> [w1404 _]
                  tunnel: w1395 -> [w1403 _]
                  tunnel: [w1401 _] -> w1392
                  tunnel: w1394 -> [w1400 _]
                  tunnel: w1391 -> [w1397 _]
                  frame No Error {
                    w1398 = T5[] [enum."CalRotateImage", enum."UpdateUIOverlay"] items=["Init Setting", "Get Root Path", "Exit", "ActivateAllControls", "UpdateROIListbox", "UpdateSelectROIOverlay", "UpdateUIOverlay", "UpdateSelectedOverlay", "ConfigAnalysis", "ConfigProcess", "UpdateExistProjNames", "Init Result Page", "UpdateResultTable", "Init Menu", "Activate Menu", "UpdateProcess", "UpdateAnalysis", "SingleRun", "UpdateSelecedOutput", "ReloadResultTable", "SingleRunWithoutCaliper", "AddNewSeq", "UpdateCaliper", "SaveVisionSEQ", "Init User Parameter", "Cont.Run", "CalRotateImage", "Idle", "UpdateInitStatus", "Initilaize Camera", "Init Read Template", ""]
                    n608 = call "IMAQ Create"("Image Name"="Snap", "Image Type"=w1403) -> ("New Image"=w1402:T3)  [unwired: 2 in, 2 out]
                    n609 = call "ImageFile_GetSingleImage.vi"("error in (no error)"=w1397, "File Path"=w1400, "Image In"=w1402) -> ("error out"=w1399:errorcluster, "New Image"=w1401:T3)  [unwired: 7 in]
                    n610 = for {
                      tunnel: w1404 -> [w1408]
                      tunnel: w1399 -> [w1407]
                      tunnel: w1398 -> [w1406] mode=indexing
                      n611 = Enqueue Element(queue=w1408, element=w1406, error in (no error)=w1407) -> ()  [unwired: 1 in, 3 out]
                    }
                  }
                  frame Error {
                    n612 = One Button Dialog(message="Please select an image") -> ()  [unwired: 1 in, 1 out]
                  }
                }
              }
            }
          }
          event "SingleRun": Value Change {
            n613 = event-data() -> ()  [unwired: 1 in, 1 out]
            n614 = property on="File Path" class="Path"() -> ("Visible"=w1414:bool)  [unwired: 2 in, 2 out]
            n615 = case shown="True" w1414 {
              tunnel: [w1420 w1450] -> w1413
              tunnel: [w1421 w1445] -> w1412
              frame False {
                n616 = control-ref of="CameraName"() -> (w1419:refnum<vi>)
                n617 = call "Camera_CheckCameraSetting.vi"("CameraName"=w1419) -> ("CameraGot?"=w1423:bool, "Camera Session"=w1422:T47)  [unwired: 9 in]
                n618 = case shown="True" w1423 {
                  tunnel: [T3 refnum ("New Image") w1427] -> w1420
                  tunnel: w1422 -> [_ _]
                  tunnel: [errorcluster {"status"=TRUE, "code"=0, "source"=""} ("error out") w1426] -> w1421
                  frame False {
                  }
                  frame True {
                    n619 = call "IMAQ Create"("Image Name"="Snap") -> ("New Image"=w1428:T3)  [unwired: 3 in, 2 out]
                    n620 = disable-structure shown="Disabled" {
                      disable-tunnel: w1428 -> [w1432 w1443]
                      disable-tunnel: [w1431 w1442] -> w1427
                      disable-tunnel: [w1430 w1441] -> w1426
                      frame Disabled {
                        n621 = disable-structure shown="Enabled" {
                          disable-tunnel: [w1436 w1440] -> w1430
                          disable-tunnel: w1432 -> [w1435 w1438]
                          disable-tunnel: [w1434 w1439] -> w1431
                          disable-tunnel: _ -> [w1433 w1437]
                          frame Disabled {
                            n622 = call "Camera_Snap.vi"("Camera Session In"=w1433, "Image In"=w1435) -> ("error out"=w1436:errorcluster, "New Image"=w1434:T3)  [unwired: 8 in]
                          }
                          frame Enabled {
                            n623 = call "Camera_Snap_Jesse.vi"("Camera Session In"=w1437, "Image In"=w1438) -> ("error out"=w1440:errorcluster, "New Image"=w1439:T3)  [unwired: 8 in]
                          }
                        }
                      }
                      frame Enabled {
                        n624 = call "[FGV] Camera Settings.vi"("Action"=T13."Grab", "Image In"=w1443) -> ("error out"=w1441:errorcluster, "Image Out"=w1442:T3)  [unwired: 7 in, 1 out]
                      }
                    }
                  }
                }
              }
              frame True {
                n625 = local read "CycleThruFolder"() -> (w1446:bool)
                n626 = case shown="True" w1446 {
                  tunnel: [w1451 w1453] -> w1449
                  frame False {
                    n627 = local read "File Path"() -> (w1451:path)
                  }
                  frame True {
                    n628 = control-ref of="Folder Image Files"() -> (w1452:refnum<vi>)
                    n629 = call "ImageFile_GetFolderImageAndRotate.vi"("Folder Image Files"=w1452) -> ("File Path"=w1453:path)  [unwired: 9 in, 1 out]
                  }
                }
                n630 = call <vilib>:"Check if File or Folder Exists.vi"("path"=w1449) -> ("file or folder exists?"=w1448:bool, "dup path"=w1447:path)  [unwired: 8 in, 1 out]
                n631 = case shown="True" w1448 {
                  tunnel: [T3 refnum ("New Image") w1458] -> w1450
                  tunnel: w1447 -> [_ w1457]
                  tunnel: [errorcluster {"status"=TRUE, "code"=0, "source"=""} ("error out") w1456] -> w1445
                  frame False {
                  }
                  frame True {
                    n632 = call "IMAQ GetFileInfo"("File Path"=w1457) -> ("Image Type"=w1460:T32)  [unwired: 4 in, 6 out]
                    n633 = call "IMAQ Create"("Image Name"="Snap", "Image Type"=w1460) -> ("New Image"=w1459:T3)  [unwired: 2 in, 2 out]
                    n634 = call "ImageFile_GetSingleImage.vi"("File Path"=w1457, "Image In"=w1459) -> ("error out"=w1456:errorcluster, "New Image"=w1458:T3)  [unwired: 8 in]
                  }
                }
              }
            }
            n635 = case shown="No Error" w1412 {
              tunnel: w1411 -> [w1416 _]
              frame No Error {
                w1415 = T5[] [enum."Idle", enum."CalRotateImage", enum."SingleRun", enum."UpdateSelecedOutput"] items=["Init Setting", "Get Root Path", "Exit", "ActivateAllControls", "UpdateROIListbox", "UpdateSelectROIOverlay", "UpdateUIOverlay", "UpdateSelectedOverlay", "ConfigAnalysis", "ConfigProcess", "UpdateExistProjNames", "Init Result Page", "UpdateResultTable", "Init Menu", "Activate Menu", "UpdateProcess", "UpdateAnalysis", "SingleRun", "UpdateSelecedOutput", "ReloadResultTable", "SingleRunWithoutCaliper", "AddNewSeq", "UpdateCaliper", "SaveVisionSEQ", "Init User Parameter", "Cont.Run", "CalRotateImage", "Idle", "UpdateInitStatus", "Initilaize Camera", "Init Read Template", ""]
                n636 = for {
                  tunnel: w1416 -> [w1418]
                  tunnel: w1415 -> [w1417] mode=indexing
                  n637 = Enqueue Element(queue=w1418, element=w1417) -> ()  [unwired: 2 in, 3 out]
                }
              }
              frame Error {
              }
            }
          }
          event "ConfigureCaliper": Value Change {
            n638 = event-data() -> ()  [unwired: 1 in, 1 out]
            n639 = Enqueue Element(queue=w1471, element=UI_Action."SingleRunWithoutCaliper", error in (no error)=w1470) -> (queue out=w1468:refnum<queue>, error out=w1467:errorcluster)  [unwired: 1 in, 1 out]
            n640 = Enqueue Element(queue=w1468, element=UI_Action."UpdateCaliper", error in (no error)=w1467) -> (queue out=w1465:refnum<queue>, error out=w1464:errorcluster)  [unwired: 1 in, 1 out]
            n641 = Enqueue Element(queue=w1465, element=UI_Action."UpdateResultTable", error in (no error)=w1464) -> ()  [unwired: 1 in, 3 out]
          }
          event "CycleThruFolder": Value Change {
            n642 = event-data() -> ("NewVal"=w1475:bool)  [unwired: 1 in]
            n643 = case shown="True" w1475 {
              frame False {
              }
              frame True {
                n644 = local read "File Path"() -> (w1476:path)
                n645 = call <vilib>:"Check if File or Folder Exists.vi"("path"=w1476) -> ("file or folder exists?"=w1477:bool, "dup path"=w1478:path)  [unwired: 8 in, 1 out]
                n646 = case shown="True" w1477 {
                  tunnel: w1478 -> [_ w1479]
                  frame False {
                  }
                  frame True {
                    n647 = call "ImageFile_GetFolderImageFiles.vi"("File Path"=w1479) -> ("Folder Image Files"=w1480:path[])  [unwired: 9 in, 1 out]
                    n648 = local write "Folder Image Files"(w1480) -> ()
                  }
                }
              }
            }
          }
          event "File Path": Value Change {
            n649 = event-data() -> ("NewVal"=w1482:path)  [unwired: 1 in]
            n650 = property on="CycleThruFolder" class="Bool (strict)"() -> ("Value"=w1483:bool)  [unwired: 2 in, 2 out]
            n651 = case shown="False" w1483 {
              tunnel: w1482 -> [_ w1485]
              frame False {
              }
              frame True {
                n652 = call <vilib>:"Check if File or Folder Exists.vi"("path"=w1485) -> ("file or folder exists?"=w1486:bool, "dup path"=w1487:path)  [unwired: 8 in, 1 out]
                n653 = case shown="True" w1486 {
                  tunnel: w1487 -> [_ w1488]
                  frame False {
                  }
                  frame True {
                    n654 = call "ImageFile_GetFolderImageFiles.vi"("File Path"=w1488) -> ("Folder Image Files"=w1489:path[])  [unwired: 9 in, 1 out]
                    n655 = local write "Folder Image Files"(w1489) -> ()
                  }
                }
              }
            }
          }
          event "AddToOutput": Value Change {
            n656 = event-data() -> ()  [unwired: 1 in, 1 out]
            n657 = property on="Analysis Result" class="MCListbox (strict)"() -> ("Value"=w1493:i32[])  [unwired: 2 in, 2 out]
            n658 = Array Size(array=w1493) -> (size(s)=w1492:i32)
            n659 = Initialize Array("", w1492) -> (w1490:string[])
            n660 = call "[FGV] Output List.vi"("Action"=T9."Add", "Criteria"=w1490, "Indexes In"=w1493) -> ("error out"=w1497:errorcluster)  [unwired: 7 in, 1 out]
            n661 = Enqueue Element(queue=w1498, element=UI_Action."UpdateSelecedOutput", error in (no error)=w1497) -> ()  [unwired: 1 in, 3 out]
          }
          event "RemoveFromList": Value Change {
            n662 = event-data() -> ()  [unwired: 1 in, 1 out]
            n663 = property on="Output List" class="MCListbox (strict)"() -> ("Value"=w1502:i32[])  [unwired: 2 in, 2 out]
            n664 = call "[FGV] Output List.vi"("Action"=T9."Remove", "Indexes In"=w1502) -> ("error out"=w1504:errorcluster)  [unwired: 8 in, 1 out]
            n665 = Enqueue Element(queue=w1505, element=UI_Action."UpdateSelecedOutput", error in (no error)=w1504) -> ()  [unwired: 1 in, 3 out]
          }
          event Menu Selection (User) {
            n666 = event-data() -> ("MenuRef"=w1513:refnum<k9>, "ItemTag"=w1514:string)  [unwired: 1 in]
            n667 = case shown="\"Calibration\"" w1514 {
              tunnel: w1513 -> [w1517 w1533 _ _ _ _]
              tunnel: [w1516 w1532 w1548 w1573 w1607 w1621] -> w1512
              tunnel: w1511 -> [w1516 w1532 w1548 w1576 w1607 w1621]
              tunnel: w1510 -> [_ _ _ w1574 _ _]
              tunnel: w1509 -> [_ _ _ _ w1598 _]
              tunnel: w1508 -> [_ _ _ _ w1597 _]
              tunnel: w1507 -> [_ _ _ w1572 _ _]
              frame "Camera Mode", Default {
                w1518 = FALSE ("checked")
                w1519 = TRUE ("checked")
                w1528 = "Image File Mode" ("message")
                w1523 = "Camera Mode" ("message")
                n668 = Get Menu Item Info(7:w1523, 11:w1517) -> (1:w1520:bool, 2:w1524:string, 3:w1522:refnum<k9>, 6:w1525:T40)  [unwired: 1 in, 3 out]
                n669 = Set Menu Item Info(4:w1525, 6:w1519, 7:w1523, 9:w1520, 10:w1524, 11:w1522) -> (3:w1530:refnum<k9>)  [unwired: 1 in, 1 out]
                n670 = Get Menu Item Info(7:w1528, 11:w1530) -> (1:w1521:bool, 2:w1527:string, 3:w1529:refnum<k9>, 6:w1526:T40)  [unwired: 1 in, 3 out]
                n671 = Set Menu Item Info(4:w1526, 6:w1518, 7:w1528, 9:w1521, 10:w1527, 11:w1529) -> ()  [unwired: 1 in, 2 out]
                n672 = disable-structure shown="Enabled" {
                  disable-tunnel: w1519 -> [w1531 _]
                  frame Enabled {
                    n673 = property on="CameraName" class="Ring (strict)"("Visible"=w1531) -> ()  [unwired: 2 in, 2 out]
                  }
                  frame Disabled {
                  }
                }
                n674 = property on="Snap" class="Bool"("Visible"=w1519) -> ()  [unwired: 2 in, 2 out]
                n675 = property on="CycleThruFolder" class="Bool (strict)"("Visible"=w1518) -> ()  [unwired: 2 in, 2 out]
                n676 = property on="GetImage" class="Bool"("Visible"=w1518) -> ()  [unwired: 2 in, 2 out]
                n677 = property on="File Path" class="Path"("Visible"=w1518) -> ()  [unwired: 2 in, 2 out]
              }
              frame "Image File Mode" {
                w1534 = TRUE ("checked")
                w1535 = FALSE ("checked")
                w1544 = "Image File Mode" ("message")
                w1539 = "Camera Mode" ("message")
                n678 = Get Menu Item Info(7:w1539, 11:w1533) -> (1:w1536:bool, 2:w1540:string, 3:w1538:refnum<k9>, 6:w1541:T40)  [unwired: 1 in, 3 out]
                n679 = Set Menu Item Info(4:w1541, 6:w1535, 7:w1539, 9:w1536, 10:w1540, 11:w1538) -> (3:w1546:refnum<k9>)  [unwired: 1 in, 1 out]
                n680 = Get Menu Item Info(7:w1544, 11:w1546) -> (1:w1537:bool, 2:w1543:string, 3:w1545:refnum<k9>, 6:w1542:T40)  [unwired: 1 in, 3 out]
                n681 = Set Menu Item Info(4:w1542, 6:w1534, 7:w1544, 9:w1537, 10:w1543, 11:w1545) -> ()  [unwired: 1 in, 2 out]
                n682 = disable-structure shown="Enabled" {
                  disable-tunnel: w1535 -> [w1547 _]
                  frame Enabled {
                    n683 = property on="CameraName" class="Ring (strict)"("Visible"=w1547) -> ()  [unwired: 2 in, 2 out]
                  }
                  frame Disabled {
                  }
                }
                n684 = property on="Snap" class="Bool"("Visible"=w1535) -> ()  [unwired: 2 in, 2 out]
                n685 = property on="CycleThruFolder" class="Bool (strict)"("Visible"=w1534) -> ()  [unwired: 2 in, 2 out]
                n686 = property on="GetImage" class="Bool"("Visible"=w1534) -> ()  [unwired: 2 in, 2 out]
                n687 = property on="File Path" class="Path"("Visible"=w1534) -> ()  [unwired: 2 in, 2 out]
              }
              frame "Coordinate Space" {
                w1559 = 0 ("y")
                n688 = local read "Vision_Image"() -> (w1550:T3)
                n689 = call "Imaq GetImageInfo"("Image"=w1550) -> ("error out"=w1555:errorcluster, "Y Resolution"=w1558:i32, "X Resolution"=w1560:i32)  [unwired: 3 in, 5 out]
                n690 = property on="SEQ_Name" class="Ring (strict)"() -> ("Strings []"=w1554:string[], "Value"=w1553:u16)  [unwired: 2 in, 2 out]
                n691 = Index Array(array=w1554, index=w1553) -> (element=w1551:string)
                n692 = call <vilib>:"Clear Errors.vi"("error in (no error)"=w1555) -> ()  [unwired: 5 in, 2 out]
                n693 = property on="RootPath" class="Path"() -> ("Value"=w1549:path)  [unwired: 2 in, 2 out]
                n694 = Not Equal?(x=w1558, y=w1559) -> (x != y?=w1556:bool)
                n695 = Not Equal?(x=w1560, y=w1559) -> (x != y?=w1557:bool)
                n696 = And(x=w1557, y=w1556) -> (x .and. y?=w1552:bool)
                n697 = case shown="True" w1552 {
                  tunnel: w1551 -> [_ w1564]
                  tunnel: w1550 -> [_ w1563]
                  tunnel: w1549 -> [_ w1562]
                  frame False {
                    n698 = One Button Dialog(message="Please load or snap one image ") -> ()  [unwired: 1 in, 1 out]
                  }
                  frame True {
                    n699 = stacked-sequence {
                      tunnel: w1564 -> [_ w1571]
                      tunnel: w1563 -> [_ w1570]
                      tunnel: w1562 -> [_ w1568]
                      frame #0 {
                        n700 = local read "Coordinate On"() -> (w1565:bool)
                        n701 = case shown="True" w1565 {
                          frame False {
                            n702 = call "CoordinateDataEntry.vi"("CoordinateAction"=CoordinateAction."CoordEntryBackup") -> ()  [unwired: 9 in, 2 out]
                          }
                          frame True {
                            n703 = call "CoordinateDataEntry.vi"("CoordinateAction"=CoordinateAction."CoordEntryTemp") -> ()  [unwired: 9 in, 2 out]
                          }
                        }
                      }
                      frame #1 {
                        n704 = call "Coordinate Space_Setting_UI.vi"("RootPath"=w1568, "Project Name"=w1571, "Image In"=w1570) -> ("Origin Set"=w1569:bool)  [unwired: 8 in]
                        n705 = local write "Coordinate Status"(w1569) -> ()
                        n706 = local write "Coordinate On"(w1569) -> ()
                      }
                    }
                  }
                }
              }
              frame "Calibration" {
                n707 = property on="SEQ_Name" class="Ring (strict)"() -> ("Strings []"=w1581:string[], "Value"=w1580:u16)  [unwired: 2 in, 2 out]
                n708 = property on="RootPath" class="Path"() -> ("Value"=w1582:path)  [unwired: 2 in, 2 out]
                n709 = local read "Image Calibration"() -> (w1575:bool)
                n710 = Index Array(array=w1581, index=w1580) -> (element=w1579:string)
                n711 = Equal?(x=w1579, y="") -> (x = y?=w1577:bool)
                n712 = case shown="False" w1577 {
                  tunnel: w1582 -> [w1584 _]
                  tunnel: w1579 -> [w1588 _]
                  tunnel: [w1586 w1593] -> w1573
                  tunnel: w1576 -> [_ w1593]
                  tunnel: w1575 -> [w1583 _]
                  tunnel: w1574 -> [w1589 _]
                  tunnel: w1572 -> [w1590 _]
                  frame False {
                    n713 = control-ref of="CameraName"() -> (w1591:refnum<vi>)
                    n714 = call "Camera_CheckCameraSetting.vi"("CameraName"=w1591) -> ("CameraGot?"=w1585:bool)  [unwired: 9 in, 1 out]
                    n715 = call "Calibration_Setting_UI.vi"("Real Position Info"=w1590, "CamGot?"=w1585, "Cal Info Image"=w1589, "Cal Status In"=w1583, "Root Path"=w1584, "Seq"=w1588) -> ("Calibration Done"=w1587:bool, "CalTemp"=w1586:T3)  [unwired: 3 in, 1 out]
                    n716 = local write "Image Calibration"(w1587) -> ()
                    n717 = local write "Calibration On"(w1587) -> ()
                  }
                  frame True {
                    n718 = One Button Dialog(message="Please select a seqeunce") -> ()  [unwired: 1 in, 1 out]
                  }
                }
                "Cal Info Image" <- w1573
              }
              frame "Auto Loading ROI Setting" {
                w1605 = 0 ("y")
                n719 = local read "Vision_Image"() -> (w1599:T3)
                n720 = property on="SEQ_Name" class="Ring (strict)"() -> ("Strings []"=w1596:string[], "Value"=w1595:u16)  [unwired: 2 in, 2 out]
                n721 = call "Imaq GetImageInfo"("Image"=w1599) -> ("error out"=w1601:errorcluster, "Y Resolution"=w1604:i32, "X Resolution"=w1606:i32)  [unwired: 3 in, 5 out]
                n722 = Index Array(array=w1596, index=w1595) -> (element=w1594:string)
                n723 = call <vilib>:"Clear Errors.vi"("error in (no error)"=w1601) -> ()  [unwired: 5 in, 2 out]
                n724 = Not Equal?(x=w1604, y=w1605) -> (x != y?=w1602:bool)
                n725 = Not Equal?(x=w1606, y=w1605) -> (x != y?=w1603:bool)
                n726 = And(x=w1603, y=w1602) -> (x .and. y?=w1600:bool)
                n727 = case shown="True" w1600 {
                  tunnel: w1599 -> [_ w1616]
                  tunnel: w1598 -> [_ w1611]
                  tunnel: w1597 -> [_ w1610]
                  tunnel: w1594 -> [_ w1608]
                  frame False {
                  }
                  frame True {
                    w1609 = T5[] [enum."UpdateROIListbox", enum."UpdateUIOverlay", enum."UpdateResultTable", enum."UpdateSelecedOutput", enum."Init Read Template"] items=["Init Setting", "Get Root Path", "Exit", "ActivateAllControls", "UpdateROIListbox", "UpdateSelectROIOverlay", "UpdateUIOverlay", "UpdateSelectedOverlay", "ConfigAnalysis", "ConfigProcess", "UpdateExistProjNames", "Init Result Page", "UpdateResultTable", "Init Menu", "Activate Menu", "UpdateProcess", "UpdateAnalysis", "SingleRun", "UpdateSelecedOutput", "ReloadResultTable", "SingleRunWithoutCaliper", "AddNewSeq", "UpdateCaliper", "SaveVisionSEQ", "Init User Parameter", "Cont.Run", "CalRotateImage", "Idle", "UpdateInitStatus", "Initilaize Camera", "Init Read Template", ""]
                    n728 = call "[FGV] ROI_List.vi"("Action"=ROI_List_Action."ROIEntryBackup", "error in (no error)"=w1610) -> ("error out"=w1613:errorcluster)  [unwired: 7 in, 2 out]
                    n729 = property on="RootPath" class="Path"() -> ("Value"=w1614:path)  [unwired: 2 in, 2 out]
                    n730 = call "AutoROI_Setting_UI.vi"("Root"=w1614, "ProjectName"=w1608, "error in (no error)"=w1613, "Vision_Image"=w1616) -> ("error out"=w1612:errorcluster)  [unwired: 7 in]
                    n731 = for {
                      tunnel: w1611 -> [w1620]
                      tunnel: w1612 -> [w1619]
                      tunnel: w1609 -> [w1618] mode=indexing
                      tunnel: [w1617] -> _
                      n732 = Enqueue Element(queue=w1620, element=w1618, error in (no error)=w1619) -> (error out=w1617:errorcluster)  [unwired: 1 in, 2 out]
                    }
                  }
                }
              }
              frame "OCR Training" {
                n733 = call "OCRTraing.vi"() -> ()  [unwired: 12 in]
              }
            }
          }
          event "Coordinate On": Value Change {
            n734 = event-data() -> ()  [unwired: 1 in, 6 out]
            n735 = disable-structure shown="Disabled" {
              disable-tunnel: "Coordinate On" -> [w1628 _]
              frame Disabled {
                n736 = call "CoordinateDataEntry.vi"("CoordinateAction"=CoordinateAction."CoordEntryOutput") -> ("CoordinatteEntry Output"=w1626:T17)  [unwired: 9 in, 1 out]
                n737 = Bundle By Name(cluster=w1626, "Coord?"=w1628) -> (w1625:T17)
                n738 = call "CoordinateDataEntry.vi"("CoordinateAction"=CoordinateAction."CoordEntryInput", "OneCoordStep Input"=w1625) -> ()  [unwired: 8 in, 2 out]
              }
              frame Enabled {
              }
            }
            "Coordinate Status" <- "Coordinate On"
          }
          event "Calibration On": Value Change {
            n739 = event-data() -> ()  [unwired: 1 in, 1 out]
            n740 = flat-sequence {
              tunnel: [w1639] -> w1632
              tunnel: w1631 -> [w1639]
              frame #0 {
                n741 = call "[FGV]Parameters.vi"(7:"Parameter"=Parameter."Write" ("Parameter"), "ParamName"="Cal?", 11:"Parameter"="Calibration On") -> ()  [unwired: 7 in, 2 out]
                "Image Calibration" <- "Calibration On"
              }
            }
            n742 = Enqueue Element(queue=w1632, element=UI_Action."CalRotateImage", error in (no error)=w1633) -> ()  [unwired: 1 in, 3 out]
          }
          event "CreateROI", "RemoveROI": Value Change {
            n743 = event-data() -> ("CtlRef"=w1651:refnum<vi>)  [unwired: 1 in]
            n744 = property class="Bool"(reference=w1651) -> ("Label.Text"=w1650:string)  [unwired: 1 in, 2 out]
            n745 = Not Equal?(x=w1646, y=T3 refnum ("Image Out")) -> (x != y?=w1649:bool)
            n746 = case shown="\"CreateROI\"" w1650 {
              tunnel: w1649 -> [_ w1667 _]
              tunnel: w1648 -> [w1660 w1666 w1702]
              tunnel: w1647 -> [w1659 w1665 w1698]
              tunnel: w1646 -> [w1661 w1664 w1703]
              tunnel: [w1661 w1664 w1703] -> w1645
              tunnel: [w1660 w1663 w1702] -> w1644
              tunnel: [w1659 w1662 w1692] -> w1643
              frame "-1", Default {
              }
              frame "CreateROI" {
                n747 = case shown="True" w1667 {
                  tunnel: w1666 -> [w1669 w1674]
                  tunnel: w1665 -> [w1668 w1673]
                  tunnel: [w1669 w1672] -> w1663
                  tunnel: [w1668 w1671] -> w1662
                  frame False {
                    n748 = One Button Dialog(message="Please Acquire Image First") -> ()  [unwired: 1 in, 1 out]
                  }
                  frame True {
                    n749 = property on="Vision_Image" class="ImageControl"() -> ("ROI"=w1677:T48)  [unwired: 2 in, 2 out]
                    n750 = Unbundle By Name(w1677) -> ("Contours"=w1678:T49)
                    n751 = Index Array(array=w1678) -> (element=w1675:T50)  [unwired: 1 in]
                    n752 = Array Size(array=w1678) -> (size(s)=w1679:i32)
                    n753 = Not Equal To 0?(x=w1679) -> (x != 0?=w1676:bool)
                    n754 = case shown="True" w1676 {
                      tunnel: w1675 -> [_ w1684]
                      tunnel: w1674 -> [w1681 w1683]
                      tunnel: w1673 -> [w1680 w1682]
                      tunnel: [w1681 w1683] -> w1672
                      tunnel: [w1680 w1682] -> w1671
                      frame False {
                      }
                      frame True {
                        n755 = call "[FGV] ROI_List.vi"("Action"=ROI_List_Action."Add ROI", "ROI_To_Add"=w1684) -> ("error out"=w1685:errorcluster)  [unwired: 7 in, 2 out]
                        n756 = invoke on="Vision_Image" class="ImageControl" method="Clear ROI"(error in=w1685) -> ()  [unwired: 2 in, 3 out]
                      }
                    }
                  }
                }
              }
              frame "RemoveROI" {
                n757 = property on="ROI List" class="LstBox (strict)"(error in=w1698) -> (error out=w1697:errorcluster, "Item Names"=w1700:string[])  [unwired: 1 in, 1 out]
                n758 = property on="ROI List" class="LstBox (strict)"() -> ("Value"=w1701:i32[])  [unwired: 2 in, 2 out]
                n759 = property on="RootPath" class="Path"() -> ("Value"=w1690:path)  [unwired: 2 in, 2 out]
                n760 = property on="SEQ_Name" class="Ring (strict)"() -> ("Strings []"=w1689:string[], "Value"=w1687:u16)  [unwired: 2 in, 2 out]
                n761 = Index Array(array=w1701) -> (element=w1699:i32)  [unwired: 1 in]
                n762 = invoke on="Vision_Image" class="ImageControl" method="Clear ROI"(error in=w1697) -> (error out=w1696:errorcluster)  [unwired: 2 in, 2 out]
                n763 = Index Array(array=w1700, index=w1699) -> (element=w1688:string)
                n764 = disable-structure shown="Enabled" {
                  disable-tunnel: w1696 -> [w1711 w1714]
                  disable-tunnel: [w1709 w1717] -> w1691
                  disable-tunnel: w1690 -> [w1708 w1716]
                  disable-tunnel: w1689 -> [w1707 w1715]
                  disable-tunnel: w1688 -> [w1706 w1713]
                  disable-tunnel: w1687 -> [w1705 w1712]
                  frame Disabled {
                    n765 = call "Change DataFolders File Name_PM.vi"("error in (no error)"=w1711, "Value"=w1708, "ROI Name"=w1706, "Value 2"=w1705, "Strings []"=w1707) -> ("error out"=w1710:errorcluster)  [unwired: 6 in]
                    n766 = call <vilib>:"Clear Errors.vi"("error in (no error)"=w1710) -> ("error out"=w1704:errorcluster)  [unwired: 5 in, 1 out]
                    n767 = call "Change DataFolders File Name_CM.vi"("error in (no error)"=w1704, "Value"=w1708, "ROI Name"=w1706, "Value 2"=w1705, "Strings []"=w1707) -> ("error out"=w1709:errorcluster)  [unwired: 6 in]
                  }
                  frame Enabled {
                    n768 = call "Template Rename.vi"("ROI"=w1713, "Root Path"=w1716, "error in (no error)"=w1714, "Project List Idx"=w1712, "Project List"=w1715) -> ("error out"=w1717:errorcluster)  [unwired: 6 in]
                  }
                }
                n769 = property on="ROI List" class="LstBox (strict)"(error in=w1691) -> (error out=w1693:errorcluster, "Value"=w1694:i32[])  [unwired: 1 in, 1 out]
                n770 = call "[FGV] ROI_List.vi"("Action"=ROI_List_Action."Delete ROI", "error in (no error)"=w1693, "ROIs_Index"=w1694) -> ("error out"=w1692:errorcluster)  [unwired: 6 in, 2 out]
              }
            }
            n771 = local read "Auto Loading ROI Setting"() -> (w1641:bool)
            n772 = case shown="False" w1641 {
              tunnel: [w1653 w1654] -> w1640
              frame False {
                w1653 = T5[] [enum."UpdateROIListbox", enum."UpdateUIOverlay", enum."UpdateProcess", enum."UpdateAnalysis", enum."UpdateResultTable", enum."UpdateSelecedOutput", enum."Init Read Template"] items=["Init Setting", "Get Root Path", "Exit", "ActivateAllControls", "UpdateROIListbox", "UpdateSelectROIOverlay", "UpdateUIOverlay", "UpdateSelectedOverlay", "ConfigAnalysis", "ConfigProcess", "UpdateExistProjNames", "Init Result Page", "UpdateResultTable", "Init Menu", "Activate Menu", "UpdateProcess", "UpdateAnalysis", "SingleRun", "UpdateSelecedOutput", "ReloadResultTable", "SingleRunWithoutCaliper", "AddNewSeq", "UpdateCaliper", "SaveVisionSEQ", "Init User Parameter", "Cont.Run", "CalRotateImage", "Idle", "UpdateInitStatus", "Initilaize Camera", "Init Read Template", ""]
              }
              frame True {
                w1654 = T5[] [enum."UpdateROIListbox", enum."UpdateUIOverlay", enum."UpdateResultTable", enum."UpdateSelecedOutput", enum."Init Read Template"] items=["Init Setting", "Get Root Path", "Exit", "ActivateAllControls", "UpdateROIListbox", "UpdateSelectROIOverlay", "UpdateUIOverlay", "UpdateSelectedOverlay", "ConfigAnalysis", "ConfigProcess", "UpdateExistProjNames", "Init Result Page", "UpdateResultTable", "Init Menu", "Activate Menu", "UpdateProcess", "UpdateAnalysis", "SingleRun", "UpdateSelecedOutput", "ReloadResultTable", "SingleRunWithoutCaliper", "AddNewSeq", "UpdateCaliper", "SaveVisionSEQ", "Init User Parameter", "Cont.Run", "CalRotateImage", "Idle", "UpdateInitStatus", "Initilaize Camera", "Init Read Template", ""]
              }
            }
            n773 = for {
              tunnel: w1644 -> [w1658]
              tunnel: w1643 -> [w1657]
              tunnel: w1640 -> [w1656] mode=indexing
              tunnel: [w1655] -> _
              n774 = Enqueue Element(queue=w1658, element=w1656, error in (no error)=w1657) -> (error out=w1655:errorcluster)  [unwired: 1 in, 2 out]
            }
          }
          event "CameraName": Value Change {
            n775 = event-data() -> ("NewVal"=w1720:u16)  [unwired: 1 in, 5 out]
            n776 = control-ref of="CameraName"() -> (w1721:refnum<vi>)
            n777 = call "Camera_SetCameraRing.vi"("Camera Index"=w1720, "CameraName"=w1721) -> ()  [unwired: 9 in, 1 out]
          }
          event "ContRun": Value Change {
            w1728 = T5[] [enum."Cont.Run"] items=["Init Setting", "Get Root Path", "Exit", "ActivateAllControls", "UpdateROIListbox", "UpdateSelectROIOverlay", "UpdateUIOverlay", "UpdateSelectedOverlay", "ConfigAnalysis", "ConfigProcess", "UpdateExistProjNames", "Init Result Page", "UpdateResultTable", "Init Menu", "Activate Menu", "UpdateProcess", "UpdateAnalysis", "SingleRun", "UpdateSelecedOutput", "ReloadResultTable", "SingleRunWithoutCaliper", "AddNewSeq", "UpdateCaliper", "SaveVisionSEQ", "Init User Parameter", "Cont.Run", "CalRotateImage", "Idle", "UpdateInitStatus", "Initilaize Camera", "Init Read Template", ""]
            n778 = control-ref of="Main_Tab"() -> (w1722:refnum<vi>)
            n779 = event-data() -> ("NewVal"=w1723:bool)  [unwired: 1 in]
            n780 = case shown="False" w1723 {
              tunnel: w1727 -> [w1734 w1754]
              tunnel: w1726 -> [w1733 w1753]
              tunnel: [w1734 w1754] -> w1725
              tunnel: [w1733 w1753] -> w1724
              tunnel: w1722 -> [w1731 w1751]
              frame True {
                n781 = property class="TabCtl (strict)"(reference=w1731) -> ("Pages"=w1732:refnum<vi>[])  [unwired: 1 in, 2 out]
                n782 = for {
                  tunnel: w1732 -> [w1737] mode=indexing
                  n783 = property class="Page"(reference=w1737) -> ("ControlsOnPage"=w1736:refnum<vi>[])  [unwired: 1 in, 2 out]
                  n784 = for {
                    tunnel: w1736 -> [w1746] mode=indexing
                    tunnel: [w1738] -> w1735
                    w1738 = T8."Disabled and Grayed Out" ("Disabled")
                    n785 = property class="Ctl"(reference=w1746) -> (reference out=w1744:refnum<vi>, "Label.Text"=w1743:string)  [unwired: 1 in, 1 out]
                    n786 = Equal?(x=w1743, y="Vision_Image") -> (x = y?=w1742:bool)
                    n787 = Equal?(x=w1743, y="ContRun") -> (x = y?=w1741:bool)
                    n788 = Or(x=w1742, y=w1741) -> (x .or. y?=w1740:bool)
                    n789 = case shown="False" w1740 {
                      tunnel: w1744 -> [w1748 w1750]
                      tunnel: w1738 -> [w1747 _]
                      frame False {
                        n790 = property class="Ctl"(reference=w1748, "DisabledEnum"=w1747) -> ()  [unwired: 1 in, 2 out]
                      }
                      frame True {
                        n791 = property class="Ctl"(reference=w1750, "DisabledEnum"=T8."Enabled" ("Disabled")) -> ()  [unwired: 1 in, 2 out]
                      }
                    }
                  }
                  n792 = property on="NewVisionSEQ" class="Bool"("DisabledEnum"=w1735) -> ()  [unwired: 2 in, 2 out]
                  n793 = property on="ExitVisionEditor" class="Bool"("DisabledEnum"=w1735) -> ()  [unwired: 2 in, 2 out]
                  n794 = property on="Vision_SEQ_Name" class="Enum (strict)"("DisabledEnum"=w1735) -> ()  [unwired: 2 in, 2 out]
                  n795 = property on="SaveVisionSEQ" class="Bool"("DisabledEnum"=w1735) -> ()  [unwired: 2 in, 2 out]
                  n796 = property on="DeleteVisionSEQ" class="Bool"("DisabledEnum"=w1735) -> ()  [unwired: 2 in, 2 out]
                  n797 = property on="SEQ_Name" class="Ring (strict)"("DisabledEnum"=w1735) -> ()  [unwired: 2 in, 2 out]
                }
              }
              frame False {
                n798 = property class="TabCtl (strict)"(reference=w1751) -> ("Pages"=w1752:refnum<vi>[])  [unwired: 1 in, 2 out]
                n799 = for {
                  tunnel: w1752 -> [w1757] mode=indexing
                  n800 = property class="Page"(reference=w1757) -> ("ControlsOnPage"=w1756:refnum<vi>[])  [unwired: 1 in, 2 out]
                  n801 = for {
                    tunnel: w1756 -> [w1766] mode=indexing
                    tunnel: [w1758] -> w1755
                    w1758 = T8."Enabled" ("Disabled")
                    n802 = property class="Ctl"(reference=w1766) -> (reference out=w1764:refnum<vi>, "Label.Text"=w1763:string)  [unwired: 1 in, 1 out]
                    n803 = Equal?(x=w1763, y="Vision_Image") -> (x = y?=w1762:bool)
                    n804 = Equal?(x=w1763, y="ContRun") -> (x = y?=w1761:bool)
                    n805 = Or(x=w1762, y=w1761) -> (x .or. y?=w1760:bool)
                    n806 = case shown="False" w1760 {
                      tunnel: w1764 -> [w1768 w1770]
                      tunnel: w1758 -> [w1767 _]
                      frame False {
                        n807 = property class="Ctl"(reference=w1768, "DisabledEnum"=w1767) -> ()  [unwired: 1 in, 2 out]
                      }
                      frame True {
                        n808 = property class="Ctl"(reference=w1770, "DisabledEnum"=T8."Enabled" ("Disabled")) -> ()  [unwired: 1 in, 2 out]
                      }
                    }
                  }
                  n809 = property on="NewVisionSEQ" class="Bool"("DisabledEnum"=w1755) -> ()  [unwired: 2 in, 2 out]
                  n810 = property on="ExitVisionEditor" class="Bool"("DisabledEnum"=w1755) -> ()  [unwired: 2 in, 2 out]
                  n811 = property on="Vision_SEQ_Name" class="Enum (strict)"("DisabledEnum"=w1755) -> ()  [unwired: 2 in, 2 out]
                  n812 = property on="SEQ_Name" class="Ring (strict)"("DisabledEnum"=w1755) -> ()  [unwired: 2 in, 2 out]
                  n813 = property on="DeleteVisionSEQ" class="Bool"("DisabledEnum"=w1755) -> ()  [unwired: 2 in, 2 out]
                  n814 = property on="SaveVisionSEQ" class="Bool"("DisabledEnum"=w1755) -> ()  [unwired: 2 in, 2 out]
                }
              }
            }
            n815 = for {
              tunnel: w1725 -> [w1775]
              tunnel: w1728 -> [w1774] mode=indexing
              tunnel: w1724 -> [w1773]
              tunnel: [w1772] -> _
              tunnel: [w1771] -> _
              n816 = Enqueue Element(queue=w1775, element=w1774, error in (no error)=w1773) -> (queue out=w1772:refnum<queue>, error out=w1771:errorcluster)  [unwired: 1 in, 1 out]
            }
          }
          event User Event {
            n817 = event-data() -> ()  [unwired: 1 in, 1 out]
            n818 = property on="File Path" class="Path"() -> ("Visible"=w1780:bool)  [unwired: 2 in, 2 out]
            n819 = case shown="True" w1780 {
              tunnel: [w1797 w1827] -> w1776
              tunnel: [w1798 w1822] -> w1779
              frame False {
                n820 = control-ref of="CameraName"() -> (w1796:refnum<vi>)
                n821 = call "Camera_CheckCameraSetting.vi"("CameraName"=w1796) -> ("CameraGot?"=w1800:bool, "Camera Session"=w1799:T47)  [unwired: 9 in]
                n822 = case shown="True" w1800 {
                  tunnel: [T3 refnum ("New Image") w1804] -> w1797
                  tunnel: w1799 -> [_ _]
                  tunnel: [errorcluster {"status"=TRUE, "code"=0, "source"=""} ("error out") w1803] -> w1798
                  frame False {
                  }
                  frame True {
                    n823 = call "IMAQ Create"("Image Name"="Snap") -> ("New Image"=w1805:T3)  [unwired: 3 in, 2 out]
                    n824 = disable-structure shown="Disabled" {
                      disable-tunnel: w1805 -> [w1809 w1820]
                      disable-tunnel: [w1808 w1819] -> w1804
                      disable-tunnel: [w1807 w1818] -> w1803
                      frame Disabled {
                        n825 = disable-structure shown="Enabled" {
                          disable-tunnel: [w1813 w1817] -> w1807
                          disable-tunnel: w1809 -> [w1812 w1815]
                          disable-tunnel: [w1811 w1816] -> w1808
                          disable-tunnel: _ -> [w1810 w1814]
                          frame Disabled {
                            n826 = call "Camera_Snap.vi"("Camera Session In"=w1810, "Image In"=w1812) -> ("error out"=w1813:errorcluster, "New Image"=w1811:T3)  [unwired: 8 in]
                          }
                          frame Enabled {
                            n827 = call "Camera_Snap_Jesse.vi"("Camera Session In"=w1814, "Image In"=w1815) -> ("error out"=w1817:errorcluster, "New Image"=w1816:T3)  [unwired: 8 in]
                          }
                        }
                      }
                      frame Enabled {
                        n828 = call "[FGV] Camera Settings.vi"("Action"=T13."Grab", "Image In"=w1820) -> ("error out"=w1818:errorcluster, "Image Out"=w1819:T3)  [unwired: 7 in, 1 out]
                      }
                    }
                  }
                }
              }
              frame True {
                n829 = local read "CycleThruFolder"() -> (w1823:bool)
                n830 = case shown="True" w1823 {
                  tunnel: [w1828 w1830] -> w1826
                  frame False {
                    n831 = local read "File Path"() -> (w1828:path)
                  }
                  frame True {
                    n832 = control-ref of="Folder Image Files"() -> (w1829:refnum<vi>)
                    n833 = call "ImageFile_GetFolderImageAndRotate.vi"("Folder Image Files"=w1829) -> ("File Path"=w1830:path)  [unwired: 9 in, 1 out]
                  }
                }
                n834 = call <vilib>:"Check if File or Folder Exists.vi"("path"=w1826) -> ("file or folder exists?"=w1825:bool, "dup path"=w1824:path)  [unwired: 8 in, 1 out]
                n835 = case shown="True" w1825 {
                  tunnel: [T3 refnum ("New Image") w1835] -> w1827
                  tunnel: w1824 -> [_ w1834]
                  tunnel: [errorcluster {"status"=TRUE, "code"=0, "source"=""} ("error out") w1833] -> w1822
                  frame False {
                  }
                  frame True {
                    n836 = call "IMAQ GetFileInfo"("File Path"=w1834) -> ("Image Type"=w1837:T32)  [unwired: 4 in, 6 out]
                    n837 = call "IMAQ Create"("Image Name"="Snap", "Image Type"=w1837) -> ("New Image"=w1836:T3)  [unwired: 2 in, 2 out]
                    n838 = call "ImageFile_GetSingleImage.vi"("File Path"=w1834, "Image In"=w1836) -> ("error out"=w1833:errorcluster, "New Image"=w1835:T3)  [unwired: 8 in]
                  }
                }
              }
            }
            n839 = case shown="No Error" w1779 {
              tunnel: w1778 -> [w1784 _]
              frame No Error {
                w1783 = T5[] [enum."CalRotateImage", enum."SingleRun"] items=["Init Setting", "Get Root Path", "Exit", "ActivateAllControls", "UpdateROIListbox", "UpdateSelectROIOverlay", "UpdateUIOverlay", "UpdateSelectedOverlay", "ConfigAnalysis", "ConfigProcess", "UpdateExistProjNames", "Init Result Page", "UpdateResultTable", "Init Menu", "Activate Menu", "UpdateProcess", "UpdateAnalysis", "SingleRun", "UpdateSelecedOutput", "ReloadResultTable", "SingleRunWithoutCaliper", "AddNewSeq", "UpdateCaliper", "SaveVisionSEQ", "Init User Parameter", "Cont.Run", "CalRotateImage", "Idle", "UpdateInitStatus", "Initilaize Camera", "Init Read Template", ""]
                w1785 = T5[] [enum."UpdateSelecedOutput", enum."Cont.Run"] items=["Init Setting", "Get Root Path", "Exit", "ActivateAllControls", "UpdateROIListbox", "UpdateSelectROIOverlay", "UpdateUIOverlay", "UpdateSelectedOverlay", "ConfigAnalysis", "ConfigProcess", "UpdateExistProjNames", "Init Result Page", "UpdateResultTable", "Init Menu", "Activate Menu", "UpdateProcess", "UpdateAnalysis", "SingleRun", "UpdateSelecedOutput", "ReloadResultTable", "SingleRunWithoutCaliper", "AddNewSeq", "UpdateCaliper", "SaveVisionSEQ", "Init User Parameter", "Cont.Run", "CalRotateImage", "Idle", "UpdateInitStatus", "Initilaize Camera", "Init Read Template", ""]
                n840 = for {
                  tunnel: w1784 -> [w1795]
                  tunnel: w1783 -> [w1794] mode=indexing
                  tunnel: [w1793] -> w1787
                  tunnel: [w1792] -> w1781
                  n841 = Enqueue Element(queue=w1795, element=w1794) -> (queue out=w1792:refnum<queue>, error out=w1793:errorcluster)  [unwired: 2 in, 1 out]
                }
                n842 = call "Time Delay2"("error in (no error)"=w1787, "Delay Time (s)"=1.0) -> ("error out"=w1782:errorcluster)  [unwired: 9 in]
                n843 = for {
                  tunnel: w1781 -> [w1791]
                  tunnel: w1785 -> [w1790] mode=indexing
                  tunnel: [w1789] -> _
                  tunnel: w1782 -> [w1788]
                  n844 = Enqueue Element(queue=w1791, element=w1790, error in (no error)=w1788) -> (error out=w1789:errorcluster)  [unwired: 1 in, 2 out]
                }
              }
              frame Error {
              }
            }
          }
          event "DeleteVisionSEQ": Value Change {
            n845 = event-data() -> ()  [unwired: 1 in, 1 out]
            n846 = Two Button Dialog(message="Do You Want Delet File?", 1:"No" ("F button name (\"Cancel\")"), 2:"Yes" ("T button name (\"OK\")")) -> (T button?=w1846:bool)
            n847 = case shown="True" w1846 {
              tunnel: w1842 -> [_ w1851]
              tunnel: w1841 -> [_ _]
              tunnel: w1840 -> [w1848 w1850]
              tunnel: [w1848 w1850] -> w1839
              frame False {
              }
              frame True {
                w1852 = T5[] [enum."UpdateExistProjNames", enum."Init User Parameter", enum."UpdateROIListbox"] items=["Init Setting", "Get Root Path", "Exit", "ActivateAllControls", "UpdateROIListbox", "UpdateSelectROIOverlay", "UpdateUIOverlay", "UpdateSelectedOverlay", "ConfigAnalysis", "ConfigProcess", "UpdateExistProjNames", "Init Result Page", "UpdateResultTable", "Init Menu", "Activate Menu", "UpdateProcess", "UpdateAnalysis", "SingleRun", "UpdateSelecedOutput", "ReloadResultTable", "SingleRunWithoutCaliper", "AddNewSeq", "UpdateCaliper", "SaveVisionSEQ", "Init User Parameter", "Cont.Run", "CalRotateImage", "Idle", "UpdateInitStatus", "Initilaize Camera", "Init Read Template", ""]
                n848 = property on="SEQ_Name" class="Ring (strict)"() -> ("Strings []"=w1854:string[], "Value"=w1855:u16)  [unwired: 2 in, 2 out]
                n849 = Delete From Array(array=w1854, index=w1855) -> (array with subset deleted=w1861:string[])  [unwired: 1 in, 1 out]
                n850 = Index Array(array=w1854, index=w1855) -> (element=w1859:string)
                n851 = property on="RootPath" class="Path"() -> ("Value"=w1856:path)  [unwired: 2 in, 2 out]
                n852 = property on="SEQ_Name" class="Ring (strict)"("Strings []"=w1861, "Value"=0) -> ()  [unwired: 2 in, 2 out]
                n853 = Build Path(base path=w1856, name or relative path="data") -> (appended path=w1858:path)
                n854 = Build Path(base path=w1858, name or relative path=w1859) -> (appended path=w1860:path)
                n855 = call "[FGV]Button Click Frequency.vi"("Command"=enum16{"Initialize", "Add", "Read"}."Initialize") -> ()  [unwired: 9 in, 2 out]
                n856 = Delete(path (use dialog)=w1860, entire hierarchy (F)=TRUE) -> (error out=w1849:errorcluster)  [unwired: 3 in, 2 out]
                n857 = for {
                  tunnel: w1852 -> [w1866] mode=indexing
                  tunnel: w1851 -> [w1865]
                  tunnel: w1849 -> [w1864]
                  n858 = Enqueue Element(queue=w1865, element=w1866, error in (no error)=w1864) -> ()  [unwired: 1 in, 3 out]
                }
              }
            }
          }
        }
      }
    }
    frame Enabled {
    }
  }
  n859 = disable-structure shown="Disabled" {
    frame Disabled {
      n860 = case shown="False" "Auto Loading ROI Setting" {
        frame False {
          n861 = local write "Auto Loading ROI Setting"(TRUE) -> ()
        }
        frame True {
          n862 = local write "Auto Loading ROI Setting"(FALSE) -> ()
        }
      }
    }
    frame Enabled {
    }
  }
  n863 = call "IMAQ Dispose"("Image"=w19) -> ()  [unwired: 5 in, 1 out]
  n864 = Unregister For Events(event registration refnum=w12) -> ()  [unwired: 1 in, 1 out]
  n865 = Flush Queue(queue=w23) -> (queue out=w22:refnum<queue>, error out=w21:errorcluster)  [unwired: 1 in, 1 out]
  n866 = Destroy User Event(user event=w13) -> ()  [unwired: 1 in, 1 out]
  n867 = Release Queue(queue=w22, error in (no error)=w21) -> ()  [unwired: 1 in, 3 out]
